vi "高压板校准程序1.2.vi"(8 "波特率":T3(ring)=enum."500Kbps", 9 "CAN路数":u16(ring) items=["0", "1"], 10 "设备索引":u16(ring) items=["0", "1", "2", "3", "4", "5", "6", "7", "8", "9", "10", "11", "12", "13", "14", "15", ""], 11 "CAN卡类型":u32(ring)=21 items=["PCI5121"=1, "PCI9810"=2, "USBCAN1"=3, "USBCAN2"=4, "PCI9820"=5, "PCI5110"=7, "CANLite(mini)"=8, "ISA9620"=9, "ISA5420"=10, "PC104CAN"=11, "DNP9810"=13, "PCI9840B"=14, "PC104C2"=15, "PCI9820I"=16, "pec9920"=18, "USBCAN_E_U"=20, "USBCAN_2E_U"=21]) -> (6 "E-U_baud":u32(ring)=393223 items=["0x060003--1000Kbps"=393219, "0x060004--800Kbps"=393220, "0x060007--500Kbps"=393223, "0x1C0008--250Kbps"=1835016, "0x1C0011--125Kbps"=1835025, "0x160023--100Kbps"=1441827, "0x1C002C--50Kbps"=1835052, "0x1600B3--20Kbps"=1441971, "0x1C00E0--10Kbps"=1835232, "0x1C01C1--5Kbps"=1835457])   [LabVIEW 2013]
uses:
  <vilib>/Instr/_visa.llb/VISA Configure Serial Port (Instr).vi
  <vilib>/Utility/config.llb/Write Key (String).vi
  <vilib>/Utility/file.llb/Read From Spreadsheet File (string).vi
  <vilib>/Utility/file.llb/Write To Spreadsheet File (string).vi
  <vilib>/Utility/config.llb/NI_LVConfig.lvlib
  data/kerneldlls/usbcan.dll
panel:
  out "输出3":dbl
  in  "输出簇":T1
  out "Life":dbl
  out "分流器":enum32{"选项卡 1"}(tab)
  out "外总压":enum32{"选项卡 1"}(tab)
  out "内总压":enum32{"选项卡 1"}(tab)
  out "电流校正 2":enum32{"选项卡 1"}(tab)
  out "电流校正":enum32{"选项卡 1"}(tab)
  in  "Judge(%)":dbl=1.0
  in  "Judge(%)":dbl=0.5
  in  "记录":bool
  out "结果":i32(listbox)=-1
  in  "一键校正":bool
  in  "刷新":bool
  in  "分流器大小":T2(ring)=enum."300A"
  out "监控状态":bool
  out "Curr":dbl format="%#.6f"
  out "SumV_out":dbl format="%#.6f"
  out "SumV_in":dbl format="%#.6f"
  in  "平均电压":dbl
  in  "电压增益":dbl
  in  "平均电流":dbl
  in  "电流增益":dbl
  in  "放电能量阀值":dbl=375.0
  in  "充电能量阀值":dbl=375.0
  in  "分流器型号":bool
  out "Current Gain结果 4":bool
  in  "充电能量阀值":bool
  out "Current Offset结果 4":bool
  in  "Set Current Gain 3":bool
  out "Current Gain结果 3":bool
  in  "Set Current Offset 3":bool
  out "Current Offset结果 3":bool
  out "Shunt Volt Gain":string
  out "Shunt Volt Offset":string
  in  "Set Current Gain 2":bool
  out "Current Gain结果 2":bool
  in  "Volt Offset":bool
  out "Current Offset结果 2":bool
  in  "导入配置结果":bool
  in  "读版本结果":bool
  in  "写版本结果":bool
  out "版本号-读":string
  in  "版本号":string
  in  "写配置文件版本":bool
  in  "读配置文件版本":bool
  in  "生成配置":bool
  in  "导入配置":bool
  out "config_data":string="000124FE00264205"
  out "充放电阈值":dbl=75006.0
  in  "连接状态 10":bool
  in  "设置参数":bool
  in  "安时分辨率/AH":u16(ring)=1 items=["0.001", "0.2"]
  in  "是否有外部高压":u16(ring)=1 items=["有", "无"]
  in  "分流器大小/A":u16(ring)=3 items=["50", "100", "200", "300", "400", "500", "600", "700", "800", "900", "1000"]
  in  "传感器类型":u16(ring)=1 items=["霍尔传感器", "分流器"]
  in  "电压分辨率/V":u16(ring)=1 items=["0.01", "0.1"]
  in  "电流分辨率/A":u16(ring)=1 items=["0.01", "0.1"]
  in  "Set":dbl
  in  "Volt2":dbl=300.0
  in  "Volt1":dbl=150.0
  in  "Clear":bool
  out "Clear结果":bool
  out "电流增益":string
  out "电流零点":string
  in  "Read1_in":bool
  out "Read1_in结果":bool
  in  "REAL1":dbl=150.0
  out "AD1":dbl
  in  "REAL2":dbl=300.0
  out "AD2":dbl
  in  "Offset":i32 format="%x"
  in  "Gain":dbl
  in  "REAL1":dbl=150.0
  in  "AD1":dbl
  in  "REAL2":dbl=300.0
  in  "AD2":dbl
  in  "Offset":i32 format="%x"
  in  "Gain":dbl
  in  "Read2_in":bool
  out "Read2_in结果":bool
  in  "Set_in":bool
  out "Set_in结果":bool
  in  "Read1_Out":bool
  out "Read1_Out结果":bool
  in  "Read2_Out":bool
  out "Read2_Out结果":bool
  in  "Set_out":bool
  out "Set_out结果":bool
  in  "Read1":bool
  out "Read1结果":bool
  in  "REAL1":dbl=40.0
  out "AD1":u16
  in  "REAL2":dbl=80.0
  out "AD2":u16
  in  "Gain":dbl
  in  "Read2":bool
  out "Read2结果":bool
  in  "Set":bool
  out "Set结果":bool
  in  "Set Current Gain":bool
  out "Current Gain结果":bool
  in  "Set Current Offset":bool
  out "Current Offset结果":bool
  in  "Clear_out":bool
  out "Clear_out结果":bool
  in  "Clear_in":bool
  out "Clear_in结果":bool
  in  "输出自定义值1":bool
  in  "输出自定义值2":bool
  out "Actual":dbl format="%#.6f"
  out "Set":dbl format="%#.6f"
  out "Actual":dbl
  in  "连接电压源":bool
  out "连接状态 10":bool
  in  "VISA resource name 4":refnum<visa-resource-name>="COM1" caption="设备端口号"
  in  "工作方式":u8(ring) items=["Normal", "Listen Only"]
  in  "滤波方式":u8(ring) items=["Dual Filter", "Single Filter"]
  out "CAN连接状态":bool
  in  "启动CAN连接":bool
  in  "VISA resource name 2":refnum<visa-resource-name>="GPIB0::5::INSTR" caption="设备端口号"
  out "连接状态 10":bool
  in  "连接GPIB":bool
  in  "Curr1":dbl=40.0
  in  "输出自定义值1 2":bool
  in  "输出自定义值2 2":bool
  in  "Curr2":dbl=80.0
  in  "退出":bool
  out "设置中？ 2":bool
  out "CAN状态 3":bool
  in  "设备索引 3":u16(ring) items=["0", "1", "2", "3", "4", "5", "6", "7", "8", "9", "10", "11", "12", "13", "14", "15", ""]
  in  "CAN路数 3":u16(ring) items=["0", "1"]
  in  "设备类型 3":u16(ring)=4 items=["PCI5121"=1, "PCI9810"=2, "USBCAN1"=3, "USBCAN2"=4, "PCI9820"=5, "CAN232"=6, "PCI5110"=7, "CANLite(mini)"=8, "ISA9620"=9, "ISA5420"=10, "PC104CAN"=11, "CANETE"=12, "DNP9810"=13]
  out "CAN 3":bool
  in  "停止 2":bool=TRUE
  out "监控 4":bool
  out "x-y":u32
  in  "退出程序 2":bool
  in  "error in (no error)":errorcluster caption="错误输入（无错误）"
  in  "控制读取  2":bool
  out "VISA资源名称输出":refnum<visa-resource-name>="0"
  in  "退出程序 3":bool
  in  "输出200A":bool
  out "实际值 2":dbl
  out "设定值 2":dbl
  in  "输出100A":bool
  in  "停止 7":bool=TRUE
  in  "分辨率偏移值 4":T4={"主板总电压分辨率"=0.01, "主板总电压偏移量"=0.0, "主板总电流分辨率"=0.01, "主板总电流偏移量"=-300.0, "主板安时分辨率"=0.2, "主板安时偏移量"=0.0, "主板SOC分辨率"=0.4, "主板SOC偏移量"=0.0, "从板总电压分辨率"=0.01, "从板总电压偏移量"=0.0, "从板总电流分辨率"=0.01, "从板总电流偏移量"=0.0, "从板安时分辨率"=0.2, "从板安时偏移量"=0.0, "从板SOC分辨率"=0.4, "从板SOC偏移量"=0.0, "功率分辨率"=0.01, "功率偏移量"=-300.0, "单体电压分辨率 "=0.0001, "单体电压偏移量"=0.0, "温度分辨率"=1.0, "温度偏移量"=-40.0, "高压板总电压分辨率"=0.01, "高压板总电压偏移量"=0.0, "高压板总电流分辨率"=0.01, "高压板总电流偏移量"=-300.0, "高压板安时分辨率"=0.2, "高压板安时偏移量"=0.0, "高压板SOC分辨率"=0.4, "高压板SOC偏移量"=0.0, "高压板功率分辨率"=0.01, "高压板功率偏移量"=-300.0}
  in  "分辨率偏移值 3":T4={"主板总电压分辨率"=0.01, "主板总电压偏移量"=0.0, "主板总电流分辨率"=0.01, "主板总电流偏移量"=-300.0, "主板安时分辨率"=0.2, "主板安时偏移量"=0.0, "主板SOC分辨率"=0.4, "主板SOC偏移量"=0.0, "从板总电压分辨率"=0.01, "从板总电压偏移量"=0.0, "从板总电流分辨率"=0.01, "从板总电流偏移量"=0.0, "从板安时分辨率"=0.2, "从板安时偏移量"=0.0, "从板SOC分辨率"=0.4, "从板SOC偏移量"=0.0, "功率分辨率"=0.01, "功率偏移量"=-300.0, "单体电压分辨率 "=0.0001, "单体电压偏移量"=0.0, "温度分辨率"=1.0, "温度偏移量"=-40.0, "高压板总电压分辨率"=0.01, "高压板总电压偏移量"=0.0, "高压板总电流分辨率"=0.01, "高压板总电流偏移量"=-300.0, "高压板安时分辨率"=0.2, "高压板安时偏移量"=0.0, "高压板SOC分辨率"=0.4, "高压板SOC偏移量"=0.0, "高压板功率分辨率"=0.01, "高压板功率偏移量"=-300.0}
  in  "监控":bool
  out "VCI_CAN_OBJ_R 2":T5={"ID"=0, "TimeStamp"=0, "TimeFlag"=0, "SendType"=1, "RemoteFlag"=0, "ExternFlag"=0, "DataLen"=8, 0, 0, 0, 0, 0, 0, 0, 0, 0, 0, 0}
  in  "分辨率偏移值":T6
  out "允许读取":bool
  out "设置中？":bool
  out "CAN状态 2":bool=TRUE
  in  "设备索引 2":u16(ring) items=["0", "1", "2", "3", "4", "5", "6", "7", "8", "9", "10", "11", "12", "13", "14", "15", ""]
  in  "CAN路数 2":u16(ring) items=["0", "1"]
  in  "设备类型 2":u16(ring)=4 items=["PCI5121"=1, "PCI9810"=2, "USBCAN1"=3, "USBCAN2"=4, "PCI9820"=5, "CAN232"=6, "PCI5110"=7, "CANLite(mini)"=8, "ISA9620"=9, "ISA5420"=10, "PC104CAN"=11, "CANETE"=12, "DNP9810"=13]
  out "CAN 2":bool
  in  "监控 2":bool
  in  "停止 6":bool=TRUE
  out "接收":T5={"ID"=67239966, "TimeStamp"=241409471, "TimeFlag"=1, "SendType"=250, "RemoteFlag"=0, "ExternFlag"=1, "DataLen"=8, 0, 0, 117, 48, 117, 48, 0, 0, 0, 0, 124} {"ID" format="%x"}
  in  "高压板信息":T7={"内部高压/V"=0.0, "Life"=10.0, "外部高压/V"=0.0, "power/KW"=0.0, "current/A"=0.0, "error code"=1, "SOC/%"=0.0, "总充电安时/AH"=0.0, "总放电安时/AH"=0.0, "平均电压"=0.0} {"平均电压" format="%.3f"; "总放电安时/AH" format="%#.3f"; "总充电安时/AH" format="%#.3f"; "SOC/%" format="%.3g"; "error code" format="%x"; "current/A" format="%.3g"; "power/KW" format="%#.3f"; "外部高压/V" format="%.3g"; "内部高压/V" format="%.3g"}
  in  "控制读取  5":bool
  out "VISA资源名称输出 10":refnum<visa-resource-name>
  in  "输出300V":bool
  out "电流/A 4":dbl
  in  "输出150V":bool
  in  "停止 3":bool=TRUE
  out "error out 3":errorcluster caption="error out"
  in  "错误输入（无错误）":errorcluster
  in  "控制读取  2":bool
  out "VISA资源名称输出 9":refnum<visa-resource-name>
  in  "退出程序":bool
  in  "输出80A":bool
  in  "输出40A":bool
  in  "控制读取  4":bool
  out "VISA资源名称输出 8":refnum<visa-resource-name>
  in  "连接状态 7":bool
  out "error out 2":errorcluster caption="error out"
  in  "控制读取  2":bool
  in  "连接状态 6":bool
  in  "控制读取  3":bool
  out "VISA资源名称输出 6":refnum<visa-resource-name>
  out "error out":errorcluster
  in  "控制读取  2":bool
  out "VISA资源名称输出 5":refnum<visa-resource-name>
  in  "电流值":dbl
  in  "自动控制仪器":bool=TRUE
  out "VISA资源名称输出 4":refnum<visa-resource-name>
  out "VISA资源名称输出 3":refnum<visa-resource-name>
  out "实际值 3":dbl format="%#.6f"
  out "设定值":dbl format="%#.6f"
  in  "控制读取  2":bool
  out "电流/A":dbl
  in  "控制读取":bool
  in  "Boar_Type":bool
  out "temp1":bool
  in  "总步骤":dbl=21.0
  in  "NG重测次数":dbl=3.0
  out "一键测试":bool
  out "测试结果":bool=TRUE
  in  "行号":dbl
  out "CAN状态":bool=TRUE
  out "CAN":bool
  in  "监控":bool=TRUE
  out "VCI_CAN_OBJ_R":T5={"ID"=0, "TimeStamp"=0, "TimeFlag"=0, "SendType"=1, "RemoteFlag"=0, "ExternFlag"=0, "DataLen"=8, 0, 0, 0, 0, 0, 0, 0, 0, 0, 0, 0}
  in  "停止":bool=TRUE
  # "重要参数设置"
  # "A"
  # "V"
  # "蓝微新源BMS_电压电流校准"
  # "内总压"
  # "电流增益"
  # "AD2=AD1*2"
  # "外总压"
  # "BMS_Monitor"
  # "分辩率"
  # "偏移量"
  # "分辩率"
  # "偏移量"
  # "分辩率"
  # "偏移量"
  # "分辩率"
  # "偏移量"
  # "分辩率"
  # "偏移量"
  # "分辩率"
  # "偏移量"
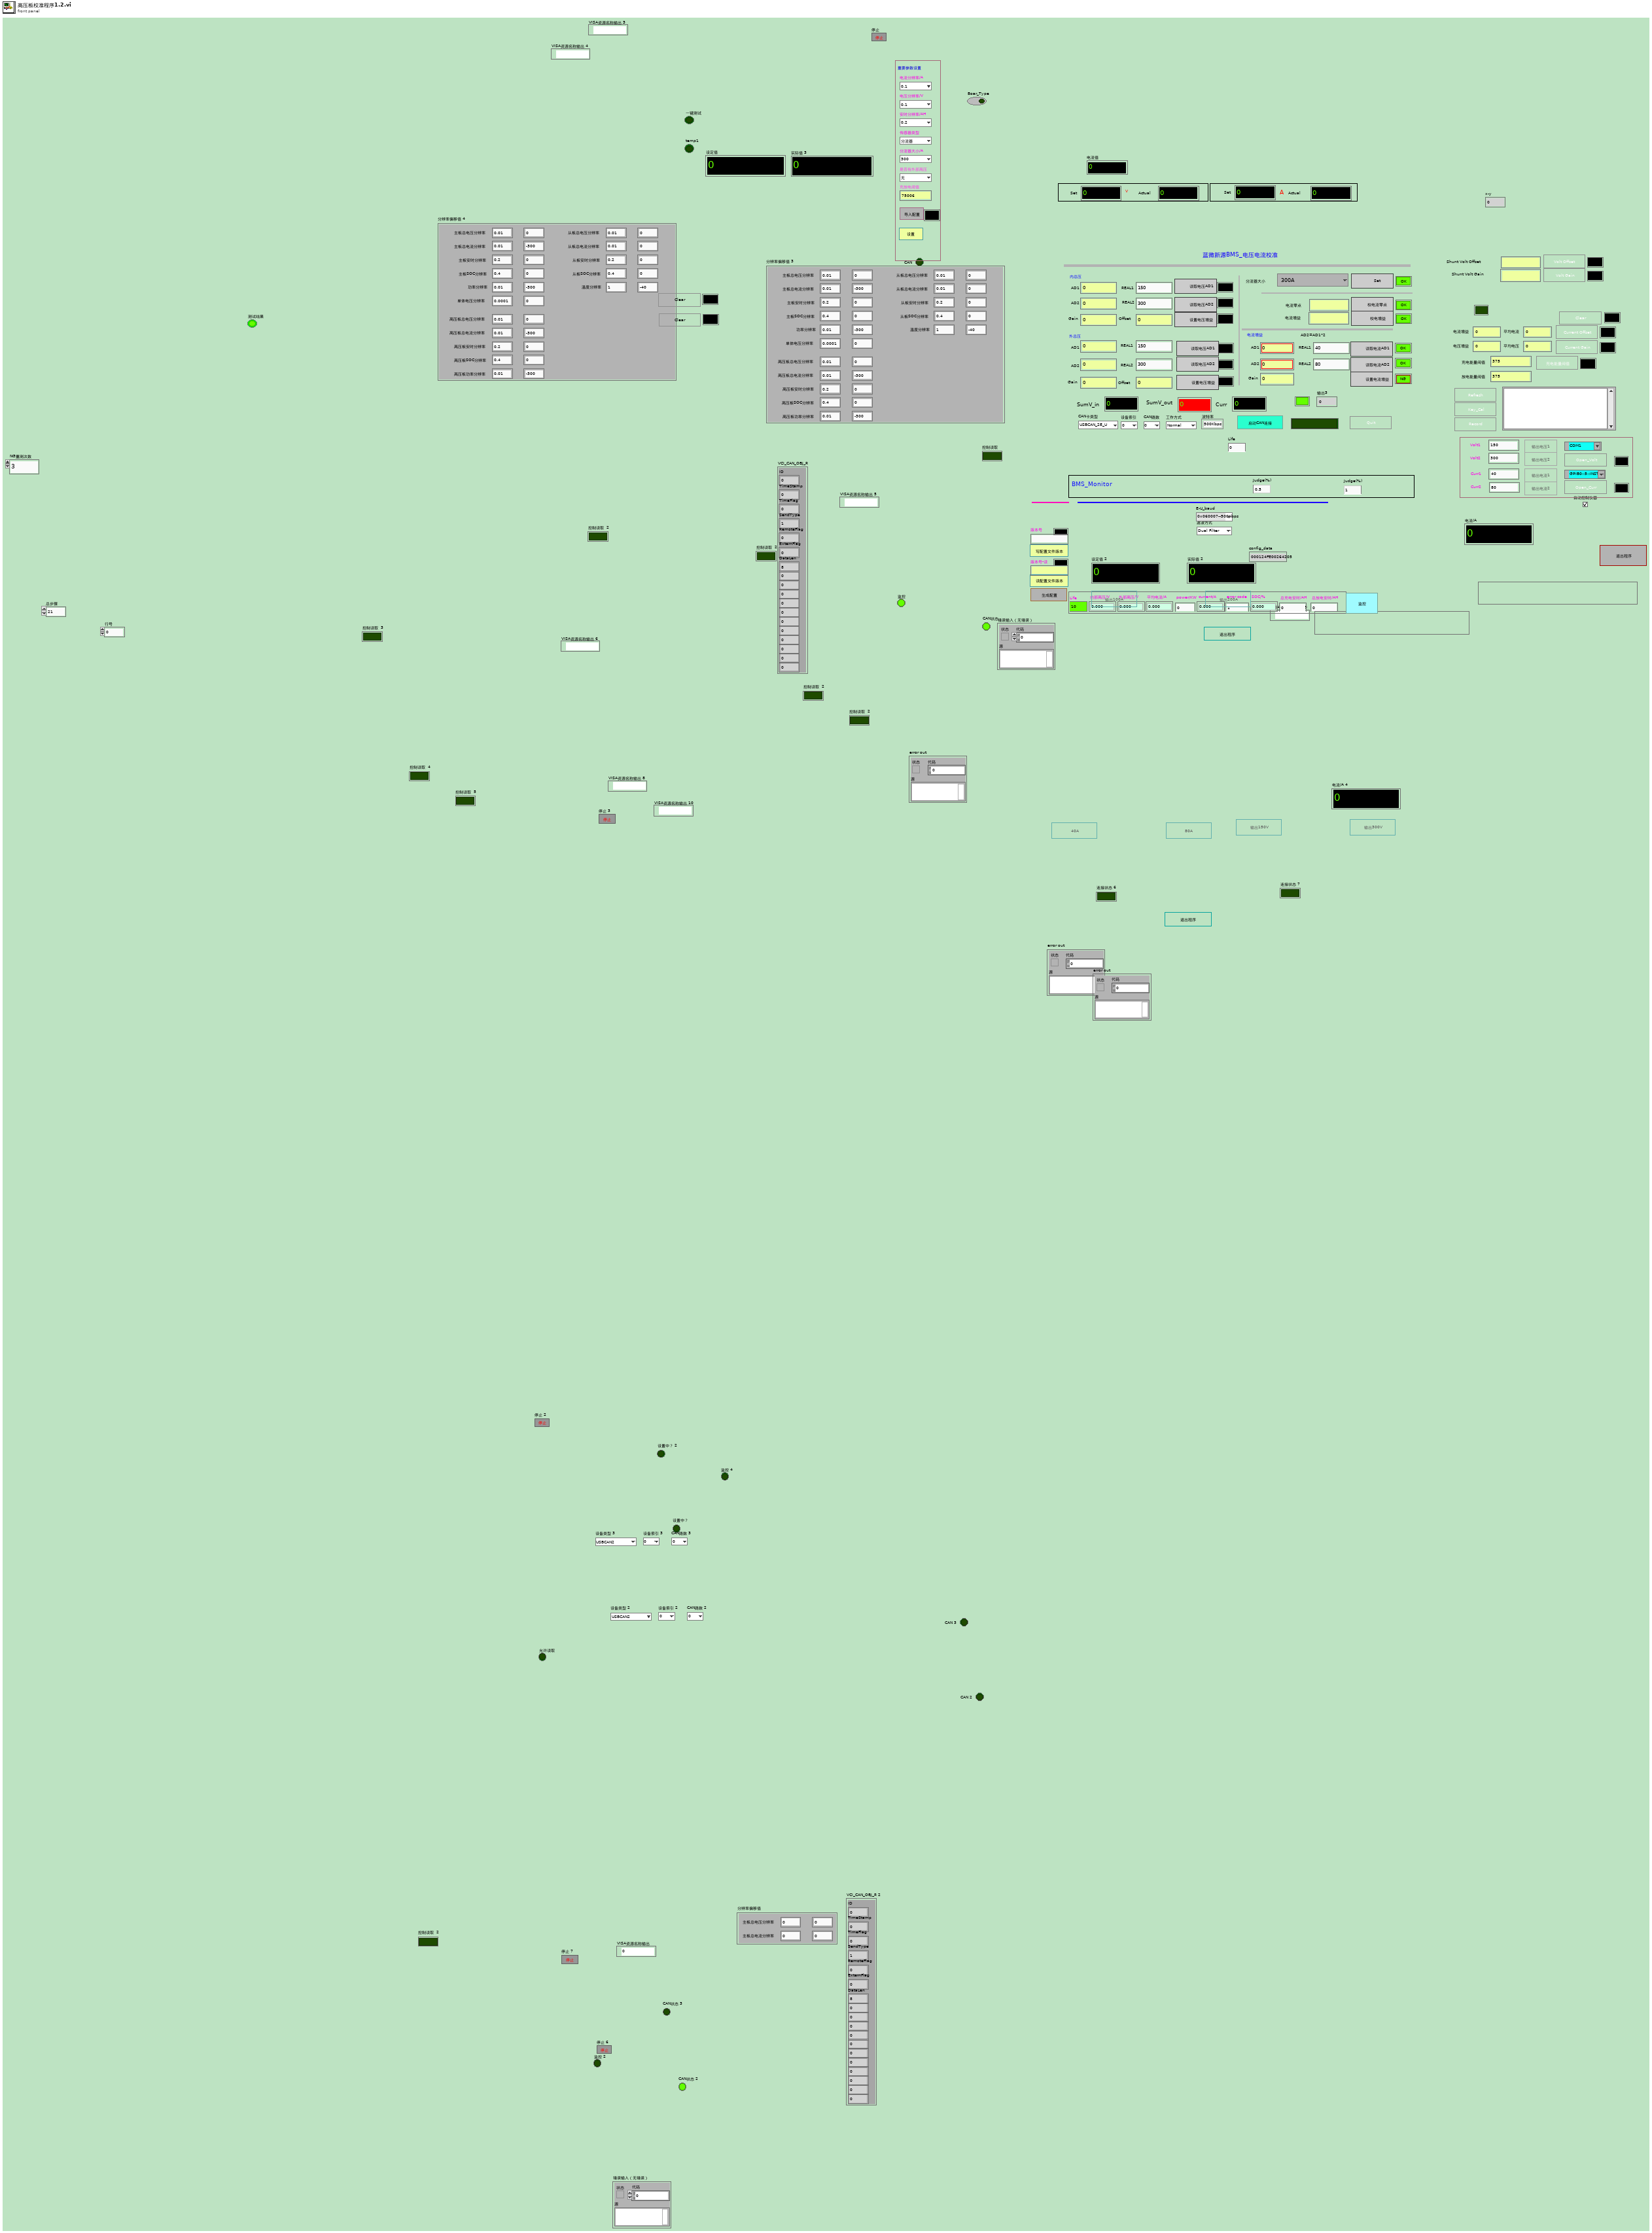
[diagram p1: front panel]
types:
  T1 = cluster{"return type":u32, "pReceive":cluster{"ID":u32, "TimeStamp":u32, "TimeFlag":u8, "SendType":u8, "RemoteFlag":u8, "ExternFlag":u8, "DataLen":u8, u8, u8, u8, u8, u8, u8, u8, u8, u8, u8, u8}[]}
  T2 = enum16{"选择分流器型号", "100A", "200A", "300A", "400A", "500A", "600A", "700A", "800A", "900A", "1000A"}
  T3 = enum16{"5Kbps", "10Kbps", "20Kbps", "40Kbps", "50Kbps", "80Kbps", "100Kbps", "125Kbps", "200Kbps", "250Kbps", "400Kbps", "500Kbps", "666Kbps", "800Kbps", "1000Kbps"}
  T4 = cluster{"主板总电压分辨率":dbl, "主板总电压偏移量":dbl, "主板总电流分辨率":dbl, "主板总电流偏移量":dbl, "主板安时分辨率":dbl, "主板安时偏移量":dbl, "主板SOC分辨率":dbl, "主板SOC偏移量":dbl, "从板总电压分辨率":dbl, "从板总电压偏移量":dbl, "从板总电流分辨率":dbl, "从板总电流偏移量":dbl, "从板安时分辨率":dbl, "从板安时偏移量":dbl, "从板SOC分辨率":dbl, "从板SOC偏移量":dbl, "功率分辨率":dbl, "功率偏移量":dbl, "单体电压分辨率 ":dbl, "单体电压偏移量":dbl, "温度分辨率":dbl, "温度偏移量":dbl, "高压板总电压分辨率":dbl, "高压板总电压偏移量":dbl, "高压板总电流分辨率":dbl, "高压板总电流偏移量":dbl, "高压板安时分辨率":dbl, "高压板安时偏移量":dbl, "高压板SOC分辨率":dbl, "高压板SOC偏移量":dbl, "高压板功率分辨率":dbl, "高压板功率偏移量":dbl}
  T5 = cluster{"ID":u32, "TimeStamp":u32, "TimeFlag":u8, "SendType":u8, "RemoteFlag":u8, "ExternFlag":u8, "DataLen":u8, u8, u8, u8, u8, u8, u8, u8, u8, u8, u8, u8}
  T6 = cluster{"主板总电压分辨率":dbl, "主板总电压偏移量":dbl, "主板总电流分辨率":dbl, "主板总电流偏移量":dbl, "主板安时分辨率":dbl, "主板安时偏移量":dbl, "主板SOC分辨率":dbl, "主板SOC偏移量":dbl, "从板总电压分辨率":dbl, "从板总电压偏移量":dbl, "从板总电流分辨率":dbl, "从板总电流偏移量":dbl, "从板安时分辨率":dbl, "从板安时偏移量":dbl, "从板SOC分辨率":dbl, "从板SOC偏移量":dbl, "功率分辨率":dbl, "功率偏移量":dbl, "单体电压分辨率 ":dbl, "单体电压偏移量":dbl, "温度分辨率":dbl, "温度偏移量":dbl}
  T7 = cluster{"内部高压/V":dbl, "Life":dbl, "外部高压/V":dbl, "power/KW":dbl, "current/A":dbl, "error code":u32, "SOC/%":dbl, "总充电安时/AH":dbl, "总放电安时/AH":dbl, "平均电压":dbl}
  T8 = enum16{"Set Current Offset", "Set Current Gain 4", "Set Current Gain", "Set Volt offset", "Set Volt Gain", "Set Current Offset 3", "Set Current Gain 3", "Set Current Offset 4", "Read", "Set", "Clear", "Read_in", "Set_in", "Clear_in", "Read_out", "Set_out", "Clear_out", "参数设置", "写配置文件版本", "读配置文件版本"}
  T9 = enum16{"Set Current Offset", "Set Current Gain", "Read", "Set", "Clear", "Read_in", "Set_in", "Clear_in", "Read_out", "Set_out", "Clear_out", "参数设置", "写配置文件版本", "读配置文件版本"}
  T10 = enum16{"Set Current Offset", "Set Current Gain", "Read", "Set", "Clear", "Read_in", "Set_in", "Clear_in", "Read_out", "Set_out", "Clear_out"}
  T11 = cluster{"ID":u32, "TimeStamp":u32, "TimeFlag":u8, "SendType":u8, "RemoteFlag":u8, "ExternFlag":u8, "DataLen":u8, u8, u8, u8, u8, u8, u8, u8, u8, u8, u8, u8}[]
  T12 = enum32{"Invalid", "Standard", "Closed", "Hidden", "Minimized", "Maximized"}
  T13 = typedef "NI_LVConfig.lvlib/Config Data RefNum.ctl" = refnum<k1>
  T14 = cluster{"return type":u32, "pReceive":cluster{"ID":u32, "TimeStamp":u32, "TimeFlag":u8, "SendType":u8, "RemoteFlag":u8, "ExternFlag":u8, "DataLen":u8, "1":u8, "2":u8, "3":u8, "4":u8, "5":u8, "6":u8, "7":u8, "8":u8, "9":u8, "10":u8, "11":u8}[]}
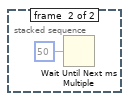
[diagram p2: hidden frame]
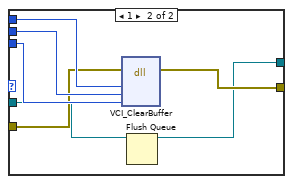
[diagram p4: hidden frame]
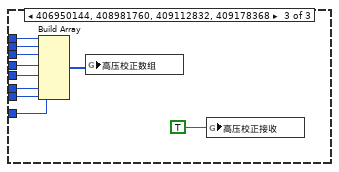
[diagram p7: hidden frame]
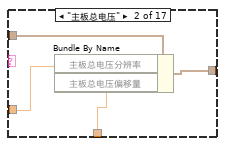
[diagram p10: hidden frame]
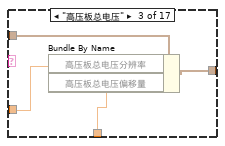
[diagram p11: hidden frame]
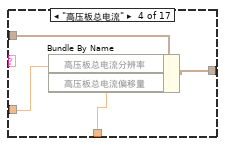
[diagram p12: hidden frame]
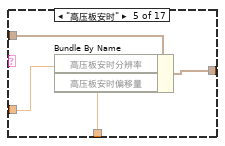
[diagram p13: hidden frame]
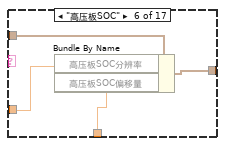
[diagram p14: hidden frame]
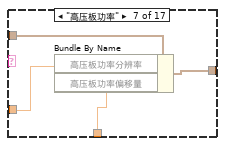
[diagram p15: hidden frame]
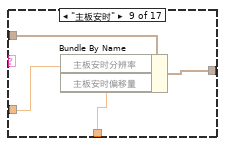
[diagram p16: hidden frame]
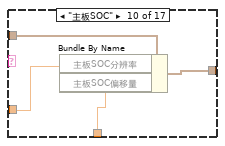
[diagram p17: hidden frame]
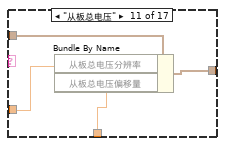
[diagram p18: hidden frame]
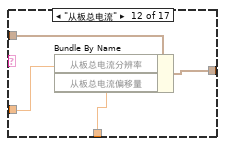
[diagram p19: hidden frame]
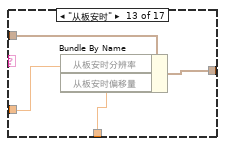
[diagram p20: hidden frame]
diagram:
  w19 = u32 0
  w36 = FALSE ("停止")
  w40 = u16 1 items=["霍尔传感器", "分流器"] ("传感器类型")
  w38 = cluster{u32, u32}[] [{0, 0}] ("颜色[4]")
  w37 = "" ("布尔文本.文本")
  w51 = u8 2 ("禁用")
  w47 = 0.0 ("电流/A")
  (unwired) "SET:GRO 1,10,1,1,0,0,0" ("写入缓冲区")
  w62 = u8 2 ("禁用")
  w46 = u8 2 ("禁用")
  (unwired) "SET:GRO 1,10,1,1,0,0,0" ("写入缓冲区")
  w69 = u8 0 ("禁用")
  w25 = cluster{u32, u32}[] [{0, 0}] ("颜色[4]")
  w24 = "" ("布尔文本.文本")
  (unwired) u8 2 ("禁用")
  (unwired) 20
  (unwired) u8 2 ("禁用")
  w70 = "Cmd" ("名称（未命名）")
  n1 = disable-structure shown="禁用" {
    frame Disabled {
      n2 = call "getpath.vi"() -> ("stripped path"=w78:path)  [unwired: 11 out]
      n3 = local read "分辨率偏移值 3"() -> (w75:T4)
      n4 = Build Path(base path=w78, name or relative path="Settings\\300以下分辨率偏移值.xls" ("名称或相对路径")) -> (appended path=w82:path)
      n5 = call-poly <vilib>:"Read From Spreadsheet File.vi"("file path (dialog if empty)"=w82) -> ("all rows"=w79:string[][])  [unwired: 3 in, 7 out]
      n6 = Delete From Array(array=w79, length=1 ("长度"), index (row)=0 ("索引")) -> (array with subset deleted=w76:string[][])  [unwired: 1 in, 1 out]
      n7 = for {
        tunnel: w76 -> [w91] mode=indexing
        shift-right: [w83] -> w74
        shift-left: w75 -> [w88]
        n8 = Index Array(array=w91, index #1=0 ("索引")) -> (element #1=w89:string, element #2=w87:string, element #3=w85:string)  [unwired: 2 in]
        n9 = Fract/Exp String To Number(string=w87) -> (number=w86:dbl)  [unwired: 4 out]
        n10 = Fract/Exp String To Number(string=w85) -> (number=w84:dbl)  [unwired: 4 out]
        n11 = case shown="\"主板总电流\"" w89 {
          tunnel: w88 -> [w92 w96 w100 w104 w108 w112 w116 w120 w124 w128 w132 w136 w140 w144 w148 w152 w156]
          tunnel: [w92 w95 w99 w103 w107 w111 w115 w119 w123 w127 w131 w135 w139 w143 w147 w151 w155] -> w83
          tunnel: w86 -> [_ w94 w98 w102 w106 w110 w114 w118 w122 w126 w130 w134 w138 w142 w146 w150 w154]
          tunnel: w84 -> [_ w93 w97 w101 w105 w109 w113 w117 w121 w125 w129 w133 w137 w141 w145 w149 w153]
          frame "假", Default {
          }
          frame "主板总电压" {
            n12 = Bundle By Name(cluster=w96, "主板总电压分辨率"=w94, "主板总电压偏移量"=w93) -> (w95:T4)
          }
          frame "高压板总电压" {
            n13 = Bundle By Name(cluster=w100, "高压板总电压分辨率"=w98, "高压板总电压偏移量"=w97) -> (w99:T4)
          }
          frame "高压板总电流" {
            n14 = Bundle By Name(cluster=w104, "高压板总电流分辨率"=w102, "高压板总电流偏移量"=w101) -> (w103:T4)
          }
          frame "高压板安时" {
            n15 = Bundle By Name(cluster=w108, "高压板安时分辨率"=w106, "高压板安时偏移量"=w105) -> (w107:T4)
          }
          frame "高压板SOC" {
            n16 = Bundle By Name(cluster=w112, "高压板SOC分辨率"=w110, "高压板SOC偏移量"=w109) -> (w111:T4)
          }
          frame "高压板功率" {
            n17 = Bundle By Name(cluster=w116, "高压板功率分辨率"=w114, "高压板功率偏移量"=w113) -> (w115:T4)
          }
          frame "主板总电流" {
            n18 = Bundle By Name(cluster=w120, "主板总电流分辨率"=w118, "主板总电流偏移量"=w117) -> (w119:T4)
          }
          frame "主板安时" {
            n19 = Bundle By Name(cluster=w124, "主板安时分辨率"=w122, "主板安时偏移量"=w121) -> (w123:T4)
          }
          frame "主板SOC" {
            n20 = Bundle By Name(cluster=w128, "主板SOC分辨率"=w126, "主板SOC偏移量"=w125) -> (w127:T4)
          }
          frame "从板总电压" {
            n21 = Bundle By Name(cluster=w132, "从板总电压分辨率"=w130, "从板总电压偏移量"=w129) -> (w131:T4)
          }
          frame "从板总电流" {
            n22 = Bundle By Name(cluster=w136, "从板总电流分辨率"=w134, "从板总电流偏移量"=w133) -> (w135:T4)
          }
          frame "从板安时" {
            n23 = Bundle By Name(cluster=w140, "从板安时分辨率"=w138, "从板安时偏移量"=w137) -> (w139:T4)
          }
          frame "从板SOC" {
            n24 = Bundle By Name(cluster=w144, "从板SOC分辨率"=w142, "从板SOC偏移量"=w141) -> (w143:T4)
          }
          frame "温度" {
            n25 = Bundle By Name(cluster=w148, "温度分辨率"=w146, "温度偏移量"=w145) -> (w147:T4)
          }
          frame "功率" {
            n26 = Bundle By Name(cluster=w152, "功率分辨率"=w150, "功率偏移量"=w149) -> (w151:T4)
          }
          frame "单体电压" {
            n27 = Bundle By Name(cluster=w156, "单体电压分辨率"=w154, "单体电压偏移量"=w153) -> (w155:T4)
          }
        }
      }
      n28 = local write "分辨率偏移值 3"(w74) -> ()
    }
    frame Enabled {
    }
  }
  n29 = disable-structure shown="禁用" {
    disable-tunnel: [w157 _] -> w20
    frame Disabled {
      n30 = stacked-sequence {
        tunnel: [w159 _] -> w157
        frame #0 {
          n31 = global read "EV05全局变量1.vi" "设备索引号"() -> (w161:u16)
          n32 = global read "EV05全局变量1.vi" "CAN卡类型"() -> (w162:u32)
          n33 = global read "EV05全局变量1.vi" "CAN端口"() -> (w160:u16)
          n34 = Build Array(1) -> (w163:i32[])
          n35 = call "transmit-8.6.vi"("can卡类型"=w162, "设备索引号"=w161, "CAN端口"=w160, "ID"=418398080, "SendType"=u8 0, "Data"=w163) -> ("错误输出"=w159:errorcluster)  [unwired: 3 in, 10 out]
        }
        frame #1 {
          n36 = Wait Until Next ms Multiple(millisecond multiple=u32 50 ("毫秒倍数")) -> ()  [unwired: 1 out]
        }
      }
    }
    frame Enabled {
    }
  }
  n37 = disable-structure shown="禁用" {
    frame Disabled {
      w173 = "MOSHI" ("section")
      n38 = call "getpath.vi"() -> ("stripped path"=w177:path)  [unwired: 11 out]
      n39 = Build Path(base path=w177, name or relative path="Settings\\EV03.ini" ("名称或相对路径")) -> (appended path=w175:path)
      n40 = call "Read&Write ini.vi"("功能"=enum16{"读取配置", "写入配置"}."读取配置", "configuration file path"=w175, "section"=w173, "key"=w173) -> ("key 4"=w172:string)  [unwired: 1 in, 10 out]
      n41 = Equal?(x=w172, y="1") -> (x = y?=w170:bool)
      n42 = Select(t=u8 0 ("禁用"), s=w170, f=u8 1 ("禁用")) -> (s? t:f=w167:u8)
      n43 = property on="电流分辨率/A" class="Ring (严格)"("Disabled"=w167) -> ()  [unwired: 2 in, 2 out]
      n44 = property on="电压分辨率/V" class="Ring (严格)"("Disabled"=w167) -> ()  [unwired: 2 in, 2 out]
      n45 = property on="是否有外部高压" class="Ring (严格)"("Disabled"=w167) -> ()  [unwired: 2 in, 2 out]
      n46 = property on="充放电阈值" class="DigNum (严格)"("Disabled"=w167) -> ()  [unwired: 2 in, 2 out]
      n47 = property on="传感器类型" class="Ring (严格)"("Disabled"=w167) -> ()  [unwired: 2 in, 2 out]
      n48 = property on="分流器大小/A" class="Ring (严格)"("Disabled"=w167) -> ()  [unwired: 2 in, 2 out]
      n49 = property on="安时分辨率/AH" class="Ring (严格)"("Disabled"=w167) -> ()  [unwired: 2 in, 2 out]
      n50 = property on="版本号" class="Str"("Disabled"=w167) -> ()  [unwired: 2 in, 2 out]
    }
    frame Enabled {
    }
  }
  n51 = local write "连接状态 10"(FALSE ("连接状态")) -> ()
  n52 = property on="输出150V" class="Bool"("Disabled"=w62) -> ()  [unwired: 2 in, 2 out]
  n53 = property on="输出300V" class="Bool"("Disabled"=w62) -> ()  [unwired: 2 in, 2 out]
  n54 = property on="输出自定义值2" class="Bool"("Disabled"=w62) -> ()  [unwired: 2 in, 2 out]
  n55 = property on="输出自定义值1" class="Bool"("Disabled"=w62) -> ()  [unwired: 2 in, 2 out]
  n56 = local write "VISA resource name 2"("GPIB0::5::INSTR" ("写入缓冲区")) -> ()
  n57 = local write "VISA资源名称输出 9"("" ("写入缓冲区")) -> ()
  n58 = local write "连接状态 10"(FALSE ("连接状态")) -> ()
  n59 = global read "EV05全局变量1.vi" "分流器型号"() -> (w2:T2)
  n60 = local write "连接状态 10"(FALSE ("设置_结果")) -> ()
  n61 = property on="Set_out" class="Bool (严格)"("Disabled"=w69) -> ()  [unwired: 2 in, 2 out]
  n62 = property on="Clear_in" class="Bool (严格)"("Disabled"=w69) -> ()  [unwired: 2 in, 2 out]
  n63 = property on="Set_in" class="Bool (严格)"("Disabled"=w69) -> ()  [unwired: 2 in, 2 out]
  n64 = local write "连接状态 10"(FALSE ("连接状态")) -> ()
  n65 = property on="Read2_Out" class="Bool (严格)"("Disabled"=w69) -> ()  [unwired: 2 in, 2 out]
  n66 = property on="Clear" class="Bool (严格)"("Disabled"=w69) -> ()  [unwired: 2 in, 2 out]
  n67 = local write "退出"(FALSE ("退出")) -> ()
  n68 = property on="输出40A" class="Bool"("Disabled"=w46) -> ()  [unwired: 2 in, 2 out]
  n69 = property on="输出80A" class="Bool"("Disabled"=w46) -> ()  [unwired: 2 in, 2 out]
  n70 = local write "NG重测次数"(3.0 ("NG重测次数")) -> ()
  n71 = property on="Read1_Out" class="Bool (严格)"("Disabled"=w69) -> ()  [unwired: 2 in, 2 out]
  n72 = property on="输出100A" class="Bool"("Disabled"=w51) -> ()  [unwired: 2 in, 2 out]
  n73 = property on="输出200A" class="Bool"("Disabled"=w51) -> ()  [unwired: 2 in, 2 out]
  n74 = property on="输出自定义值2 2" class="Bool"("Disabled"=w51) -> ()  [unwired: 2 in, 2 out]
  n75 = property on="输出自定义值1 2" class="Bool"("Disabled"=w51) -> ()  [unwired: 2 in, 2 out]
  n76 = property on="Set Current Gain" class="Bool (严格)"("Disabled"=w69) -> ()  [unwired: 2 in, 2 out]
  n77 = property on="Set Current Offset" class="Bool (严格)"("Disabled"=w69) -> ()  [unwired: 2 in, 2 out]
  n78 = property on="Read1_in" class="Bool (严格)"("Disabled"=w69) -> ()  [unwired: 2 in, 2 out]
  n79 = property on="Clear_out" class="Bool (严格)"("Disabled"=w69) -> ()  [unwired: 2 in, 2 out]
  n80 = local write "分流器大小"(w2) -> ()
  n81 = local write "Actual"(w47) -> ()
  n82 = global read "EV05全局变量1.vi" "设备索引号"() -> (w33:u16)
  n83 = global read "EV05全局变量1.vi" "CAN卡类型"() -> (w34:u32)
  n84 = local write "连接状态 10"(FALSE ("连接状态")) -> ()
  n85 = global read "EV05全局变量1.vi" "CAN端口"() -> (w35:u16)
  n86 = property on="Read2_in" class="Bool (严格)"("Disabled"=w69) -> ()  [unwired: 2 in, 2 out]
  n87 = global read "EV05全局变量1.vi" "波特率"() -> (w1:u16)
  n88 = property on="Set" class="Bool (严格)"("Disabled"=w69) -> ()  [unwired: 2 in, 2 out]
  n89 = property on="Read2" class="Bool (严格)"("Disabled"=w69) -> ()  [unwired: 2 in, 2 out]
  n90 = local write "Set"(w47) -> ()
  n91 = property on="Read1" class="Bool (严格)"("Disabled"=w69) -> ()  [unwired: 2 in, 2 out]
  n92 = local write "Curr1"(40.0 ("电流1（A）")) -> ()
  n93 = local write "Curr2"(80.0 ("电流2（A）")) -> ()
  n94 = local write "Volt1"(150.0 ("电压1 4")) -> ()
  n95 = local write "Volt2"(300.0 ("电压2 5")) -> ()
  n96 = local write "CAN卡类型"(w34) -> ()
  n97 = local write "CAN路数"(w35) -> ()
  n98 = local write "设备索引"(w33) -> ()
  n99 = local write "波特率"(w1) -> ()
  n100 = Obtain Queue(name (unnamed)="CAN" ("名称（未命名）"), element data type="输出簇", error in (no error)="error in (no error)") -> (queue out=w8:refnum<queue>, error out=w42:errorcluster)  [unwired: 2 in, 1 out]
  n101 = local write "VISA资源名称输出"("0" ("写入缓冲区")) -> ()
  n102 = property on="读版本结果" class="Bool (严格)"("Colors [4]"=w38, "BoolText.Text"=w37) -> ()  [unwired: 2 in, 2 out]
  n103 = property on="写版本结果" class="Bool (严格)"("Colors [4]"=w38, "BoolText.Text"=w37) -> ()  [unwired: 2 in, 2 out]
  n104 = property on="导入配置结果" class="Bool (严格)"("Colors [4]"=w38, "BoolText.Text"=w37) -> ()  [unwired: 2 in, 2 out]
  n105 = property on="连接状态 10" class="Bool (严格)"("Colors [4]"=w38, "BoolText.Text"=w37) -> ()  [unwired: 2 in, 2 out]
  n106 = local write "版本号"("" ("版本号")) -> ()
  n107 = invoke on="监控" class="Bool" method="Reinit To Default"() -> ()  [unwired: 3 in, 3 out]
  n108 = local write "监控 2"(FALSE ("监控 2")) -> ()
  n109 = local write "传感器类型"(w40) -> ()
  n110 = Obtain Queue(name (unnamed)=w70, element data type=w70) -> (queue out=w45:refnum<queue>, error out=w44:errorcluster)  [unwired: 3 in, 1 out]
  n111 = while {
    tunnel: [w213] -> _
    tunnel: w20 -> [_]
    stop <- "停止 3" stop-if-true
    n112 = local read "连接状态 10"() -> (w216:bool)
    n113 = local read "控制读取  5"() -> (w217:bool)
    n114 = local read "Judge(%)"() -> (w212:dbl)
    n115 = local read "SumV_out"() -> (w205:dbl)
    n116 = local read "SumV_in"() -> (w207:dbl)
    n117 = local read "Actual"() -> (w200:dbl)
    n118 = And(x=w216, y=w217) -> (x .and. y?=w215:bool)
    n119 = case shown="真" w215 {
      tunnel: [_ w220] -> w214
      frame False {
      }
      frame True {
        n120 = local read "VISA资源名称输出 10"() -> (w237:refnum<visa-resource-name>)
        n121 = Concatenate Strings("MEA:ALL?" ("写入缓冲区"), "\n") -> (w234:string)
        n122 = VISA Write(VISA resource name=w237, write buffer=w234) -> (VISA resource name out=w236:refnum<visa-resource-name>, error out=w232:errorcluster)  [unwired: 1 in, 1 out]
        n123 = flat-sequence {
          tunnel: w236 -> [w240]
          tunnel: [w240] -> w231
          tunnel: [w238] -> w230
          tunnel: w232 -> [w238]
          tunnel: [w245] -> w229
          tunnel: [w244] -> w228
          tunnel: w231 -> [w243]
          tunnel: w230 -> [w242]
          tunnel: [w241] -> w227
          frame #0 {
            n124 = Wait (ms)(milliseconds to wait=u32 50 ("等待时间（毫秒）")) -> ()  [unwired: 1 out]
          }
          frame #1 {
            n125 = property class="Instr"(reference=w243, error in=w242) -> (reference out=w245:refnum<visa-resource-name>, error out=w241:errorcluster, "Serial Settings:Number of Bytes at Serial Port"=w244:u32)
          }
        }
        n126 = VISA Read(VISA resource name=w229, byte count=w228, error in (no error)=w227) -> (read buffer=w226:string, error out=w220:errorcluster)  [unwired: 2 out]
        n127 = Match Pattern(string=w226, regular expression="," ("正则表达式")) -> (before substring=w223:string, after substring=w224:string)  [unwired: 3 out]
        n128 = Fract/Exp String To Number(string=w223) -> (number=w222:dbl)  [unwired: 4 out]
        n129 = Fract/Exp String To Number(string=w224) -> (number=w221:dbl)  [unwired: 4 out]
        n130 = local write "电流/A 4"(w221) -> ()
        n131 = local write "Actual"(w222) -> ()
      }
    }
    n132 = Divide(x=w212, y=100.0) -> (x/y=w208:dbl)
    n133 = Add(x=1.0, y=w208) -> (x+y=w204:dbl)
    n134 = Subtract(x=1.0, y=w208) -> (x-y=w206:dbl)
    n135 = Multiply(x=w204, y=w200) -> (x*y=w194:dbl)
    n136 = Multiply(x=w206, y=w200) -> (x*y=w193:dbl)
    n137 = In Range and Coerce(upper limit=w194, x=w207, lower limit=w193) -> (In Range?=w203:bool)  [unwired: 1 out]
    n138 = In Range and Coerce(upper limit=w194, x=w205, lower limit=w193) -> (In Range?=w196:bool)  [unwired: 1 out]
    n139 = Select(t=u32 0, s=w203, f=u32 16711680) -> (s? t:f=w199:u32)
    n140 = Select(t=u32 0, s=w196, f=u32 16711680) -> (s? t:f=w195:u32)
    n141 = property on="SumV_in" class="DigNum (严格)"("NumText.BGColor"=w199) -> ()  [unwired: 2 in, 2 out]
    n142 = property on="SumV_out" class="DigNum (严格)"("NumText.BGColor"=w195) -> ()  [unwired: 2 in, 2 out]
    n143 = local read "Judge(%)"() -> (w187:dbl)
    n144 = local read "Actual"() -> (w188:dbl)
    n145 = Divide(x=w187, y=100.0) -> (x/y=w178:dbl)
    n146 = local read "Curr"() -> (w182:dbl)
    n147 = Subtract(x=1.0, y=w178) -> (x-y=w190:dbl)
    n148 = Add(x=1.0, y=w178) -> (x+y=w192:dbl)
    n149 = Multiply(x=w190, y=w188) -> (x*y=w180:dbl)
    n150 = Multiply(x=w192, y=w188) -> (x*y=w181:dbl)
    n151 = In Range and Coerce(upper limit=w181, x=w182, lower limit=w180) -> (In Range?=w185:bool)  [unwired: 1 out]
    n152 = Wait (ms)(milliseconds to wait=u32 50 ("等待时间（毫秒）")) -> ()  [unwired: 1 out]
    n153 = Select(t=u32 0, s=w185, f=u32 16711680) -> (s? t:f=w179:u32)
    n154 = property on="Curr" class="DigNum (严格)"("NumText.BGColor"=w179) -> ()  [unwired: 2 in, 2 out]
    n155 = call <vilib>:"Clear Errors.vi"("error in (no error)"=w214) -> ("error out"=w213:errorcluster)  [unwired: 6 out]
  }
  n156 = while {
    tunnel: w45 -> [w248]
    tunnel: w44 -> [w247]
    tunnel: w20 -> [_]
    stop <- w246 stop-if-true
    n157 = Dequeue Element(queue=w248, error in (no error)=w247) -> (queue out=w249:refnum<queue>, element=w250:string, error out=w246:errorcluster)  [unwired: 2 out]
    n158 = case shown="无错误" w246 {
      tunnel: w250 -> [w253 _]
      tunnel: w249 -> [w252 _]
      tunnel: w246 -> [w251 _]
      frame No Error {
        n159 = while {
          tunnel: w253 -> [w280]
          tunnel: w251 -> [_]
          tunnel: w252 -> [_]
          i -> [w278]
          stop <- w276 stop-if-true
          n160 = case shown="\"Set Current Gain 4\"" w280 {
            selector: w280 -> [w921 w925 w929 w933 w937 w943 w947 w951 w955 w959 w963 w967 w973 w979 w982 w986 w992 w998 w1002 w1006 w1010 w1014 w1024 w1034]
            tunnel: ["" ("转换结果") "00" ("产品编号") "00" ("产品编号") "00" ("产品编号") "00" ("产品编号") w939 "00" ("产品编号") "00" ("产品编号") "00" ("产品编号") "00" ("产品编号") "00" ("产品编号") "00" ("产品编号") w969 w975 "2710" ("产品编号") w984 w989 w994 "000100000000" ("产品编号") "000100000000" ("产品编号") "00" ("产品编号") "00" ("产品编号") w1016 w1028] -> w274
            tunnel: [w921 w925 w929 w933 w937 w943 w947 w951 w955 w959 w963 w967 w973 w979 w982 w986 w992 w998 w1002 w1006 w1010 w1014 w1024 w1034] -> w281
            tunnel: [enum16{"ASCII字符", "16进制字符"}."ASCII字符" ("传入类型") enum16{"ASCII字符", "16进制字符"}."16进制字符" ("传入类型") enum16{"ASCII字符", "16进制字符"}."16进制字符" ("传入类型") enum16{"ASCII字符", "16进制字符"}."16进制字符" ("传入类型") enum16{"ASCII字符", "16进制字符"}."16进制字符" ("传入类型") enum16{"ASCII字符", "16进制字符"}."16进制字符" ("传入类型") enum16{"ASCII字符", "16进制字符"}."16进制字符" ("传入类型") enum16{"ASCII字符", "16进制字符"}."16进制字符" ("传入类型") enum16{"ASCII字符", "16进制字符"}."16进制字符" ("传入类型") enum16{"ASCII字符", "16进制字符"}."16进制字符" ("传入类型") enum16{"ASCII字符", "16进制字符"}."16进制字符" ("传入类型") enum16{"ASCII字符", "16进制字符"}."16进制字符" ("传入类型") enum16{"ASCII字符", "16进制字符"}."16进制字符" ("传入类型") enum16{"ASCII字符", "16进制字符"}."16进制字符" ("传入类型") enum16{"ASCII字符", "16进制字符"}."16进制字符" ("传入类型") enum16{"ASCII字符", "16进制字符"}."16进制字符" ("传入类型") enum16{"ASCII字符", "16进制字符"}."ASCII字符" ("传入类型") enum16{"ASCII字符", "16进制字符"}."ASCII字符" ("传入类型") enum16{"ASCII字符", "16进制字符"}."16进制字符" ("传入类型") enum16{"ASCII字符", "16进制字符"}."16进制字符" ("传入类型") enum16{"ASCII字符", "16进制字符"}."16进制字符" ("传入类型") enum16{"ASCII字符", "16进制字符"}."16进制字符" ("传入类型") enum16{"ASCII字符", "16进制字符"}."16进制字符" ("传入类型") enum16{"ASCII字符", "16进制字符"}."16进制字符" ("传入类型")] -> w265
            tunnel: [_ T8."Read" ("校准命令") T8."Read_out" ("校准命令") T8."Read_out" ("校准命令") T8."Read" ("校准命令") T8."Set" ("校准命令") T8."Set Current Offset" ("校准命令") T8."Set Current Gain" ("校准命令") T8."Set Volt offset" ("校准命令") T8."Set Volt Gain" ("校准命令") T8."Set Current Offset 3" ("校准命令") T8."Set Current Gain 3" ("校准命令") T8."Set Current Offset 4" ("校准命令") T8."Set Current Gain 4" ("校准命令") _ T8."参数设置" ("校准命令") T8."写配置文件版本" ("校准命令") T9."读配置文件版本" ("校准命令") T10."Clear_in" ("校准命令") T10."Clear_out" ("校准命令") T8."Read_in" ("校准命令") T8."Read_in" ("校准命令") T8."Set_in" ("校准命令") T8."Set_out" ("校准命令")] -> w263
            frame "NULL", Default {
            }
            frame "Read1" {
            }
            frame "Read1_out" {
            }
            frame "Read2_out" {
            }
            frame "Read2" {
            }
            frame "Set" {
              n161 = local read "Gain"() -> (w941:dbl)
              n162 = Number To Hexadecimal String(1:i16 4 ("宽度(-)"), 2:w941) -> (0:w939:string)
            }
            frame "Set Current Offset" {
            }
            frame "Set Current Gain" {
            }
            frame "Set Volt offset" {
            }
            frame "Set Volt Gain" {
            }
            frame "Set Current Offset 3" {
            }
            frame "Set Current Gain 3" {
            }
            frame "Set Current Offset 4" {
              n163 = local read "充电能量阀值"() -> (w968:dbl)
              n164 = Number To Hexadecimal String(1:i16 8 ("宽度(-)"), 2:w968) -> (0:w969:string)
            }
            frame "Set Current Gain 4" {
              n165 = local read "分流器大小"() -> (w974:T2)
              n166 = Number To Hexadecimal String(1:i16 2 ("宽度(-)"), 2:w974) -> (0:w975:string)
            }
            frame "Clear" {
              (unwired) T8."Clear" ("校准命令")
            }
            frame "设置参数" {
              n167 = local read "config_data"() -> (w984:string)
            }
            frame "写配置文件版本" {
              n168 = local read "版本号"() -> (w988:string)
              n169 = String Subset(string=w988, length (rest)=8 ("长度（剩余）")) -> (substring=w989:string)  [unwired: 1 out]
            }
            frame "读配置文件版本" {
              n170 = local read "版本号"() -> (w993:string)
              n171 = String Subset(string=w993, length (rest)=8 ("长度（剩余）")) -> (substring=w994:string)  [unwired: 1 out]
            }
            frame "Clear_in" {
            }
            frame "Clear_out" {
            }
            frame "Read1_in" {
            }
            frame "Read2_in" {
            }
            frame "Set_in" {
              n172 = local read "Offset"() -> (w1021:i32)
              n173 = local read "Gain"() -> (w1022:dbl)
              n174 = Number To Hexadecimal String(1:i16 4 ("宽度(-)"), 2:w1022) -> (0:w1018:string)
              n175 = Number To Hexadecimal String(1:i16 8 ("宽度(-)"), 2:w1021) -> (0:w1017:string)
              n176 = Concatenate Strings(w1018, w1017) -> (w1016:string)
            }
            frame "Set_out" {
              n177 = local read "Offset"() -> (w1027:i32)
              n178 = local read "Gain"() -> (w1026:dbl)
              n179 = Number To Hexadecimal String(1:i16 4 ("宽度(-)"), 2:w1026) -> (0:w1030:string)
              n180 = Number To Hexadecimal String(1:i16 8 ("宽度(-)"), 2:w1027) -> (0:w1029:string)
              n181 = Concatenate Strings(w1030, w1029) -> (w1028:string)
            }
          }
          n182 = local read "CAN卡类型"() -> (w270:u32)
          n183 = disable-structure shown="禁用" {
            disable-tunnel: [w282 0.0 ("NG重测次数")] -> w279
            frame Disabled {
              n184 = local read "NG重测次数"() -> (w282:dbl)
            }
            frame Enabled {
            }
          }
          n185 = local read "滤波方式"() -> (w269:u8)
          n186 = local read "设备索引"() -> (w271:u16)
          n187 = local read "CAN路数"() -> (w272:u16)
          n188 = local read "工作方式"() -> (w268:u8)
          n189 = local read "波特率"() -> (w273:T3)
          n190 = call "高压板校正命令.vi"("CAN卡类型"=w270, "设备索引"=w271, "波特率"=w273, "CAN路数"=w272, "Data Input"=w274, "滤波方式"=w269, "传入类型"=w265, "工作方式"=w268, "校准命令"=w263) -> ("结果"=w267:bool, "VCI_CAN_OBJ_R"=w254:T5, "添加的数组"=w262:u8[], "错误输出"=w256:errorcluster)  [unwired: 3 in, 4 out]
          n191 = Equal?(x=w279, y=w278) -> (x = y?=w277:bool)
          n192 = call <vilib>:"Clear Errors.vi"("error in (no error)"=w256) -> ()  [unwired: 7 out]
          n193 = Index Array(array=w262) -> (element #1=w257:u8, element #2=w261:u8, element #3=w260:u8, element #4=w259:u8, element #5=w258:u8)  [unwired: 5 in]
          n194 = case shown="\"Read1_in\"" w281 {
            tunnel: "" ("转换结果") -> [_ _ _ _ _ _ _ _ _ _ _ _ _ _ _ _ _ _ _ _ _ _ _ _]
            tunnel: ["跳过..." ("布尔文本.文本") w297 w330 w356 w383 w409 w436 w459 w481 w516 _ w578 w613 w648 w684 w717 w748 w771 w789 w807 w824 w845 w866 w880] -> _
            tunnel: [TRUE w286 w319 w345 w372 w398 w426 w449 w470 w506 w530 w566 w601 w636 w671 w704 w738 w761 w782 w800 w817 w835 w856 w876] -> w266
            tunnel: FALSE -> [_ w293 w326 w352 w379 w405 w432 w455 w477 w512 w539 w574 w609 w644 w680 w713 w744 w767 w785 w803 w820 w841 w862 w878]
            tunnel: w277 -> [_ w294 w327 w353 w380 w406 w433 w456 w478 w513 w540 w575 w610 w645 w681 w714 w745 w768 w786 w804 w821 w842 w863 w879]
            tunnel: w267 -> [_ w286 w319 w345 w372 w398 w426 w449 w470 w506 w530 w566 w601 w636 w671 w704 w738 w761 w782 w800 w817 w836 w857 w877]
            tunnel: w261 -> [_ w289 w322 w348 w375 w401 w429 w452 w473 w509 w535 w570 w605 w640 w675 w708 w741 w764 _ _ _ w834 w855 _]
            tunnel: w260 -> [_ w288 w321 w347 w374 w400 _ _ w472 _ w534 w569 w604 w639 w674 w707 _ _ _ _ _ _ _ _]
            tunnel: w259 -> [_ _ _ _ _ _ _ _ _ _ w533 w568 w603 w638 w673 w706 _ _ _ _ _ _ _ _]
            tunnel: w258 -> [_ _ _ _ _ _ _ _ _ _ w532 w567 w602 w637 w672 w705 _ _ _ _ _ _ _ _]
            tunnel: w257 -> [_ _ _ _ _ _ _ _ _ _ _ _ _ _ _ _ _ _ _ _ _ _ _ _]
            tunnel: w254 -> [_ _ _ _ w371 _ _ _ _ _ _ _ _ _ _ _ _ _ _ _ _ _ _ _]
            frame "NULL", Default {
              n195 = call <vilib>:"Unset Busy.vi"() -> ()  [unwired: 2 in, 10 out]
            }
            frame "Read1" {
              n196 = case shown="真" w286 {
                tunnel: [_ w303] -> w290
                tunnel: w289 -> [_ w302]
                tunnel: w288 -> [_ w301]
                frame False {
                }
                frame True {
                  n197 = Join Numbers(hi=w302, lo=w301) -> ((hi.lo)=w303:u16)
                }
              }
              n198 = disable-structure shown="禁用" {
                disable-tunnel: w290 -> [w304 _]
                frame Disabled {
                  w307 = 500.0 ("x")
                  n199 = local read "REAL1"() -> (w310:dbl)
                  n200 = Multiply(x=w310, y=100.0) -> (x*y=w308:dbl)
                  n201 = Add(x=w307, y=w308) -> (x+y=w306:dbl)
                  n202 = Subtract(x=w308, y=w307) -> (x-y=w305:dbl)
                  n203 = In Range and Coerce(upper limit=w306, x=w304, lower limit=w305) -> ()  [unwired: 2 out]
                }
                frame Enabled {
                }
              }
              n204 = global write "EV05全局变量1.vi" "CAN接收"(TRUE ("CAN接收")) -> ()
              n205 = case shown="假" w286 {
                tunnel: cluster{u32, u32}[] [{6618880, 6618880}] ("颜色[4]") -> [w315 _]
                tunnel: cluster{u32, u32}[] [{15663131, 6618880}] ("颜色[4]") -> [_ w318]
                tunnel: [w315 w318] -> w298
                tunnel: ["OK" ("布尔文本.文本") "NG" ("布尔文本.文本")] -> w297
                frame True {
                  n206 = call <vilib>:"Unset Busy.vi"() -> ()  [unwired: 2 in, 10 out]
                }
                frame False {
                  n207 = call <vilib>:"Unset Busy.vi"() -> ()  [unwired: 2 in, 10 out]
                }
              }
              n208 = Not(x=w293) -> (.not. x?=w296:bool)
              n209 = And(x=w286, y=w296) -> (x .and. y?=w295:bool)
              n210 = And(x=w296, y=w294) -> (x .and. y?=w292:bool)
              n211 = Or(x=w295, y=w292) -> (x .or. y?=w291:bool)
              n212 = case shown="真" w291 {
                tunnel: w298 -> [_ w314]
                tunnel: w297 -> [_ w313]
                tunnel: w290 -> [_ w312]
                frame False {
                }
                frame True {
                  n213 = local write "AD1"(w312) -> ()
                  n214 = property on="Read1结果" class="Bool (严格)"("Colors [4]"=w314, "BoolText.Text"=w313) -> (error out=w311:errorcluster)  [unwired: 2 in, 1 out]
                  n215 = call <vilib>:"Clear Errors.vi"("error in (no error)"=w311) -> ()  [unwired: 7 out]
                }
              }
            }
            frame "Read1_out" {
              n216 = case shown="真" w319 {
                tunnel: [_ w336] -> w323
                tunnel: w322 -> [_ w335]
                tunnel: w321 -> [_ w334]
                frame False {
                }
                frame True {
                  n217 = Join Numbers(hi=w335, lo=w334) -> ((hi.lo)=w336:u16)
                }
              }
              n218 = global write "EV05全局变量1.vi" "CAN接收"(TRUE ("CAN接收")) -> ()
              n219 = case shown="假" w319 {
                tunnel: cluster{u32, u32}[] [{6618880, 6618880}] ("颜色[4]") -> [w341 _]
                tunnel: cluster{u32, u32}[] [{15663131, 6618880}] ("颜色[4]") -> [_ w344]
                tunnel: [w341 w344] -> w331
                tunnel: ["OK" ("布尔文本.文本") "NG" ("布尔文本.文本")] -> w330
                frame True {
                  n220 = call <vilib>:"Unset Busy.vi"() -> ()  [unwired: 2 in, 10 out]
                }
                frame False {
                  n221 = call <vilib>:"Unset Busy.vi"() -> ()  [unwired: 2 in, 10 out]
                }
              }
              n222 = Not(x=w326) -> (.not. x?=w329:bool)
              n223 = And(x=w319, y=w329) -> (x .and. y?=w328:bool)
              n224 = And(x=w329, y=w327) -> (x .and. y?=w325:bool)
              n225 = Or(x=w328, y=w325) -> (x .or. y?=w324:bool)
              n226 = case shown="真" w324 {
                tunnel: w331 -> [_ w340]
                tunnel: w330 -> [_ w339]
                tunnel: w323 -> [_ w338]
                frame False {
                }
                frame True {
                  n227 = local write "AD1"(w338) -> ()
                  n228 = property on="Read1_Out结果" class="Bool (严格)"("Colors [4]"=w340, "BoolText.Text"=w339) -> (error out=w337:errorcluster)  [unwired: 2 in, 1 out]
                  n229 = call <vilib>:"Clear Errors.vi"("error in (no error)"=w337) -> ()  [unwired: 7 out]
                }
              }
            }
            frame "Read2_out" {
              n230 = case shown="真" w345 {
                tunnel: [_ w362] -> w349
                tunnel: w348 -> [_ w361]
                tunnel: w347 -> [_ w360]
                frame False {
                }
                frame True {
                  n231 = Join Numbers(hi=w361, lo=w360) -> ((hi.lo)=w362:u16)
                }
              }
              n232 = global write "EV05全局变量1.vi" "CAN接收"(TRUE ("CAN接收")) -> ()
              n233 = case shown="假" w345 {
                tunnel: cluster{u32, u32}[] [{6618880, 6618880}] ("颜色[4]") -> [w367 _]
                tunnel: cluster{u32, u32}[] [{15663131, 6618880}] ("颜色[4]") -> [_ w370]
                tunnel: [w367 w370] -> w357
                tunnel: ["OK" ("布尔文本.文本") "NG" ("布尔文本.文本")] -> w356
                frame True {
                  n234 = call <vilib>:"Unset Busy.vi"() -> ()  [unwired: 2 in, 10 out]
                }
                frame False {
                  n235 = call <vilib>:"Unset Busy.vi"() -> ()  [unwired: 2 in, 10 out]
                }
              }
              n236 = Not(x=w352) -> (.not. x?=w355:bool)
              n237 = And(x=w345, y=w355) -> (x .and. y?=w354:bool)
              n238 = And(x=w355, y=w353) -> (x .and. y?=w351:bool)
              n239 = Or(x=w354, y=w351) -> (x .or. y?=w350:bool)
              n240 = case shown="真" w350 {
                tunnel: w357 -> [_ w366]
                tunnel: w356 -> [_ w365]
                tunnel: w349 -> [_ w364]
                frame False {
                }
                frame True {
                  n241 = local write "AD2"(w364) -> ()
                  n242 = property on="Read2_Out结果" class="Bool (严格)"("Colors [4]"=w366, "BoolText.Text"=w365) -> (error out=w363:errorcluster)  [unwired: 2 in, 1 out]
                  n243 = call <vilib>:"Clear Errors.vi"("error in (no error)"=w363) -> ()  [unwired: 7 out]
                }
              }
            }
            frame "Read1_in" {
              n244 = case shown="真" w372 {
                tunnel: [_ w389] -> w376
                tunnel: w375 -> [_ w388]
                tunnel: w374 -> [_ w387]
                frame False {
                }
                frame True {
                  n245 = Join Numbers(hi=w388, lo=w387) -> ((hi.lo)=w389:u16)
                }
              }
              n246 = global write "EV05全局变量1.vi" "CAN接收"(TRUE ("CAN接收")) -> ()
              n247 = case shown="假" w372 {
                tunnel: cluster{u32, u32}[] [{6618880, 6618880}] ("颜色[4]") -> [w394 _]
                tunnel: cluster{u32, u32}[] [{15663131, 6618880}] ("颜色[4]") -> [_ w397]
                tunnel: [w394 w397] -> w384
                tunnel: ["OK" ("布尔文本.文本") "NG" ("布尔文本.文本")] -> w383
                frame True {
                  n248 = call <vilib>:"Unset Busy.vi"() -> ()  [unwired: 2 in, 10 out]
                }
                frame False {
                  n249 = call <vilib>:"Unset Busy.vi"() -> ()  [unwired: 2 in, 10 out]
                }
              }
              n250 = Not(x=w379) -> (.not. x?=w382:bool)
              n251 = And(x=w372, y=w382) -> (x .and. y?=w381:bool)
              n252 = And(x=w382, y=w380) -> (x .and. y?=w378:bool)
              n253 = Or(x=w381, y=w378) -> (x .or. y?=w377:bool)
              n254 = case shown="真" w377 {
                tunnel: w384 -> [_ w393]
                tunnel: w383 -> [_ w392]
                tunnel: w376 -> [_ w391]
                tunnel: w371 -> [_ _]
                frame False {
                }
                frame True {
                  n255 = property on="Read1_in结果" class="Bool (严格)"("Colors [4]"=w393, "BoolText.Text"=w392) -> (error out=w390:errorcluster)  [unwired: 2 in, 1 out]
                  n256 = local write "AD1"(w391) -> ()
                  n257 = call <vilib>:"Clear Errors.vi"("error in (no error)"=w390) -> ()  [unwired: 7 out]
                }
              }
            }
            frame "Read2_in" {
              n258 = case shown="真" w398 {
                tunnel: [_ w415] -> w402
                tunnel: w401 -> [_ w414]
                tunnel: w400 -> [_ w413]
                frame False {
                }
                frame True {
                  n259 = Join Numbers(hi=w414, lo=w413) -> ((hi.lo)=w415:u16)
                }
              }
              n260 = global write "EV05全局变量1.vi" "CAN接收"(TRUE ("CAN接收")) -> ()
              n261 = case shown="假" w398 {
                tunnel: cluster{u32, u32}[] [{6618880, 6618880}] ("颜色[4]") -> [w420 _]
                tunnel: cluster{u32, u32}[] [{15663131, 6618880}] ("颜色[4]") -> [_ w423]
                tunnel: [w420 w423] -> w410
                tunnel: ["OK" ("布尔文本.文本") "NG" ("布尔文本.文本")] -> w409
                frame True {
                  n262 = call <vilib>:"Unset Busy.vi"() -> ()  [unwired: 2 in, 10 out]
                }
                frame False {
                  n263 = call <vilib>:"Unset Busy.vi"() -> ()  [unwired: 2 in, 10 out]
                }
              }
              n264 = Not(x=w405) -> (.not. x?=w408:bool)
              n265 = And(x=w398, y=w408) -> (x .and. y?=w407:bool)
              n266 = And(x=w408, y=w406) -> (x .and. y?=w404:bool)
              n267 = Or(x=w407, y=w404) -> (x .or. y?=w403:bool)
              n268 = case shown="真" w403 {
                tunnel: w410 -> [_ w419]
                tunnel: w409 -> [_ w418]
                tunnel: w402 -> [_ w417]
                frame False {
                }
                frame True {
                  n269 = local write "AD2"(w417) -> ()
                  n270 = property on="Read2_in结果" class="Bool (严格)"("Colors [4]"=w419, "BoolText.Text"=w418) -> (error out=w416:errorcluster)  [unwired: 2 in, 1 out]
                  n271 = call <vilib>:"Clear Errors.vi"("error in (no error)"=w416) -> ()  [unwired: 7 out]
                }
              }
            }
            frame "Set_in" {
              n272 = Equal?(x=w429, y=u8 1 ("x")) -> (x = y?=w427:bool)
              n273 = global write "EV05全局变量1.vi" "CAN接收"(TRUE ("CAN接收")) -> ()
              n274 = And(x=w427, y=w426) -> (x .and. y?=w425:bool)
              n275 = case shown="假" w425 {
                tunnel: cluster{u32, u32}[] [{6618880, 6618880}] ("颜色[4]") -> [w443 _]
                tunnel: cluster{u32, u32}[] [{15663131, 6618880}] ("颜色[4]") -> [_ w446]
                tunnel: [w443 w446] -> w437
                tunnel: ["OK" ("布尔文本.文本") "NG" ("布尔文本.文本")] -> w436
                frame True {
                  n276 = call <vilib>:"Unset Busy.vi"() -> ()  [unwired: 2 in, 10 out]
                }
                frame False {
                  n277 = call <vilib>:"Unset Busy.vi"() -> ()  [unwired: 2 in, 10 out]
                }
              }
              n278 = Not(x=w432) -> (.not. x?=w435:bool)
              n279 = And(x=w426, y=w435) -> (x .and. y?=w434:bool)
              n280 = And(x=w435, y=w433) -> (x .and. y?=w431:bool)
              n281 = Or(x=w434, y=w431) -> (x .or. y?=w430:bool)
              n282 = case shown="真" w430 {
                tunnel: w437 -> [_ w442]
                tunnel: w436 -> [_ w441]
                frame False {
                }
                frame True {
                  n283 = property on="Set_in结果" class="Bool (严格)"("Colors [4]"=w442, "BoolText.Text"=w441) -> (error out=w440:errorcluster)  [unwired: 2 in, 1 out]
                  n284 = call <vilib>:"Clear Errors.vi"("error in (no error)"=w440) -> ()  [unwired: 7 out]
                }
              }
            }
            frame "Set_out" {
              n285 = Equal?(x=w452, y=u8 1) -> (x = y?=w450:bool)
              n286 = global write "EV05全局变量1.vi" "CAN接收"(TRUE ("CAN接收")) -> ()
              n287 = And(x=w450, y=w449) -> (x .and. y?=w448:bool)
              n288 = case shown="假" w448 {
                tunnel: cluster{u32, u32}[] [{6618880, 6618880}] ("颜色[4]") -> [w466 _]
                tunnel: cluster{u32, u32}[] [{15663131, 6618880}] ("颜色[4]") -> [_ w469]
                tunnel: [w466 w469] -> w460
                tunnel: ["OK" ("布尔文本.文本") "NG" ("布尔文本.文本")] -> w459
                frame True {
                  n289 = call <vilib>:"Unset Busy.vi"() -> ()  [unwired: 2 in, 10 out]
                }
                frame False {
                  n290 = call <vilib>:"Unset Busy.vi"() -> ()  [unwired: 2 in, 10 out]
                }
              }
              n291 = Not(x=w455) -> (.not. x?=w458:bool)
              n292 = And(x=w449, y=w458) -> (x .and. y?=w457:bool)
              n293 = And(x=w458, y=w456) -> (x .and. y?=w454:bool)
              n294 = Or(x=w457, y=w454) -> (x .or. y?=w453:bool)
              n295 = case shown="真" w453 {
                tunnel: w460 -> [_ w465]
                tunnel: w459 -> [_ w464]
                frame False {
                }
                frame True {
                  n296 = property on="Set_out结果" class="Bool (严格)"("Colors [4]"=w465, "BoolText.Text"=w464) -> (error out=w463:errorcluster)  [unwired: 2 in, 1 out]
                  n297 = call <vilib>:"Clear Errors.vi"("error in (no error)"=w463) -> ()  [unwired: 7 out]
                }
              }
            }
            frame "Read2" {
              n298 = case shown="真" w470 {
                tunnel: [_ w487] -> w474
                tunnel: w473 -> [_ w486]
                tunnel: w472 -> [_ w485]
                frame False {
                }
                frame True {
                  n299 = Join Numbers(hi=w486, lo=w485) -> ((hi.lo)=w487:u16)
                }
              }
              n300 = disable-structure shown="禁用" {
                disable-tunnel: w474 -> [w489 _]
                frame Disabled {
                  w492 = 500.0 ("x")
                  n301 = local read "REAL2"() -> (w488:dbl)
                  n302 = Multiply(x=w488, y=100.0) -> (x*y=w493:dbl)
                  n303 = Add(x=w492, y=w493) -> (x+y=w491:dbl)
                  n304 = Subtract(x=w493, y=w492) -> (x-y=w490:dbl)
                  n305 = In Range and Coerce(upper limit=w491, x=w489, lower limit=w490) -> ()  [unwired: 2 out]
                }
                frame Enabled {
                }
              }
              n306 = global write "EV05全局变量1.vi" "CAN接收"(TRUE ("CAN接收")) -> ()
              n307 = case shown="假" w470 {
                tunnel: cluster{u32, u32}[] [{6618880, 6618880}] ("颜色[4]") -> [w499 _]
                tunnel: cluster{u32, u32}[] [{15663131, 6618880}] ("颜色[4]") -> [_ w502]
                tunnel: [w499 w502] -> w482
                tunnel: ["OK" ("布尔文本.文本") "NG" ("布尔文本.文本")] -> w481
                frame True {
                  n308 = call <vilib>:"Unset Busy.vi"() -> ()  [unwired: 2 in, 10 out]
                }
                frame False {
                  n309 = call <vilib>:"Unset Busy.vi"() -> ()  [unwired: 2 in, 10 out]
                }
              }
              n310 = Not(x=w477) -> (.not. x?=w480:bool)
              n311 = And(x=w470, y=w480) -> (x .and. y?=w479:bool)
              n312 = And(x=w480, y=w478) -> (x .and. y?=w476:bool)
              n313 = Or(x=w479, y=w476) -> (x .or. y?=w475:bool)
              n314 = case shown="真" w475 {
                tunnel: w482 -> [_ w498]
                tunnel: w481 -> [_ w497]
                tunnel: w474 -> [_ w496]
                frame False {
                }
                frame True {
                  n315 = local write "AD2"(w496) -> ()
                  n316 = property on="Read2结果" class="Bool (严格)"("Colors [4]"=w498, "BoolText.Text"=w497) -> (error out=w495:errorcluster)  [unwired: 2 in, 1 out]
                  n317 = call <vilib>:"Clear Errors.vi"("error in (no error)"=w495) -> ()  [unwired: 7 out]
                }
              }
            }
            frame "Set" {
              n318 = Equal?(x=w509, y=u8 1) -> (x = y?=w507:bool)
              n319 = disable-structure shown="禁用" {
                frame Disabled {
                  n320 = local read "Gain"() -> (w521:dbl)
                  n321 = In Range and Coerce(upper limit=100.0 ("上限"), x=w521, lower limit=94.0 ("上限")) -> (In Range?=w519:bool)  [unwired: 1 out]
                  n322 = And(x=w519, y=w519) -> ()  [unwired: 1 out]
                }
                frame Enabled {
                }
              }
              n323 = global write "EV05全局变量1.vi" "CAN接收"(TRUE ("CAN接收")) -> ()
              n324 = And(x=w507, y=w506) -> (x .and. y?=w505:bool)
              n325 = case shown="假" w505 {
                tunnel: cluster{u32, u32}[] [{6618880, 6618880}] ("颜色[4]") -> [w526 _]
                tunnel: cluster{u32, u32}[] [{15663131, 6618880}] ("颜色[4]") -> [_ w529]
                tunnel: [w526 w529] -> w517
                tunnel: ["OK" ("布尔文本.文本") "NG" ("布尔文本.文本")] -> w516
                frame True {
                  n326 = call <vilib>:"Unset Busy.vi"() -> ()  [unwired: 2 in, 10 out]
                }
                frame False {
                  n327 = call <vilib>:"Unset Busy.vi"() -> ()  [unwired: 2 in, 10 out]
                }
              }
              n328 = Not(x=w512) -> (.not. x?=w515:bool)
              n329 = And(x=w506, y=w515) -> (x .and. y?=w514:bool)
              n330 = And(x=w515, y=w513) -> (x .and. y?=w511:bool)
              n331 = Or(x=w514, y=w511) -> (x .or. y?=w510:bool)
              n332 = case shown="真" w510 {
                tunnel: w517 -> [_ w525]
                tunnel: w516 -> [_ w524]
                frame False {
                }
                frame True {
                  n333 = property on="Set结果" class="Bool (严格)"("Colors [4]"=w525, "BoolText.Text"=w524) -> (error out=w523:errorcluster)  [unwired: 2 in, 1 out]
                  n334 = call <vilib>:"Clear Errors.vi"("error in (no error)"=w523) -> ()  [unwired: 7 out]
                }
              }
            }
            frame "Set Current Offset" {
              n335 = case shown="假" w530 {
                tunnel: [_ w553] -> w536
                tunnel: w535 -> [_ w550]
                tunnel: w534 -> [_ w549]
                tunnel: w533 -> [_ w548]
                tunnel: w532 -> [_ w547]
                frame False {
                }
                frame True {
                  w552 = i16 2 ("宽度(-)")
                  n336 = Number To Hexadecimal String(1:w552, 2:w549) -> (0:w555:string)
                  n337 = Number To Hexadecimal String(1:w552, 2:w548) -> (0:w554:string)
                  n338 = Number To Hexadecimal String(1:w552, 2:w550) -> (0:w556:string)
                  n339 = Number To Hexadecimal String(1:w552, 2:w547) -> (0:w551:string)
                  n340 = Concatenate Strings(w556, w555, w554, w551) -> (w553:string)
                }
              }
              n341 = global write "EV05全局变量1.vi" "CAN接收"(TRUE ("CAN接收")) -> ()
              n342 = case shown="真" w530 {
                tunnel: cluster{u32, u32}[] [{6618880, 6618880}] ("颜色[4]") -> [w561 _]
                tunnel: cluster{u32, u32}[] [{15663131, 6618880}] ("颜色[4]") -> [_ w564]
                tunnel: [w561 w564] -> w544
                tunnel: ["OK" ("布尔文本.文本") "NG" ("布尔文本.文本")] -> w543
                frame True {
                  n343 = call <vilib>:"Unset Busy.vi"() -> ()  [unwired: 2 in, 10 out]
                }
                frame False {
                  n344 = call <vilib>:"Unset Busy.vi"() -> ()  [unwired: 2 in, 10 out]
                }
              }
              n345 = Not(x=w539) -> (.not. x?=w542:bool)
              n346 = And(x=w530, y=w542) -> (x .and. y?=w541:bool)
              n347 = And(x=w542, y=w540) -> (x .and. y?=w538:bool)
              n348 = Or(x=w541, y=w538) -> (x .or. y?=w537:bool)
              n349 = case shown="真" w537 {
                tunnel: w544 -> [_ w560]
                tunnel: w543 -> [_ w559]
                tunnel: w536 -> [_ w558]
                frame False {
                }
                frame True {
                  n350 = property on="Current Offset结果" class="Bool (严格)"("Colors [4]"=w560, "BoolText.Text"=w559) -> (error out=w557:errorcluster)  [unwired: 2 in, 1 out]
                  n351 = local write "电流零点"(w558) -> ()
                  n352 = call <vilib>:"Clear Errors.vi"("error in (no error)"=w557) -> ()  [unwired: 7 out]
                }
              }
            }
            frame "Set Current Gain" {
              n353 = case shown="真" w566 {
                tunnel: [_ w588] -> w571
                tunnel: w570 -> [_ w585]
                tunnel: w569 -> [_ w584]
                tunnel: w568 -> [_ w583]
                tunnel: w567 -> [_ w582]
                frame False {
                }
                frame True {
                  w587 = i16 2 ("宽度(-)")
                  n354 = Number To Hexadecimal String(1:w587, 2:w584) -> (0:w590:string)
                  n355 = Number To Hexadecimal String(1:w587, 2:w585) -> (0:w591:string)
                  n356 = Number To Hexadecimal String(1:w587, 2:w582) -> (0:w586:string)
                  n357 = Number To Hexadecimal String(1:w587, 2:w583) -> (0:w589:string)
                  n358 = Concatenate Strings(w591, w590, w589, w586) -> (w588:string)
                }
              }
              n359 = global write "EV05全局变量1.vi" "CAN接收"(TRUE ("CAN接收")) -> ()
              n360 = case shown="真" w566 {
                tunnel: cluster{u32, u32}[] [{6618880, 6618880}] ("颜色[4]") -> [w596 _]
                tunnel: cluster{u32, u32}[] [{15663131, 6618880}] ("颜色[4]") -> [_ w599]
                tunnel: [w596 w599] -> w579
                tunnel: ["OK" ("布尔文本.文本") "NG" ("布尔文本.文本")] -> w578
                frame True {
                  n361 = call <vilib>:"Unset Busy.vi"() -> ()  [unwired: 2 in, 10 out]
                }
                frame False {
                  n362 = call <vilib>:"Unset Busy.vi"() -> ()  [unwired: 2 in, 10 out]
                }
              }
              n363 = Not(x=w574) -> (.not. x?=w577:bool)
              n364 = And(x=w566, y=w577) -> (x .and. y?=w576:bool)
              n365 = And(x=w577, y=w575) -> (x .and. y?=w573:bool)
              n366 = Or(x=w576, y=w573) -> (x .or. y?=w572:bool)
              n367 = case shown="真" w572 {
                tunnel: w579 -> [_ w595]
                tunnel: w578 -> [_ w594]
                tunnel: w571 -> [_ w593]
                frame False {
                }
                frame True {
                  n368 = local write "电流增益"(w593) -> ()
                  n369 = property on="Current Gain结果" class="Bool (严格)"("Colors [4]"=w595, "BoolText.Text"=w594) -> (error out=w592:errorcluster)  [unwired: 2 in, 1 out]
                  n370 = call <vilib>:"Clear Errors.vi"("error in (no error)"=w592) -> ()  [unwired: 7 out]
                }
              }
            }
            frame "Set Volt offset" {
              n371 = case shown="真" w601 {
                tunnel: [_ w623] -> w606
                tunnel: w605 -> [_ w620]
                tunnel: w604 -> [_ w619]
                tunnel: w603 -> [_ w618]
                tunnel: w602 -> [_ w617]
                frame False {
                }
                frame True {
                  w622 = i16 2 ("宽度(-)")
                  n372 = Number To Hexadecimal String(1:w622, 2:w619) -> (0:w625:string)
                  n373 = Number To Hexadecimal String(1:w622, 2:w620) -> (0:w626:string)
                  n374 = Number To Hexadecimal String(1:w622, 2:w618) -> (0:w624:string)
                  n375 = Number To Hexadecimal String(1:w622, 2:w617) -> (0:w621:string)
                  n376 = Concatenate Strings(w626, w625, w624, w621) -> (w623:string)
                }
              }
              n377 = global write "EV05全局变量1.vi" "CAN接收"(TRUE ("CAN接收")) -> ()
              n378 = case shown="假" w601 {
                tunnel: cluster{u32, u32}[] [{6618880, 6618880}] ("颜色[4]") -> [w631 _]
                tunnel: cluster{u32, u32}[] [{15663131, 6618880}] ("颜色[4]") -> [_ w634]
                tunnel: [w631 w634] -> w614
                tunnel: ["OK" ("布尔文本.文本") "NG" ("布尔文本.文本")] -> w613
                frame True {
                  n379 = call <vilib>:"Unset Busy.vi"() -> ()  [unwired: 2 in, 10 out]
                }
                frame False {
                  n380 = call <vilib>:"Unset Busy.vi"() -> ()  [unwired: 2 in, 10 out]
                }
              }
              n381 = Not(x=w609) -> (.not. x?=w612:bool)
              n382 = And(x=w601, y=w612) -> (x .and. y?=w611:bool)
              n383 = And(x=w612, y=w610) -> (x .and. y?=w608:bool)
              n384 = Or(x=w611, y=w608) -> (x .or. y?=w607:bool)
              n385 = case shown="真" w607 {
                tunnel: w614 -> [_ w630]
                tunnel: w613 -> [_ w629]
                tunnel: w606 -> [_ w628]
                frame False {
                }
                frame True {
                  n386 = local write "Shunt Volt Offset"(w628) -> ()
                  n387 = property on="Current Offset结果 2" class="Bool (严格)"("Colors [4]"=w630, "BoolText.Text"=w629) -> (error out=w627:errorcluster)  [unwired: 2 in, 1 out]
                  n388 = call <vilib>:"Clear Errors.vi"("error in (no error)"=w627) -> ()  [unwired: 7 out]
                }
              }
            }
            frame "Set Volt Gain" {
              n389 = case shown="真" w636 {
                tunnel: [_ w658] -> w641
                tunnel: w640 -> [_ w655]
                tunnel: w639 -> [_ w654]
                tunnel: w638 -> [_ w653]
                tunnel: w637 -> [_ w652]
                frame False {
                }
                frame True {
                  w657 = i16 2 ("宽度(-)")
                  n390 = Number To Hexadecimal String(1:w657, 2:w653) -> (0:w659:string)
                  n391 = Number To Hexadecimal String(1:w657, 2:w652) -> (0:w656:string)
                  n392 = Number To Hexadecimal String(1:w657, 2:w654) -> (0:w660:string)
                  n393 = Number To Hexadecimal String(1:w657, 2:w655) -> (0:w661:string)
                  n394 = Concatenate Strings(w661, w660, w659, w656) -> (w658:string)
                }
              }
              n395 = global write "EV05全局变量1.vi" "CAN接收"(TRUE ("CAN接收")) -> ()
              n396 = case shown="假" w636 {
                tunnel: cluster{u32, u32}[] [{6618880, 6618880}] ("颜色[4]") -> [w666 _]
                tunnel: cluster{u32, u32}[] [{15663131, 6618880}] ("颜色[4]") -> [_ w669]
                tunnel: [w666 w669] -> w649
                tunnel: ["OK" ("布尔文本.文本") "NG" ("布尔文本.文本")] -> w648
                frame True {
                  n397 = call <vilib>:"Unset Busy.vi"() -> ()  [unwired: 2 in, 10 out]
                }
                frame False {
                  n398 = call <vilib>:"Unset Busy.vi"() -> ()  [unwired: 2 in, 10 out]
                }
              }
              n399 = Not(x=w644) -> (.not. x?=w647:bool)
              n400 = And(x=w636, y=w647) -> (x .and. y?=w646:bool)
              n401 = And(x=w647, y=w645) -> (x .and. y?=w643:bool)
              n402 = Or(x=w646, y=w643) -> (x .or. y?=w642:bool)
              n403 = case shown="真" w642 {
                tunnel: w649 -> [_ w665]
                tunnel: w648 -> [_ w664]
                tunnel: w641 -> [_ w663]
                frame False {
                }
                frame True {
                  n404 = local write "Shunt Volt Gain"(w663) -> ()
                  n405 = property on="Current Gain结果 2" class="Bool (严格)"("Colors [4]"=w665, "BoolText.Text"=w664) -> (error out=w662:errorcluster)  [unwired: 2 in, 1 out]
                  n406 = call <vilib>:"Clear Errors.vi"("error in (no error)"=w662) -> ()  [unwired: 7 out]
                }
              }
            }
            frame "Set Current Offset 3" {
              n407 = case shown="真" w671 {
                tunnel: [_ w693] -> w677
                tunnel: [_ w692] -> w676
                tunnel: w675 -> [_ w691]
                tunnel: w674 -> [_ w690]
                tunnel: w673 -> [_ w689]
                tunnel: w672 -> [_ w688]
                frame False {
                }
                frame True {
                  n408 = Join Numbers(hi=w691, lo=w690) -> ((hi.lo)=w693:u16)
                  n409 = Join Numbers(hi=w689, lo=w688) -> ((hi.lo)=w692:u16)
                }
              }
              n410 = global write "EV05全局变量1.vi" "CAN接收"(TRUE ("CAN接收")) -> ()
              n411 = case shown="假" w671 {
                tunnel: cluster{u32, u32}[] [{6618880, 6618880}] ("颜色[4]") -> [w699 _]
                tunnel: cluster{u32, u32}[] [{15663131, 6618880}] ("颜色[4]") -> [_ w702]
                tunnel: [w699 w702] -> w685
                tunnel: ["OK" ("布尔文本.文本") "NG" ("布尔文本.文本")] -> w684
                frame True {
                  n412 = call <vilib>:"Unset Busy.vi"() -> ()  [unwired: 2 in, 10 out]
                }
                frame False {
                  n413 = call <vilib>:"Unset Busy.vi"() -> ()  [unwired: 2 in, 10 out]
                }
              }
              n414 = Not(x=w680) -> (.not. x?=w683:bool)
              n415 = And(x=w671, y=w683) -> (x .and. y?=w682:bool)
              n416 = And(x=w683, y=w681) -> (x .and. y?=w679:bool)
              n417 = Or(x=w682, y=w679) -> (x .or. y?=w678:bool)
              n418 = case shown="真" w678 {
                tunnel: w685 -> [_ w698]
                tunnel: w684 -> [_ w697]
                tunnel: w677 -> [_ w696]
                tunnel: w676 -> [_ w695]
                frame False {
                }
                frame True {
                  n419 = property on="Current Offset结果 3" class="Bool (严格)"("Colors [4]"=w698, "BoolText.Text"=w697) -> (error out=w694:errorcluster)  [unwired: 2 in, 1 out]
                  n420 = local write "平均电流"(w695) -> ()
                  n421 = local write "电流增益"(w696) -> ()
                  n422 = call <vilib>:"Clear Errors.vi"("error in (no error)"=w694) -> ()  [unwired: 7 out]
                }
              }
            }
            frame "Set Current Gain 3" {
              n423 = case shown="真" w704 {
                tunnel: [_ w726] -> w710
                tunnel: [_ w725] -> w709
                tunnel: w708 -> [_ w724]
                tunnel: w707 -> [_ w723]
                tunnel: w706 -> [_ w722]
                tunnel: w705 -> [_ w721]
                frame False {
                }
                frame True {
                  n424 = Join Numbers(hi=w724, lo=w723) -> ((hi.lo)=w726:u16)
                  n425 = Join Numbers(hi=w722, lo=w721) -> ((hi.lo)=w725:u16)
                }
              }
              n426 = global write "EV05全局变量1.vi" "CAN接收"(TRUE ("CAN接收")) -> ()
              n427 = case shown="假" w704 {
                tunnel: cluster{u32, u32}[] [{6618880, 6618880}] ("颜色[4]") -> [w732 _]
                tunnel: cluster{u32, u32}[] [{15663131, 6618880}] ("颜色[4]") -> [_ w735]
                tunnel: [w732 w735] -> w718
                tunnel: ["OK" ("布尔文本.文本") "NG" ("布尔文本.文本")] -> w717
                frame True {
                  n428 = call <vilib>:"Unset Busy.vi"() -> ()  [unwired: 2 in, 10 out]
                }
                frame False {
                  n429 = call <vilib>:"Unset Busy.vi"() -> ()  [unwired: 2 in, 10 out]
                }
              }
              n430 = Not(x=w713) -> (.not. x?=w716:bool)
              n431 = And(x=w704, y=w716) -> (x .and. y?=w715:bool)
              n432 = And(x=w716, y=w714) -> (x .and. y?=w712:bool)
              n433 = Or(x=w715, y=w712) -> (x .or. y?=w711:bool)
              n434 = case shown="真" w711 {
                tunnel: w718 -> [_ w731]
                tunnel: w717 -> [_ w730]
                tunnel: w710 -> [_ w729]
                tunnel: w709 -> [_ w728]
                frame False {
                }
                frame True {
                  n435 = property on="Current Gain结果 3" class="Bool (严格)"("Colors [4]"=w731, "BoolText.Text"=w730) -> (error out=w727:errorcluster)  [unwired: 2 in, 1 out]
                  n436 = local write "电压增益"(w729) -> ()
                  n437 = local write "平均电压"(w728) -> ()
                  n438 = call <vilib>:"Clear Errors.vi"("error in (no error)"=w727) -> ()  [unwired: 7 out]
                }
              }
            }
            frame "Set Current Offset 4" {
              n439 = Equal?(x=w741, y=u8 1) -> (x = y?=w739:bool)
              n440 = global write "EV05全局变量1.vi" "CAN接收"(TRUE ("CAN接收")) -> ()
              n441 = And(x=w739, y=w738) -> (x .and. y?=w737:bool)
              n442 = case shown="假" w737 {
                tunnel: cluster{u32, u32}[] [{6618880, 6618880}] ("颜色[4]") -> [w755 _]
                tunnel: cluster{u32, u32}[] [{15663131, 6618880}] ("颜色[4]") -> [_ w758]
                tunnel: [w755 w758] -> w749
                tunnel: ["OK" ("布尔文本.文本") "NG" ("布尔文本.文本")] -> w748
                frame True {
                  n443 = call <vilib>:"Unset Busy.vi"() -> ()  [unwired: 2 in, 10 out]
                }
                frame False {
                  n444 = call <vilib>:"Unset Busy.vi"() -> ()  [unwired: 2 in, 10 out]
                }
              }
              n445 = Not(x=w744) -> (.not. x?=w747:bool)
              n446 = And(x=w738, y=w747) -> (x .and. y?=w746:bool)
              n447 = And(x=w747, y=w745) -> (x .and. y?=w743:bool)
              n448 = Or(x=w746, y=w743) -> (x .or. y?=w742:bool)
              n449 = case shown="真" w742 {
                tunnel: w749 -> [_ w754]
                tunnel: w748 -> [_ w753]
                frame False {
                }
                frame True {
                  n450 = property on="Current Offset结果 4" class="Bool (严格)"("Colors [4]"=w754, "BoolText.Text"=w753) -> (error out=w752:errorcluster)  [unwired: 2 in, 1 out]
                  n451 = call <vilib>:"Clear Errors.vi"("error in (no error)"=w752) -> ()  [unwired: 7 out]
                }
              }
            }
            frame "Set Current Gain 4" {
              n452 = Equal?(x=w764, y=u8 1) -> (x = y?=w762:bool)
              n453 = And(x=w762, y=w761) -> (x .and. y?=w760:bool)
              n454 = global write "EV05全局变量1.vi" "CAN接收"(TRUE ("CAN接收")) -> ()
              n455 = case shown="假" w760 {
                tunnel: cluster{u32, u32}[] [{6618880, 6618880}] ("颜色[4]") -> [w778 _]
                tunnel: cluster{u32, u32}[] [{15663131, 6618880}] ("颜色[4]") -> [_ w781]
                tunnel: [w778 w781] -> w772
                tunnel: ["OK" ("布尔文本.文本") "NG" ("布尔文本.文本")] -> w771
                frame True {
                  n456 = call <vilib>:"Unset Busy.vi"() -> ()  [unwired: 2 in, 10 out]
                }
                frame False {
                  n457 = call <vilib>:"Unset Busy.vi"() -> ()  [unwired: 2 in, 10 out]
                }
              }
              n458 = Not(x=w767) -> (.not. x?=w770:bool)
              n459 = And(x=w761, y=w770) -> (x .and. y?=w769:bool)
              n460 = And(x=w770, y=w768) -> (x .and. y?=w766:bool)
              n461 = Or(x=w769, y=w766) -> (x .or. y?=w765:bool)
              n462 = case shown="真" w765 {
                tunnel: w772 -> [_ w777]
                tunnel: w771 -> [_ w776]
                frame False {
                }
                frame True {
                  n463 = property on="Current Gain结果 4" class="Bool (严格)"("Colors [4]"=w777, "BoolText.Text"=w776) -> (error out=w775:errorcluster)  [unwired: 2 in, 1 out]
                  n464 = call <vilib>:"Clear Errors.vi"("error in (no error)"=w775) -> ()  [unwired: 7 out]
                }
              }
            }
            frame "Clear_in" {
              n465 = case shown="真" w782 {
                tunnel: cluster{u32, u32}[] [{6618880, 6618880}] ("颜色[4]") -> [w796 _]
                tunnel: cluster{u32, u32}[] [{15663131, 6618880}] ("颜色[4]") -> [_ w799]
                tunnel: [w796 w799] -> w790
                tunnel: ["OK" ("布尔文本.文本") "NG" ("布尔文本.文本")] -> w789
                frame True {
                }
                frame False {
                }
              }
              n466 = Not(x=w785) -> (.not. x?=w788:bool)
              n467 = And(x=w782, y=w788) -> (x .and. y?=w787:bool)
              n468 = And(x=w788, y=w786) -> (x .and. y?=w784:bool)
              n469 = Or(x=w787, y=w784) -> (x .or. y?=w783:bool)
              n470 = case shown="真" w783 {
                tunnel: w790 -> [_ w795]
                tunnel: w789 -> [_ w794]
                frame False {
                }
                frame True {
                  n471 = property on="Clear_in结果" class="Bool (严格)"("Colors [4]"=w795, "BoolText.Text"=w794) -> (error out=w793:errorcluster)  [unwired: 2 in, 1 out]
                  n472 = call <vilib>:"Clear Errors.vi"("error in (no error)"=w793) -> ()  [unwired: 7 out]
                }
              }
            }
            frame "Clear_out" {
              n473 = case shown="真" w800 {
                tunnel: cluster{u32, u32}[] [{6618880, 6618880}] ("颜色[4]") -> [w813 _]
                tunnel: cluster{u32, u32}[] [{15663131, 6618880}] ("颜色[4]") -> [_ w816]
                tunnel: [w813 w816] -> w808
                tunnel: ["OK" ("布尔文本.文本") "NG" ("布尔文本.文本")] -> w807
                frame True {
                }
                frame False {
                }
              }
              n474 = Not(x=w803) -> (.not. x?=w806:bool)
              n475 = And(x=w800, y=w806) -> (x .and. y?=w805:bool)
              n476 = And(x=w806, y=w804) -> (x .and. y?=w802:bool)
              n477 = Or(x=w805, y=w802) -> (x .or. y?=w801:bool)
              n478 = case shown="真" w801 {
                tunnel: w808 -> [_ w812]
                tunnel: w807 -> [_ w811]
                frame False {
                }
                frame True {
                  n479 = property on="Clear_out结果" class="Bool (严格)"("Colors [4]"=w812, "BoolText.Text"=w811) -> ()  [unwired: 2 in, 2 out]
                }
              }
            }
            frame "Clear" {
              n480 = case shown="真" w817 {
                tunnel: cluster{u32, u32}[] [{6618880, 6618880}] ("颜色[4]") -> [w830 _]
                tunnel: cluster{u32, u32}[] [{15663131, 6618880}] ("颜色[4]") -> [_ w833]
                tunnel: [w830 w833] -> w825
                tunnel: ["OK" ("布尔文本.文本") "NG" ("布尔文本.文本")] -> w824
                frame True {
                }
                frame False {
                }
              }
              n481 = Not(x=w820) -> (.not. x?=w823:bool)
              n482 = And(x=w817, y=w823) -> (x .and. y?=w822:bool)
              n483 = And(x=w823, y=w821) -> (x .and. y?=w819:bool)
              n484 = Or(x=w822, y=w819) -> (x .or. y?=w818:bool)
              n485 = case shown="真" w818 {
                tunnel: w825 -> [_ w829]
                tunnel: w824 -> [_ w828]
                frame False {
                }
                frame True {
                  n486 = property on="Clear结果" class="Bool (严格)"("Colors [4]"=w829, "BoolText.Text"=w828) -> ()  [unwired: 2 in, 2 out]
                }
              }
            }
            frame "设置参数" {
              n487 = Equal?(x=w834, y=u8 1) -> (x = y?=w837:bool)
              n488 = And(x=w837, y=w836) -> (x .and. y?=w835:bool)
              n489 = case shown="真" w835 {
                tunnel: cluster{u32, u32}[] [{6618880, 6618880}] ("颜色[4]") -> [w851 _]
                tunnel: cluster{u32, u32}[] [{15663131, 6618880}] ("颜色[4]") -> [_ w854]
                tunnel: [w851 w854] -> w846
                tunnel: ["OK" ("布尔文本.文本") "NG" ("布尔文本.文本")] -> w845
                frame True {
                }
                frame False {
                }
              }
              n490 = Not(x=w841) -> (.not. x?=w844:bool)
              n491 = And(x=w835, y=w844) -> (x .and. y?=w843:bool)
              n492 = And(x=w844, y=w842) -> (x .and. y?=w840:bool)
              n493 = Or(x=w843, y=w840) -> (x .or. y?=w839:bool)
              n494 = case shown="真" w839 {
                tunnel: w846 -> [_ w850]
                tunnel: w845 -> [_ w849]
                frame False {
                }
                frame True {
                  n495 = property on="连接状态 10" class="Bool (严格)"("Colors [4]"=w850, "BoolText.Text"=w849) -> ()  [unwired: 2 in, 2 out]
                }
              }
            }
            frame "写配置文件版本" {
              n496 = Equal?(x=w855, y=u8 1) -> (x = y?=w858:bool)
              n497 = And(x=w858, y=w857) -> (x .and. y?=w856:bool)
              n498 = case shown="真" w856 {
                tunnel: cluster{u32, u32}[] [{6618880, 6618880}] ("颜色[4]") -> [w872 _]
                tunnel: cluster{u32, u32}[] [{15663131, 6618880}] ("颜色[4]") -> [_ w875]
                tunnel: [w872 w875] -> w867
                tunnel: ["OK" ("布尔文本.文本") "NG" ("布尔文本.文本")] -> w866
                frame True {
                }
                frame False {
                }
              }
              n499 = Not(x=w862) -> (.not. x?=w865:bool)
              n500 = And(x=w856, y=w865) -> (x .and. y?=w864:bool)
              n501 = And(x=w865, y=w863) -> (x .and. y?=w861:bool)
              n502 = Or(x=w864, y=w861) -> (x .or. y?=w860:bool)
              n503 = case shown="真" w860 {
                tunnel: w867 -> [_ w871]
                tunnel: w866 -> [_ w870]
                frame False {
                }
                frame True {
                  n504 = property on="写版本结果" class="Bool (严格)"("Colors [4]"=w871, "BoolText.Text"=w870) -> ()  [unwired: 2 in, 2 out]
                }
              }
            }
            frame "读配置文件版本" {
              n505 = disable-structure shown="禁用" {
                disable-tunnel: [w890 _] -> w880
                disable-tunnel: w879 -> [w887 _]
                disable-tunnel: w878 -> [w886 _]
                disable-tunnel: w877 -> [w883 _]
                disable-tunnel: [w882 _] -> w876
                frame Disabled {
                  n506 = And(x=TRUE, y=w883) -> (x .and. y?=w882:bool)
                  n507 = case shown="真" w882 {
                    tunnel: cluster{u32, u32}[] [{6618880, 6618880}] ("颜色[4]") -> [w894 _]
                    tunnel: cluster{u32, u32}[] [{15663131, 6618880}] ("颜色[4]") -> [_ w897]
                    tunnel: [w894 w897] -> w891
                    tunnel: ["OK" ("布尔文本.文本") "NG" ("布尔文本.文本")] -> w890
                    frame True {
                    }
                    frame False {
                    }
                  }
                  n508 = Not(x=w886) -> (.not. x?=w889:bool)
                  n509 = And(x=w882, y=w889) -> (x .and. y?=w888:bool)
                  n510 = And(x=w889, y=w887) -> (x .and. y?=w885:bool)
                  n511 = Or(x=w888, y=w885) -> (x .or. y?=w884:bool)
                  n512 = case shown="真" w884 {
                    tunnel: w891 -> [_ w917]
                    tunnel: w890 -> [_ w916]
                    tunnel: _ -> [_ w918]
                    frame False {
                    }
                    frame True {
                      w915 = "" ("转换结果")
                      n513 = property on="读版本结果" class="Bool (严格)"("Colors [4]"=w917, "BoolText.Text"=w916) -> ()  [unwired: 2 in, 2 out]
                      n514 = Unbundle(w918) -> (w900, w901, w902, w903, w904, w905, w906, w907)  [unwired: 10 out]
                      n515 = Type Cast(type=w915, x=w906) -> (*(type *) &x=w913:string)
                      n516 = Type Cast(type=w915, x=w903) -> (*(type *) &x=w899:string)
                      n517 = Type Cast(type=w915, x=w900) -> (*(type *) &x=w908:string)
                      n518 = Type Cast(type=w915, x=w904) -> (*(type *) &x=w911:string)
                      n519 = Type Cast(type=w915, x=w905) -> (*(type *) &x=w912:string)
                      n520 = Type Cast(type=w915, x=w901) -> (*(type *) &x=w909:string)
                      n521 = Type Cast(type=w915, x=w902) -> (*(type *) &x=w910:string)
                      n522 = Type Cast(type=w915, x=w907) -> (*(type *) &x=w914:string)
                      n523 = Concatenate Strings(w908, w909, w910, w899, w911, w912, w913, w914) -> (w898:string)
                      n524 = local write "版本号-读"(w898) -> ()
                    }
                  }
                }
                frame Enabled {
                }
              }
            }
          }
          n525 = Or(x=w266, y=TRUE) -> (x .or. y?=w276:bool)
        }
      }
      frame Error {
      }
    }
  }
  n526 = while {
    tunnel: w20 -> [_]
    tunnel: w8 -> [w1037]
    stop <- "停止 2" stop-if-true
    n527 = Dequeue Element(queue=w1037) -> (element=w1035:T1, error out=w1036:errorcluster)  [unwired: 1 in, 3 out]
    n528 = case shown="无错误" w1036 {
      tunnel: w1035 -> [w1041 _]
      frame No Error {
        n529 = Unbundle(w1041) -> ("return type"=w1040:u32, "pReceive"=w1039:T11)
        n530 = for {
          N: w1040 -> [_]
          tunnel: w1039 -> [w1053] mode=indexing
          n531 = Unbundle(w1053) -> ("ID"=w1052:u32, w1051:u8, w1050:u8, w1049:u8, w1048:u8, w1047:u8, w1046:u8, w1043:u8, w1042:u8)  [unwired: 9 out]
          n532 = case shown="4019100" w1052 {
            tunnel: w1051 -> [_ w1066 w1082]
            tunnel: w1050 -> [_ w1065 w1081]
            tunnel: w1049 -> [_ w1064 w1080]
            tunnel: w1048 -> [_ w1063 w1079]
            tunnel: w1047 -> [_ w1062 w1078]
            tunnel: w1046 -> [_ w1061 w1077]
            tunnel: w1043 -> [_ w1057 w1076]
            tunnel: w1042 -> [_ w1056 w1075]
            frame 0, Default {
            }
            frame 67211520 {
              n533 = Join Numbers(hi=w1057, lo=w1056) -> ((hi.lo)=w1055:u16)
              n534 = Join Numbers(hi=w1066, lo=w1065) -> ((hi.lo)=w1070:u16)
              n535 = Join Numbers(hi=w1064, lo=w1063) -> ((hi.lo)=w1069:u16)
              n536 = Join Numbers(hi=w1062, lo=w1061) -> ((hi.lo)=w1068:u16)
              n537 = call "输出分辨率计算.vi"("偏移量"=sgl -3000.0, "分辨率"=0.1, "数值 3"=w1055, "数值 2"=w1069) -> ("输出3"=→"输出3":dbl, "输出2"=→"Curr":dbl)  [unwired: 2 in, 4 out]
              n538 = call "输出分辨率计算.vi"("分辨率"=0.1, "数值 3"=w1068, "数值 2"=w1070) -> ("输出3"=→"SumV_out":dbl, "输出2"=→"SumV_in":dbl)  [unwired: 3 in, 4 out]
            }
            frame 406950144, 408981760, 409112832, 409178368 {
              n539 = Build Array(w1082, w1081, w1080, w1079, w1078, w1077, w1076, w1075) -> (w1074:u8[])
              n540 = global write "EV05全局变量1.vi" "高压校正数组"(w1074) -> ()
              n541 = global write "EV05全局变量1.vi" "高压校正接收"(TRUE ("高压校正接收")) -> ()
            }
          }
          n542 = property on="监控状态" class="Bool (严格)"("Colors [4]"=cluster{u32, u32}[] [{6618880, 6618880}] ("颜色[4]")) -> (error out=w1044:errorcluster)  [unwired: 2 in, 1 out]
          n543 = call <vilib>:"Clear Errors.vi"("error in (no error)"=w1044) -> ()  [unwired: 7 out]
          "接收" <- w1053
        }
      }
      frame Error {
      }
    }
  }
  n544 = while {
    tunnel: w45 -> [w1088]
    tunnel: w44 -> [w1091]
    tunnel: [w1090] -> w32
    tunnel: [w1089] -> w31
    tunnel: w20 -> [_]
    stop <- w1083 stop-if-true
    n545 = local read "版本号"() -> (w1087:string)
    n546 = String Subset(string=w1087, length (rest)=8 ("长度（剩余）")) -> (substring=w1085:string)  [unwired: 1 out]
    n547 = local write "版本号"(w1085) -> ()
    n548 = event shown="[0] \"启动CAN连接\": 值改变" {
      selector: _ -> [_ _ _ _ _ _ _ _ _ _ _ _ _ _ _ _ _ _ _ _ _ _ _ _ _ _ _ _ _ _ _ _ _ _ _ _ _ _ _ _ _ _]
      dyn-events: _ -> [_ _ _ _ _ _ _ _ _ _ _ _ _ _ _ _ _ _ _ _ _ _ _ _ _ _ _ _ _ _ _ _ _ _ _ _ _ _ _ _ _ _]
      timeout: 100 -> [_ _ _ _ _ _ _ _ _ _ _ _ _ _ _ _ _ _ _ _ _ _ _ _ _ _ _ _ _ _ _ _ _ _ _ _ _ _ _ _ _ _]
      tunnel: w1088 -> [w1093 w1123 w1193 _ w1268 _ _ _ _ _ _ w3191 w3230 w3267 w3303 w3325 w3347 w3370 _ _ _ _ w3630 w3647 w3671 w3695 w3728 w3752 w3777 w3802 w3827 w3849 w3871 w3908 w3945 w3984 w4018 _ _ _ _ w4322]
      tunnel: w1091 -> [w1092 w1126 w1198 _ w1270 _ w2778 w2855 _ _ _ w3190 w3229 w3266 w3302 w3324 w3346 w3369 w3461 w3521 _ _ w3629 w3646 w3670 w3694 w3727 w3751 w3776 w3801 w3826 w3848 w3870 w3907 w3944 w3983 w4017 w4046 w4095 w4183 w4271 w4321]
      tunnel: [_ w1122 w1192 _ w1269 _ w2777 w2854 _ _ _ w3189 w3228 w3265 w3301 w3323 w3345 w3368 _ _ _ _ w3628 w3645 w3669 w3693 w3726 w3750 w3775 w3800 w3825 w3847 w3869 w3906 w3943 w3982 w4016 w4045 w4094 w4182 w4272 w4320] -> w1090
      tunnel: [_ w1123 w1193 _ w1267 _ _ _ _ _ _ w3188 w3227 w3264 w3300 w3322 w3344 w3367 _ _ _ _ w3627 w3644 w3668 w3692 w3725 w3749 w3774 w3799 w3824 w3846 w3868 w3905 w3942 w3981 w4015 _ _ _ _ w4319] -> w1089
      tunnel: [_ w1121 w1195 _ _ _ _ _ _ _ _ _ _ _ _ _ _ _ _ _ _ _ _ _ _ _ _ _ _ _ _ _ _ _ _ _ _ _ _ _ _ _] -> w1083
      event "启动CAN连接": Value Change {
        n549 = event-data() -> ("NewVal"=w1094:bool)  [unwired: 6 out]
        n550 = local write "监控"(w1094) -> ()
        n551 = local read "设备索引"() -> (w1099:u16)
        n552 = local read "CAN路数"() -> (w1097:u16)
        n553 = local read "CAN卡类型"() -> (w1100:u32)
        n554 = local read "波特率"() -> (w1098:T3)
        n555 = local read "滤波方式"() -> (w1096:u8)
        n556 = local read "工作方式"() -> (w1095:u8)
        n557 = case shown="真" w1094 {
          tunnel: w1100 -> [w1111 w1120]
          tunnel: w1099 -> [w1110 w1119]
          tunnel: w1098 -> [w1109 w1118]
          tunnel: w1097 -> [w1108 w1117]
          tunnel: w1096 -> [w1106 w1115]
          tunnel: w1095 -> [w1105 w1114]
          tunnel: w1093 -> [w1102 _]
          tunnel: w1092 -> [w1101 _]
          frame True {
            w1103 = u8 0 ("禁用")
            n558 = Flush Queue(queue=w1102, error in (no error)=w1101) -> ()  [unwired: 3 out]
            n559 = call "CAN_Init - EU.vi"("设备类型"=w1111, "设备索引"=w1110, "波特率"=w1109, "CAN路数"=w1108, "操作类型"=enum16{"初始化CAN", "关闭CAN"}."初始化CAN", "滤波方式"=w1106, "工作方式"=w1105) -> ("CAN 操作结果"=w1104:bool)  [unwired: 11 in, 1 out]
            n560 = local write "CAN连接状态"(w1104) -> ()
            n561 = local write "CAN状态"(w1104) -> ()
            n562 = property on="Set_out" class="Bool (严格)"("Disabled"=w1103) -> ()  [unwired: 2 in, 2 out]
            n563 = property on="Clear_in" class="Bool (严格)"("Disabled"=w1103) -> ()  [unwired: 2 in, 2 out]
            n564 = property on="Set_in" class="Bool (严格)"("Disabled"=w1103) -> ()  [unwired: 2 in, 2 out]
            n565 = property on="Read2_Out" class="Bool (严格)"("Disabled"=w1103) -> ()  [unwired: 2 in, 2 out]
            n566 = property on="Clear" class="Bool (严格)"("Disabled"=w1103) -> ()  [unwired: 2 in, 2 out]
            n567 = property on="Read1_Out" class="Bool (严格)"("Disabled"=w1103) -> ()  [unwired: 2 in, 2 out]
            n568 = property on="Set Current Gain" class="Bool (严格)"("Disabled"=w1103) -> ()  [unwired: 2 in, 2 out]
            n569 = property on="Set Current Offset" class="Bool (严格)"("Disabled"=w1103) -> ()  [unwired: 2 in, 2 out]
            n570 = property on="Read1_in" class="Bool (严格)"("Disabled"=w1103) -> ()  [unwired: 2 in, 2 out]
            n571 = property on="Clear_out" class="Bool (严格)"("Disabled"=w1103) -> ()  [unwired: 2 in, 2 out]
            n572 = property on="Read2_in" class="Bool (严格)"("Disabled"=w1103) -> ()  [unwired: 2 in, 2 out]
            n573 = property on="Set" class="Bool (严格)"("Disabled"=w1103) -> ()  [unwired: 2 in, 2 out]
            n574 = property on="Read2" class="Bool (严格)"("Disabled"=w1103) -> ()  [unwired: 2 in, 2 out]
            n575 = property on="Read1" class="Bool (严格)"("Disabled"=w1103) -> ()  [unwired: 2 in, 2 out]
          }
          frame False {
            w1112 = u8 0 ("禁用")
            w1113 = FALSE ("CAN状态")
            n576 = call "CAN_Init.vi"("设备类型"=w1120, "设备索引"=w1119, "波特率"=w1118, "CAN路数"=w1117, "操作类型"=enum16{"初始化CAN", "关闭CAN"}."关闭CAN", "滤波方式"=w1115, "工作方式"=w1114) -> ()  [unwired: 3 in, 10 out]
            n577 = invoke on="监控" class="Bool" method="Reinit To Default"() -> ()  [unwired: 3 in, 3 out]
            n578 = local write "CAN连接状态"(w1113) -> ()
            n579 = local write "CAN状态"(w1113) -> ()
            n580 = property on="Set_out" class="Bool (严格)"("Disabled"=w1112) -> ()  [unwired: 2 in, 2 out]
            n581 = property on="Clear_in" class="Bool (严格)"("Disabled"=w1112) -> ()  [unwired: 2 in, 2 out]
            n582 = property on="Set_in" class="Bool (严格)"("Disabled"=w1112) -> ()  [unwired: 2 in, 2 out]
            n583 = property on="Read2_Out" class="Bool (严格)"("Disabled"=w1112) -> ()  [unwired: 2 in, 2 out]
            n584 = property on="Clear" class="Bool (严格)"("Disabled"=w1112) -> ()  [unwired: 2 in, 2 out]
            n585 = property on="Read1_Out" class="Bool (严格)"("Disabled"=w1112) -> ()  [unwired: 2 in, 2 out]
            n586 = property on="Set Current Gain" class="Bool (严格)"("Disabled"=w1112) -> ()  [unwired: 2 in, 2 out]
            n587 = property on="Set Current Offset" class="Bool (严格)"("Disabled"=w1112) -> ()  [unwired: 2 in, 2 out]
            n588 = property on="Read1_in" class="Bool (严格)"("Disabled"=w1112) -> ()  [unwired: 2 in, 2 out]
            n589 = property on="Clear_out" class="Bool (严格)"("Disabled"=w1112) -> ()  [unwired: 2 in, 2 out]
            n590 = property on="Read2_in" class="Bool (严格)"("Disabled"=w1112) -> ()  [unwired: 2 in, 2 out]
            n591 = property on="Set" class="Bool (严格)"("Disabled"=w1112) -> ()  [unwired: 2 in, 2 out]
            n592 = property on="Read2" class="Bool (严格)"("Disabled"=w1112) -> ()  [unwired: 2 in, 2 out]
            n593 = property on="Read1" class="Bool (严格)"("Disabled"=w1112) -> ()  [unwired: 2 in, 2 out]
          }
        }
      }
      event "退出": Value Change {
        n594 = event-data() -> ()  [unwired: 7 out]
        n595 = flat-sequence {
          tunnel: w1126 -> [w1129]
          tunnel: [w1132] -> w1125
          tunnel: [w1131] -> w1124
          tunnel: [w1130] -> w1121
          tunnel: w1125 -> [_]
          tunnel: w1124 -> [w1191]
          tunnel: [w1191] -> w1122
          frame #0 {
            w1130 = TRUE ("停止")
            n596 = disable-structure shown="禁用" {
              frame Disabled {
                n597 = local read "CAN卡类型"() -> (w1149:u32)
                n598 = local read "设备索引"() -> (w1148:u16)
                n599 = call "CAN_Init.vi"("设备类型"=w1149, "设备索引"=w1148, "操作类型"=enum16{"初始化CAN", "关闭CAN"}."关闭CAN") -> ()  [unwired: 7 in, 10 out]
              }
              frame Enabled {
              }
            }
            n600 = local write "停止"(w1130) -> ()
            n601 = local write "停止 3"(w1130) -> ()
            n602 = local write "停止 2"(w1130) -> ()
            n603 = local write "停止 6"(w1130) -> ()
            n604 = local write "停止 7"(w1130) -> ()
            n605 = local read "VISA资源名称输出 10"() -> (w1135:refnum<visa-resource-name>)
            n606 = local read "VISA资源名称输出"() -> (w1140:refnum<visa-resource-name>)
            n607 = flat-sequence {
              tunnel: w1135 -> [w1154]
              tunnel: [w1154] -> w1139
              tunnel: w1129 -> [w1152]
              tunnel: [w1151] -> w1127
              tunnel: w1139 -> [w1157]
              tunnel: [w1157] -> w1138
              tunnel: [w1155] -> w1128
              tunnel: w1127 -> [w1155]
              tunnel: w1138 -> [w1161]
              tunnel: [w1160] -> w1137
              tunnel: [w1159] -> w1136
              tunnel: w1128 -> [w1158]
              tunnel: [w1164] -> w1133
              tunnel: [w1165] -> w1134
              tunnel: w1137 -> [w1165]
              tunnel: w1136 -> [w1164]
              frame #0 {
                n608 = VISA Write(VISA resource name=w1154, write buffer="OUT:OFF" ("写入缓冲区"), error in (no error)=w1152) -> (error out=w1151:errorcluster)  [unwired: 2 out]
              }
              frame #1 {
                n609 = Wait (ms)(milliseconds to wait=u32 50 ("等待时间（毫秒）")) -> ()  [unwired: 1 out]
              }
              frame #2 {
                n610 = VISA Write(VISA resource name=w1161, write buffer="OUT:OFF" ("写入缓冲区"), error in (no error)=w1158) -> (VISA resource name out=w1160:refnum<visa-resource-name>, error out=w1159:errorcluster)  [unwired: 1 out]
              }
              frame #3 {
                n611 = Wait (ms)(milliseconds to wait=u32 50 ("等待时间（毫秒）")) -> ()  [unwired: 1 out]
              }
            }
            n612 = flat-sequence {
              tunnel: w1140 -> [w1166]
              tunnel: [w1166] -> w1147
              tunnel: w1147 -> [w1168]
              tunnel: [w1168] -> w1146
              tunnel: w1146 -> [w1173]
              tunnel: [w1172] -> w1145
              tunnel: [w1171] -> w1144
              tunnel: [w1170] -> w1143
              tunnel: w1129 -> [w1169]
              tunnel: [w1176] -> w1142
              tunnel: [w1175] -> w1141
              tunnel: w1145 -> [w1178]
              tunnel: w1144 -> [w1177]
              tunnel: w1143 -> [w1174]
              frame #0 {
              }
              frame #1 {
                n613 = Wait (ms)(milliseconds to wait=u32 50 ("等待时间（毫秒）")) -> ()  [unwired: 1 out]
              }
              frame #2 {
                w1170 = "outp off" ("写入缓冲区")
                n614 = VISA Write(VISA resource name=w1173, write buffer=w1170, error in (no error)=w1169) -> (VISA resource name out=w1172:refnum<visa-resource-name>, error out=w1171:errorcluster)  [unwired: 1 out]
              }
              frame #3 {
                n615 = VISA Write(VISA resource name=w1178, write buffer=w1174, error in (no error)=w1177) -> (VISA resource name out=w1175:refnum<visa-resource-name>, error out=w1176:errorcluster)  [unwired: 1 out]
                n616 = Wait (ms)(milliseconds to wait=u32 50 ("等待时间（毫秒）")) -> ()  [unwired: 1 out]
              }
            }
            n617 = VISA Close(VISA resource name=w1141, error in (no error)=w1142) -> (error out=w1132:errorcluster)
            n618 = VISA Close(VISA resource name=w1134, error in (no error)=w1133) -> (error out=w1131:errorcluster)
          }
          frame #1 {
            n619 = global read "EV05全局变量1.vi" "设备索引号"() -> (w1186:u16)
            n620 = global read "EV05全局变量1.vi" "CAN卡类型"() -> (w1187:u32)
            n621 = global read "EV05全局变量1.vi" "CAN端口"() -> (w1185:u16)
            n622 = property class="VI"("FP.State"=T12."Hidden" ("前面板窗口:状态")) -> (reference out=w1183:refnum<vi>, error out=w1184:errorcluster)  [unwired: 2 in]
            n623 = Build Array(7) -> (w1188:i32[])
            n624 = call "transmit-8.6.vi"("can卡类型"=w1187, "设备索引号"=w1186, "CAN端口"=w1185, "ID"=418398080, "SendType"=u8 0, "Data"=w1188) -> ()  [unwired: 3 in, 11 out]
            n625 = property class="VI"(reference=w1183, error in=w1184, "Front Panel.Open"=FALSE ("前面板窗口:打开")) -> ()  [unwired: 2 out]
          }
        }
      }
      event Panel Close? {
        n626 = event-data() -> ()  [unwired: 5 out]
        n627 = flat-sequence {
          tunnel: w1198 -> [w1201]
          tunnel: [w1200] -> w1197
          tunnel: [w1199] -> w1196
          tunnel: w1197 -> [_]
          tunnel: w1196 -> [w1254]
          tunnel: [w1254] -> w1192
          tunnel: [w1253] -> w1195
          frame #0 {
            n628 = local read "VISA资源名称输出 10"() -> (w1204:refnum<visa-resource-name>)
            n629 = local read "VISA资源名称输出"() -> (w1209:refnum<visa-resource-name>)
            n630 = flat-sequence {
              tunnel: w1204 -> [w1217]
              tunnel: [w1217] -> w1208
              tunnel: w1208 -> [w1219]
              tunnel: [w1219] -> w1207
              tunnel: w1207 -> [w1223]
              tunnel: [w1222] -> w1206
              tunnel: [w1221] -> w1205
              tunnel: w1201 -> [w1220]
              tunnel: [w1226] -> w1202
              tunnel: [w1227] -> w1203
              tunnel: w1206 -> [w1227]
              tunnel: w1205 -> [w1226]
              frame #0 {
              }
              frame #1 {
                n631 = Wait (ms)(milliseconds to wait=u32 120 ("等待时间（毫秒）")) -> ()  [unwired: 1 out]
              }
              frame #2 {
                n632 = VISA Write(VISA resource name=w1223, write buffer="OUT:OFF" ("写入缓冲区"), error in (no error)=w1220) -> (VISA resource name out=w1222:refnum<visa-resource-name>, error out=w1221:errorcluster)  [unwired: 1 out]
              }
              frame #3 {
                n633 = Wait (ms)(milliseconds to wait=u32 50 ("等待时间（毫秒）")) -> ()  [unwired: 1 out]
              }
            }
            n634 = flat-sequence {
              tunnel: w1209 -> [w1228]
              tunnel: [w1228] -> w1216
              tunnel: w1216 -> [w1230]
              tunnel: [w1230] -> w1215
              tunnel: w1215 -> [w1235]
              tunnel: [w1234] -> w1214
              tunnel: [w1233] -> w1213
              tunnel: [w1232] -> w1212
              tunnel: w1201 -> [w1231]
              tunnel: [w1238] -> w1211
              tunnel: [w1237] -> w1210
              tunnel: w1214 -> [w1240]
              tunnel: w1213 -> [w1239]
              tunnel: w1212 -> [w1236]
              frame #0 {
              }
              frame #1 {
                n635 = Wait (ms)(milliseconds to wait=u32 120 ("等待时间（毫秒）")) -> ()  [unwired: 1 out]
              }
              frame #2 {
                w1232 = "outp off" ("写入缓冲区")
                n636 = VISA Write(VISA resource name=w1235, write buffer=w1232, error in (no error)=w1231) -> (VISA resource name out=w1234:refnum<visa-resource-name>, error out=w1233:errorcluster)  [unwired: 1 out]
              }
              frame #3 {
                n637 = VISA Write(VISA resource name=w1240, write buffer=w1236, error in (no error)=w1239) -> (VISA resource name out=w1237:refnum<visa-resource-name>, error out=w1238:errorcluster)  [unwired: 1 out]
                n638 = Wait (ms)(milliseconds to wait=u32 50 ("等待时间（毫秒）")) -> ()  [unwired: 1 out]
              }
            }
            n639 = VISA Close(VISA resource name=w1210, error in (no error)=w1211) -> (error out=w1200:errorcluster)
            n640 = VISA Close(VISA resource name=w1203, error in (no error)=w1202) -> (error out=w1199:errorcluster)
          }
          frame #1 {
            w1253 = TRUE ("停止")
            n641 = global read "EV05全局变量1.vi" "设备索引号"() -> (w1248:u16)
            n642 = global read "EV05全局变量1.vi" "CAN卡类型"() -> (w1249:u32)
            n643 = global read "EV05全局变量1.vi" "CAN端口"() -> (w1247:u16)
            n644 = property class="VI"("FP.State"=T12."Hidden" ("前面板窗口:状态")) -> (reference out=w1245:refnum<vi>, error out=w1246:errorcluster)  [unwired: 2 in]
            n645 = Build Array(7) -> (w1250:i32[])
            n646 = local write "停止"(w1253) -> ()
            n647 = call "transmit-8.6.vi"("can卡类型"=w1249, "设备索引号"=w1248, "CAN端口"=w1247, "ID"=418398080, "SendType"=u8 0, "Data"=w1250) -> ()  [unwired: 3 in, 11 out]
            n648 = local write "停止 3"(w1253) -> ()
            n649 = local write "停止 2"(w1253) -> ()
            n650 = local write "停止 6"(w1253) -> ()
            n651 = local write "停止 7"(w1253) -> ()
            n652 = property class="VI"(reference=w1245, error in=w1246, "Front Panel.Open"=FALSE ("前面板窗口:打开")) -> ()  [unwired: 2 out]
          }
        }
        n653 = event-data("Discard?"=FALSE ("放弃？")) -> ()  [unwired: 1 in, 1 out]
      }
      event "刷新": Value Change {
        n654 = event-data() -> ("NewVal"=w1255:bool)  [unwired: 6 out]
        n655 = case shown="真" w1255 {
          frame False {
          }
          frame True {
            w1261 = cluster{u32, u32}[] [{0, 0}] ("颜色[4]")
            w1260 = "" ("布尔文本.文本")
            n656 = property on="Set结果" class="Bool (严格)"("Colors [4]"=w1261, "BoolText.Text"=w1260) -> ()  [unwired: 2 in, 2 out]
            n657 = property on="Read1结果" class="Bool (严格)"("Colors [4]"=w1261, "BoolText.Text"=w1260) -> ()  [unwired: 2 in, 2 out]
            n658 = property on="Clear_in结果" class="Bool (严格)"("Colors [4]"=w1261, "BoolText.Text"=w1260) -> ()  [unwired: 2 in, 2 out]
            n659 = property on="Current Offset结果 2" class="Bool (严格)"("Colors [4]"=w1261, "BoolText.Text"=w1260) -> ()  [unwired: 2 in, 2 out]
            n660 = property on="Current Offset结果 4" class="Bool (严格)"("Colors [4]"=w1261, "BoolText.Text"=w1260) -> ()  [unwired: 2 in, 2 out]
            n661 = property on="Current Gain结果 4" class="Bool (严格)"("Colors [4]"=w1261, "BoolText.Text"=w1260) -> ()  [unwired: 2 in, 2 out]
            n662 = property on="Set_out结果" class="Bool (严格)"("Colors [4]"=w1261, "BoolText.Text"=w1260) -> ()  [unwired: 2 in, 2 out]
            n663 = property on="Read2_Out结果" class="Bool (严格)"("Colors [4]"=w1261, "BoolText.Text"=w1260) -> ()  [unwired: 2 in, 2 out]
            n664 = property on="Read1_Out结果" class="Bool (严格)"("Colors [4]"=w1261, "BoolText.Text"=w1260) -> ()  [unwired: 2 in, 2 out]
            n665 = property on="Current Offset结果" class="Bool (严格)"("Colors [4]"=w1261, "BoolText.Text"=w1260) -> ()  [unwired: 2 in, 2 out]
            n666 = property on="Current Offset结果 3" class="Bool (严格)"("Colors [4]"=w1261, "BoolText.Text"=w1260) -> ()  [unwired: 2 in, 2 out]
            n667 = property on="Current Gain结果 3" class="Bool (严格)"("Colors [4]"=w1261, "BoolText.Text"=w1260) -> ()  [unwired: 2 in, 2 out]
            n668 = property on="Read2结果" class="Bool (严格)"("Colors [4]"=w1261, "BoolText.Text"=w1260) -> ()  [unwired: 2 in, 2 out]
            n669 = property on="Current Offset结果" class="Bool (严格)"("Colors [4]"=w1261, "BoolText.Text"=w1260) -> ()  [unwired: 2 in, 2 out]
            n670 = property on="Current Gain结果" class="Bool (严格)"("Colors [4]"=w1261, "BoolText.Text"=w1260) -> ()  [unwired: 2 in, 2 out]
            n671 = property on="Clear结果" class="Bool (严格)"("Colors [4]"=w1261, "BoolText.Text"=w1260) -> ()  [unwired: 2 in, 2 out]
            n672 = property on="Read1_in结果" class="Bool (严格)"("Colors [4]"=w1261, "BoolText.Text"=w1260) -> ()  [unwired: 2 in, 2 out]
            n673 = property on="Clear_out结果" class="Bool (严格)"("Colors [4]"=w1261, "BoolText.Text"=w1260) -> ()  [unwired: 2 in, 2 out]
            n674 = property on="Read2_in结果" class="Bool (严格)"("Colors [4]"=w1261, "BoolText.Text"=w1260) -> ()  [unwired: 2 in, 2 out]
            n675 = property on="Set_in结果" class="Bool (严格)"("Colors [4]"=w1261, "BoolText.Text"=w1260) -> ()  [unwired: 2 in, 2 out]
            n676 = property on="Current Gain结果 2" class="Bool (严格)"("Colors [4]"=w1261, "BoolText.Text"=w1260) -> ()  [unwired: 2 in, 2 out]
            n677 = control-ref of="结果"() -> (w1258:refnum<vi>)
            n678 = for {
              N: 40 -> [_]
              tunnel: w1258 -> [w1266]
              i -> [w1264]
              n679 = Bundle(w1264, 0) -> (w1262:cluster{i32, i32})  [unwired: 1 out]
              n680 = property class="MCListbox (严格)"(reference=w1266, "ActiveCell"=w1262, "CellBG"=u32 16448250) -> ()  [unwired: 1 in, 2 out]
            }
            n681 = property class="MCListbox (严格)"(reference=w1258, "ItemNames"=string[][] [] ("项名")) -> ()  [unwired: 1 in, 2 out]
            n682 = local write "分流器大小"(T2."选择分流器型号" ("Shunt Type")) -> ()
          }
        }
      }
      event "一键校正": Value Change {
        n683 = event-data() -> ("NewVal"=w1271:bool)  [unwired: 6 out]
        n684 = case shown="真" w1271 {
          tunnel: w1270 -> [w1273 w1277]
          tunnel: [w1273 w1276] -> w1269
          tunnel: w1268 -> [w1272 w1275]
          tunnel: [w1272 w1274] -> w1267
          frame False {
          }
          frame True {
            n685 = while {
              tunnel: w1277 -> [w1286]
              tunnel: [w1283] -> w1276
              tunnel: w1275 -> [w1285]
              tunnel: [w1284] -> w1274
              i -> [w1287]
              stop <- w1282 continue-if-true
              n686 = case shown="0, 默认" w1287 {
                tunnel: w1286 -> [w1300 w1327 w1363 w1435 w1471 w1544 w1584 w1624 w1666 w1737 w1779 w1842 w1932 w1971 w1995 w2080 w2126 w2169 w2254 w2300 w2344 w2389 w2447 w2594 w2626]
                tunnel: [w1292 w1320 w1361 w1428 w1469 w1537 w1577 w1619 w1663 w1732 w1772 w1840 TRUE ("status") w1968 w1991 w2075 w2121 w2166 w2249 w2295 w2339 w2384 w2444 w2590 w2623] -> w1282
                tunnel: w1285 -> [w1297 w1328 w1360 w1436 w1468 w1545 w1585 w1625 w1665 w1738 w1780 w1839 w1931 w1967 w1994 w2081 w2127 w2168 w2255 w2301 w2345 w2390 w2446 w2592 w2627]
                tunnel: [w1297 w1326 w1360 w1434 w1468 w1543 w1583 w1627 w1665 w1740 w1778 w1839 w1931 w1967 w1994 w2079 w2125 w2168 w2253 w2299 w2343 w2388 w2446 w2592 w2625] -> w1284
                tunnel: [w1299 w1325 w1362 w1433 w1470 w1542 w1582 w1626 w1664 w1739 w1777 w1841 w1930 w1970 w1993 w2078 w2124 w2167 w2252 w2298 w2342 w2387 w2445 w2593 w2624] -> w1283
                frame 0, Default {
                  # "打开电流源"
                  n687 = local read "VISA resource name 2"() -> (w1307:refnum<visa-resource-name>)
                  n688 = VISA Open(error in (no error)=w1300, VISA resource name=w1307) -> (VISA resource name=w1302:refnum<visa-resource-name>, error out=w1305:errorcluster)  [unwired: 3 out]
                  n689 = property class="Instr"(reference=w1302, "Timeout"=u32 100 ("General Settings:Timeout Value")) -> (reference out=w1301:refnum<visa-resource-name>)  [unwired: 1 in, 1 out]
                  n690 = VISA Write(VISA resource name=w1301, write buffer="*rst" ("写入缓冲区"), error in (no error)=w1305) -> (VISA resource name out=w1304:refnum<visa-resource-name>, error out=w1299:errorcluster)  [unwired: 1 out]
                  n691 = Unbundle(w1299) -> ("status"=w1298:bool)  [unwired: 2 out]
                  n692 = case shown="假" w1298 {
                    tunnel: w1304 -> [w1313 w1318]
                    tunnel: ["电流源连接成功" "电流源连接NG"] -> w1294
                    tunnel: [u32 6618880 u32 16711680] -> w1295
                    frame False {
                      w1311 = u8 0 ("禁用")
                      n693 = local write "VISA资源名称输出"(w1313) -> ()
                      n694 = local write "连接状态 10"(TRUE ("连接状态")) -> ()
                      n695 = property on="连接状态 10" class="Bool (严格)"("Colors [4]"=cluster{u32, u32}[] [{6618880, 6618880}] ("颜色[4]")) -> ()  [unwired: 2 in, 2 out]
                      n696 = property on="输出100A" class="Bool"("Disabled"=w1311) -> ()  [unwired: 2 in, 2 out]
                      n697 = property on="输出200A" class="Bool"("Disabled"=w1311) -> ()  [unwired: 2 in, 2 out]
                      n698 = property on="输出自定义值2 2" class="Bool"("Disabled"=w1311) -> ()  [unwired: 2 in, 2 out]
                      n699 = property on="输出自定义值1 2" class="Bool"("Disabled"=w1311) -> ()  [unwired: 2 in, 2 out]
                    }
                    frame True {
                      w1317 = u8 2 ("禁用")
                      n700 = local write "VISA资源名称输出"(w1318) -> ()
                      n701 = local write "连接状态 10"(FALSE ("连接状态")) -> ()
                      n702 = property on="连接状态 10" class="Bool (严格)"("Colors [4]"=cluster{u32, u32}[] [{15663131, 6618880}] ("颜色[4]")) -> ()  [unwired: 2 in, 2 out]
                      n703 = property on="输出100A" class="Bool"("Disabled"=w1317) -> ()  [unwired: 2 in, 2 out]
                      n704 = property on="输出200A" class="Bool"("Disabled"=w1317) -> ()  [unwired: 2 in, 2 out]
                      n705 = property on="输出自定义值2 2" class="Bool"("Disabled"=w1317) -> ()  [unwired: 2 in, 2 out]
                      n706 = property on="输出自定义值1 2" class="Bool"("Disabled"=w1317) -> ()  [unwired: 2 in, 2 out]
                    }
                  }
                  n707 = control-ref of="结果"() -> (w1296:refnum<vi>)
                  n708 = Build Array(w1294) -> (w1293:string[])
                  n709 = call "表格编辑.vi"("新元素/子数组"=w1293, "活动单元格:单元格背景色"=w1295, "MCListbox引用句柄"=w1296) -> ()  [unwired: 9 out]
                  n710 = Not(x=w1298) -> (.not. x?=w1292:bool)
                }
                frame 1 {
                  # "5460电流零点"
                  n711 = flat-sequence {
                    tunnel: w1327 -> [w1334]
                    tunnel: w1328 -> [w1335]
                    tunnel: [w1335] -> w1324
                    tunnel: [w1334] -> w1323
                    tunnel: w1324 -> [w1339]
                    tunnel: w1323 -> [w1338]
                    tunnel: [w1337] -> w1322
                    tunnel: [w1336] -> w1321
                    tunnel: [w1346] -> w1325
                    tunnel: [w1347] -> w1326
                    tunnel: w1322 -> [w1347]
                    tunnel: w1321 -> [w1346]
                    tunnel: [w1341] -> w1320
                    frame #0 {
                      n712 = local write "电流零点"("" ("5460Current Offset")) -> ()
                      n713 = global write "EV05全局变量1.vi" "高压校正接收"(FALSE ("高压校正接收")) -> ()
                      n714 = global write "EV05全局变量1.vi" "CAN接收"(FALSE ("CAN接收")) -> ()
                      n715 = call <vilib>:"Set Busy.vi"() -> ()  [unwired: 4 in, 8 out]
                      n716 = property on="Current Offset结果" class="Bool (严格)"("Colors [4]"=cluster{u32, u32}[] [{0, 0}] ("颜色[4]"), "BoolText.Text"="" ("布尔文本.文本")) -> ()  [unwired: 2 in, 2 out]
                    }
                    frame #1 {
                      n717 = Enqueue Element(queue=w1339, element="Set Current Offset" ("元素"), error in (no error)=w1338) -> (queue out=w1337:refnum<queue>, error out=w1336:errorcluster)  [unwired: 2 out]
                    }
                    frame #2 {
                      n718 = while {
                        tunnel: [w1353] -> w1341
                        i -> [w1358]
                        stop <- w1354 stop-if-true
                        n719 = property on="Current Offset结果" class="Bool (严格)"() -> ("BoolText.Text"=w1352:string)  [unwired: 2 in, 2 out]
                        n720 = Greater Or Equal?(x=w1358, y=30) -> (x >= y?=w1355:bool)
                        n721 = Not Equal?(x=w1352, y="NG" ("布尔文本.文本")) -> (x != y?=w1353:bool)
                        n722 = Wait Until Next ms Multiple(millisecond multiple=u32 110 ("毫秒倍数")) -> ()  [unwired: 1 out]
                        n723 = Or(x=w1353, y=w1355) -> (x .or. y?=w1354:bool)
                      }
                      n724 = case shown="真" w1341 {
                        tunnel: ["5460电流零点校正NG" "5460电流零点校正成功"] -> w1342
                        tunnel: [u32 16711680 u32 6618880] -> w1343
                        frame False {
                        }
                        frame True {
                        }
                      }
                      n725 = control-ref of="结果"() -> (w1344:refnum<vi>)
                      n726 = Build Array(w1342) -> (w1345:string[])
                      n727 = call "表格编辑.vi"("新元素/子数组"=w1345, "活动单元格:单元格背景色"=w1343, "MCListbox引用句柄"=w1344) -> ()  [unwired: 9 out]
                    }
                  }
                }
                frame 2 {
                  # "300A"
                  n728 = flat-sequence {
                    tunnel: FALSE ("控制读取") -> [w1376]
                    tunnel: [w1386] -> w1375
                    tunnel: [w1385] -> w1374
                    tunnel: [w1380] -> w1373
                    tunnel: w1363 -> [w1379]
                    tunnel: w1375 -> [w1390]
                    tunnel: [w1390] -> w1372
                    tunnel: w1374 -> [w1389]
                    tunnel: [w1389] -> w1371
                    tunnel: [w1387] -> w1370
                    tunnel: w1373 -> [w1387]
                    tunnel: w1372 -> [w1395]
                    tunnel: w1371 -> [w1394]
                    tunnel: [w1393] -> w1369
                    tunnel: [w1392] -> w1368
                    tunnel: w1370 -> [w1391]
                    tunnel: w1369 -> [w1398]
                    tunnel: [w1398] -> w1367
                    tunnel: w1368 -> [w1397]
                    tunnel: [w1397] -> w1366
                    tunnel: w1367 -> [w1402]
                    tunnel: w1366 -> [w1401]
                    tunnel: [w1399] -> w1365
                    tunnel: w1365 -> [w1410]
                    tunnel: [w1410] -> w1362
                    tunnel: [w1409] -> w1361
                    frame #0 {
                      n729 = local write "控制读取  2"(w1376) -> ()
                    }
                    frame #1 {
                      n730 = Wait (ms)(milliseconds to wait=u32 50 ("等待时间（毫秒）")) -> ()  [unwired: 1 out]
                    }
                    frame #2 {
                      n731 = local read "VISA资源名称输出"() -> (w1384:refnum<visa-resource-name>)
                      n732 = Number To Fractional String(number=300.0 ("数字"), precision (6)=i16 3 ("精度(6)")) -> (F-format string=w1381:string)  [unwired: 2 out]
                      n733 = Concatenate Strings("volt 1;curr " ("写入缓冲区"), w1381) -> (w1380:string)
                      n734 = VISA Write(VISA resource name=w1384, write buffer=w1380, error in (no error)=w1379) -> (VISA resource name out=w1386:refnum<visa-resource-name>, error out=w1385:errorcluster)  [unwired: 1 out]
                    }
                    frame #3 {
                      n735 = Wait (ms)(milliseconds to wait=u32 50 ("等待时间（毫秒）")) -> ()  [unwired: 1 out]
                    }
                    frame #4 {
                      n736 = VISA Write(VISA resource name=w1395, write buffer=w1391, error in (no error)=w1394) -> (VISA resource name out=w1393:refnum<visa-resource-name>, error out=w1392:errorcluster)  [unwired: 1 out]
                    }
                    frame #5 {
                      n737 = Wait (ms)(milliseconds to wait=u32 200 ("等待时间（毫秒）")) -> ()  [unwired: 1 out]
                    }
                    frame #6 {
                      n738 = Wait (ms)(milliseconds to wait=u32 50 ("等待时间（毫秒）")) -> ()  [unwired: 1 out]
                      n739 = VISA Write(VISA resource name=w1402, write buffer="outp on" ("写入缓冲区"), error in (no error)=w1401) -> (VISA resource name out=w1404:refnum<visa-resource-name>, error out=w1399:errorcluster)  [unwired: 1 out]
                      n740 = local write "VISA资源名称输出"(w1404) -> ()
                    }
                    frame #7 {
                      n741 = while {
                        tunnel: [w1413] -> w1409
                        i -> [w1416]
                        stop <- w1412 stop-if-true
                        w1418 = 300.0 ("x")
                        n742 = local read "Actual"() -> (w1422:dbl)
                        n743 = Greater Or Equal?(x=w1416, y=20) -> (x >= y?=w1414:bool)
                        n744 = Multiply(x=w1418, y=0.02) -> (x*y=w1419:dbl)
                        n745 = Add(x=w1418, y=w1419) -> (x+y=w1421:dbl)
                        n746 = Subtract(x=w1418, y=w1419) -> (x-y=w1420:dbl)
                        n747 = Wait Until Next ms Multiple(millisecond multiple=u32 200 ("毫秒倍数")) -> ()  [unwired: 1 out]
                        n748 = In Range and Coerce(upper limit=w1421, x=w1422, lower limit=w1420) -> (In Range?=w1413:bool)  [unwired: 1 out]
                        n749 = Or(x=w1413, y=w1414) -> (x .or. y?=w1412:bool)
                      }
                      n750 = local write "控制读取  2"(TRUE ("控制读取")) -> ()
                      n751 = case shown="假" w1409 {
                        tunnel: ["300A电流开启NG" "300A电流开启成功"] -> w1405
                        tunnel: [u32 16711680 u32 6618880] -> w1406
                        frame False {
                        }
                        frame True {
                        }
                      }
                      n752 = control-ref of="结果"() -> (w1407:refnum<vi>)
                      n753 = Build Array(w1405) -> (w1408:string[])
                      n754 = call "表格编辑.vi"("新元素/子数组"=w1408, "活动单元格:单元格背景色"=w1406, "MCListbox引用句柄"=w1407) -> ()  [unwired: 9 out]
                    }
                  }
                }
                frame 3 {
                  # "5460电流增益"
                  n755 = flat-sequence {
                    tunnel: w1435 -> [w1442]
                    tunnel: w1436 -> [w1443]
                    tunnel: [w1443] -> w1432
                    tunnel: [w1442] -> w1431
                    tunnel: w1432 -> [w1447]
                    tunnel: w1431 -> [w1446]
                    tunnel: [w1445] -> w1430
                    tunnel: [w1444] -> w1429
                    tunnel: [w1454] -> w1433
                    tunnel: [w1455] -> w1434
                    tunnel: w1430 -> [w1455]
                    tunnel: w1429 -> [w1454]
                    tunnel: [w1449] -> w1428
                    frame #0 {
                      n756 = global write "EV05全局变量1.vi" "高压校正接收"(FALSE ("高压校正接收")) -> ()
                      n757 = local write "电流增益"("" ("5460Current Offset")) -> ()
                      n758 = global write "EV05全局变量1.vi" "CAN接收"(FALSE ("CAN接收")) -> ()
                      n759 = call <vilib>:"Set Busy.vi"() -> ()  [unwired: 4 in, 8 out]
                      n760 = property on="Current Gain结果" class="Bool (严格)"("Colors [4]"=cluster{u32, u32}[] [{0, 0}] ("颜色[4]"), "BoolText.Text"="" ("布尔文本.文本")) -> ()  [unwired: 2 in, 2 out]
                    }
                    frame #1 {
                      n761 = Enqueue Element(queue=w1447, element="Set Current Gain" ("元素"), error in (no error)=w1446) -> (queue out=w1445:refnum<queue>, error out=w1444:errorcluster)  [unwired: 2 out]
                    }
                    frame #2 {
                      n762 = while {
                        tunnel: [w1461] -> w1449
                        i -> [w1466]
                        stop <- w1462 stop-if-true
                        n763 = property on="Current Gain结果" class="Bool (严格)"() -> ("BoolText.Text"=w1460:string)  [unwired: 2 in, 2 out]
                        n764 = Greater Or Equal?(x=w1466, y=30) -> (x >= y?=w1463:bool)
                        n765 = Not Equal?(x=w1460, y="NG" ("布尔文本.文本")) -> (x != y?=w1461:bool)
                        n766 = Wait Until Next ms Multiple(millisecond multiple=u32 110 ("毫秒倍数")) -> ()  [unwired: 1 out]
                        n767 = Or(x=w1461, y=w1463) -> (x .or. y?=w1462:bool)
                      }
                      n768 = case shown="假" w1449 {
                        tunnel: ["5460电流增益校正NG" "5460电流增益校正成功"] -> w1450
                        tunnel: [u32 16711680 u32 6618880] -> w1451
                        frame False {
                        }
                        frame True {
                        }
                      }
                      n769 = control-ref of="结果"() -> (w1452:refnum<vi>)
                      n770 = Build Array(w1450) -> (w1453:string[])
                      n771 = call "表格编辑.vi"("新元素/子数组"=w1453, "活动单元格:单元格背景色"=w1451, "MCListbox引用句柄"=w1452) -> ()  [unwired: 9 out]
                    }
                  }
                }
                frame 4 {
                  # "40A"
                  n772 = flat-sequence {
                    tunnel: FALSE ("控制读取") -> [w1485]
                    tunnel: [w1495] -> w1484
                    tunnel: [w1494] -> w1483
                    tunnel: [w1488] -> w1482
                    tunnel: w1471 -> [w1487]
                    tunnel: w1484 -> [w1499]
                    tunnel: [w1499] -> w1481
                    tunnel: w1483 -> [w1498]
                    tunnel: [w1498] -> w1480
                    tunnel: [w1496] -> w1479
                    tunnel: w1482 -> [w1496]
                    tunnel: w1481 -> [w1504]
                    tunnel: w1480 -> [w1503]
                    tunnel: [w1502] -> w1478
                    tunnel: [w1501] -> w1477
                    tunnel: w1479 -> [w1500]
                    tunnel: w1478 -> [w1507]
                    tunnel: [w1507] -> w1476
                    tunnel: w1477 -> [w1506]
                    tunnel: [w1506] -> w1475
                    tunnel: w1476 -> [w1511]
                    tunnel: w1475 -> [w1510]
                    tunnel: [w1508] -> w1474
                    tunnel: w1474 -> [w1519]
                    tunnel: [w1519] -> w1470
                    tunnel: [w1518] -> w1469
                    frame #0 {
                      n773 = local write "控制读取  2"(w1485) -> ()
                    }
                    frame #1 {
                      n774 = Wait (ms)(milliseconds to wait=u32 50 ("等待时间（毫秒）")) -> ()  [unwired: 1 out]
                    }
                    frame #2 {
                      n775 = local read "VISA资源名称输出"() -> (w1493:refnum<visa-resource-name>)
                      n776 = local read "Curr1"() -> (w1491:dbl)
                      n777 = Number To Fractional String(number=w1491, precision (6)=i16 3 ("精度(6)")) -> (F-format string=w1489:string)  [unwired: 2 out]
                      n778 = Concatenate Strings("volt 1;curr " ("写入缓冲区"), w1489) -> (w1488:string)
                      n779 = VISA Write(VISA resource name=w1493, write buffer=w1488, error in (no error)=w1487) -> (VISA resource name out=w1495:refnum<visa-resource-name>, error out=w1494:errorcluster)  [unwired: 1 out]
                    }
                    frame #3 {
                      n780 = Wait (ms)(milliseconds to wait=u32 50 ("等待时间（毫秒）")) -> ()  [unwired: 1 out]
                    }
                    frame #4 {
                      n781 = VISA Write(VISA resource name=w1504, write buffer=w1500, error in (no error)=w1503) -> (VISA resource name out=w1502:refnum<visa-resource-name>, error out=w1501:errorcluster)  [unwired: 1 out]
                    }
                    frame #5 {
                      n782 = Wait (ms)(milliseconds to wait=u32 200 ("等待时间（毫秒）")) -> ()  [unwired: 1 out]
                    }
                    frame #6 {
                      n783 = Wait (ms)(milliseconds to wait=u32 50 ("等待时间（毫秒）")) -> ()  [unwired: 1 out]
                      n784 = VISA Write(VISA resource name=w1511, write buffer="outp on" ("写入缓冲区"), error in (no error)=w1510) -> (VISA resource name out=w1513:refnum<visa-resource-name>, error out=w1508:errorcluster)  [unwired: 1 out]
                      n785 = local write "VISA资源名称输出"(w1513) -> ()
                    }
                    frame #7 {
                      n786 = while {
                        tunnel: [w1523] -> w1518
                        i -> [w1524]
                        stop <- w1522 stop-if-true
                        n787 = local read "Actual"() -> (w1531:dbl)
                        n788 = local read "Curr1"() -> (w1528:dbl)
                        n789 = Greater Or Equal?(x=w1524, y=20) -> (x >= y?=w1525:bool)
                        n790 = Multiply(x=w1528, y=0.02) -> (x*y=w1527:dbl)
                        n791 = Add(x=w1528, y=w1527) -> (x+y=w1530:dbl)
                        n792 = Subtract(x=w1528, y=w1527) -> (x-y=w1529:dbl)
                        n793 = Wait Until Next ms Multiple(millisecond multiple=u32 200 ("毫秒倍数")) -> ()  [unwired: 1 out]
                        n794 = In Range and Coerce(upper limit=w1530, x=w1531, lower limit=w1529) -> (In Range?=w1523:bool)  [unwired: 1 out]
                        n795 = Or(x=w1523, y=w1525) -> (x .or. y?=w1522:bool)
                      }
                      n796 = local write "控制读取  2"(TRUE ("控制读取")) -> ()
                      n797 = case shown="真" w1518 {
                        tunnel: ["40A电流开启NG" "40A电流开启成功"] -> w1514
                        tunnel: [u32 16711680 u32 6618880] -> w1515
                        frame False {
                        }
                        frame True {
                        }
                      }
                      n798 = control-ref of="结果"() -> (w1516:refnum<vi>)
                      n799 = Build Array(w1514) -> (w1517:string[])
                      n800 = call "表格编辑.vi"("新元素/子数组"=w1517, "活动单元格:单元格背景色"=w1515, "MCListbox引用句柄"=w1516) -> ()  [unwired: 9 out]
                    }
                  }
                  n801 = local read "Curr1"() -> (w1472:dbl)
                  n802 = local write "REAL1"(w1472) -> ()
                  n803 = local write "Set"(w1472) -> ()
                }
                frame 5 {
                  # "5460电压零点"
                  n804 = flat-sequence {
                    tunnel: w1544 -> [w1551]
                    tunnel: w1545 -> [w1552]
                    tunnel: [w1552] -> w1541
                    tunnel: [w1551] -> w1540
                    tunnel: w1541 -> [w1556]
                    tunnel: w1540 -> [w1555]
                    tunnel: [w1554] -> w1539
                    tunnel: [w1553] -> w1538
                    tunnel: [w1563] -> w1542
                    tunnel: [w1564] -> w1543
                    tunnel: w1539 -> [w1564]
                    tunnel: w1538 -> [w1563]
                    tunnel: [w1558] -> w1537
                    frame #0 {
                      n805 = local write "Shunt Volt Offset"("" ("5460Current Offset")) -> ()
                      n806 = global write "EV05全局变量1.vi" "高压校正接收"(FALSE ("高压校正接收")) -> ()
                      n807 = global write "EV05全局变量1.vi" "CAN接收"(FALSE ("CAN接收")) -> ()
                      n808 = call <vilib>:"Set Busy.vi"() -> ()  [unwired: 4 in, 8 out]
                      n809 = property on="Current Offset结果 2" class="Bool (严格)"("Colors [4]"=cluster{u32, u32}[] [{0, 0}] ("颜色[4]"), "BoolText.Text"="" ("布尔文本.文本")) -> ()  [unwired: 2 in, 2 out]
                    }
                    frame #1 {
                      n810 = Enqueue Element(queue=w1556, element="Set Volt offset" ("元素"), error in (no error)=w1555) -> (queue out=w1554:refnum<queue>, error out=w1553:errorcluster)  [unwired: 2 out]
                    }
                    frame #2 {
                      n811 = while {
                        tunnel: [w1570] -> w1558
                        i -> [w1575]
                        stop <- w1571 stop-if-true
                        n812 = property on="Current Offset结果 2" class="Bool (严格)"() -> ("BoolText.Text"=w1569:string)  [unwired: 2 in, 2 out]
                        n813 = Greater Or Equal?(x=w1575, y=30) -> (x >= y?=w1572:bool)
                        n814 = Not Equal?(x=w1569, y="NG" ("布尔文本.文本")) -> (x != y?=w1570:bool)
                        n815 = Wait Until Next ms Multiple(millisecond multiple=u32 110 ("毫秒倍数")) -> ()  [unwired: 1 out]
                        n816 = Or(x=w1570, y=w1572) -> (x .or. y?=w1571:bool)
                      }
                      n817 = case shown="真" w1558 {
                        tunnel: ["5460电压零点校正NG" "5460电压零点校正成功"] -> w1559
                        tunnel: [u32 16711680 u32 6618880] -> w1560
                        frame False {
                        }
                        frame True {
                        }
                      }
                      n818 = control-ref of="结果"() -> (w1561:refnum<vi>)
                      n819 = Build Array(w1559) -> (w1562:string[])
                      n820 = call "表格编辑.vi"("新元素/子数组"=w1562, "活动单元格:单元格背景色"=w1560, "MCListbox引用句柄"=w1561) -> ()  [unwired: 9 out]
                    }
                  }
                }
                frame 6 {
                  # "5460电压增益"
                  n821 = flat-sequence {
                    tunnel: w1584 -> [w1591]
                    tunnel: w1585 -> [w1592]
                    tunnel: [w1592] -> w1581
                    tunnel: [w1591] -> w1580
                    tunnel: w1581 -> [w1596]
                    tunnel: w1580 -> [w1595]
                    tunnel: [w1594] -> w1579
                    tunnel: [w1593] -> w1578
                    tunnel: [w1603] -> w1582
                    tunnel: [w1604] -> w1583
                    tunnel: w1579 -> [w1604]
                    tunnel: w1578 -> [w1603]
                    tunnel: [w1598] -> w1577
                    frame #0 {
                      n822 = local write "Shunt Volt Gain"("" ("5460Current Offset")) -> ()
                      n823 = global write "EV05全局变量1.vi" "高压校正接收"(FALSE ("高压校正接收")) -> ()
                      n824 = global write "EV05全局变量1.vi" "CAN接收"(FALSE ("CAN接收")) -> ()
                      n825 = call <vilib>:"Set Busy.vi"() -> ()  [unwired: 4 in, 8 out]
                      n826 = property on="Current Gain结果 2" class="Bool (严格)"("Colors [4]"=cluster{u32, u32}[] [{0, 0}] ("颜色[4]"), "BoolText.Text"="" ("布尔文本.文本")) -> ()  [unwired: 2 in, 2 out]
                    }
                    frame #1 {
                      n827 = Enqueue Element(queue=w1596, element="Set Volt Gain" ("元素"), error in (no error)=w1595) -> (queue out=w1594:refnum<queue>, error out=w1593:errorcluster)  [unwired: 2 out]
                    }
                    frame #2 {
                      n828 = while {
                        tunnel: [w1610] -> w1598
                        i -> [w1615]
                        stop <- w1611 stop-if-true
                        n829 = property on="Current Gain结果 2" class="Bool (严格)"() -> ("BoolText.Text"=w1609:string)  [unwired: 2 in, 2 out]
                        n830 = Greater Or Equal?(x=w1615, y=30) -> (x >= y?=w1612:bool)
                        n831 = Not Equal?(x=w1609, y="NG" ("布尔文本.文本")) -> (x != y?=w1610:bool)
                        n832 = Wait Until Next ms Multiple(millisecond multiple=u32 110 ("毫秒倍数")) -> ()  [unwired: 1 out]
                        n833 = Or(x=w1610, y=w1612) -> (x .or. y?=w1611:bool)
                      }
                      n834 = case shown="假" w1598 {
                        tunnel: ["5460电压增益校正NG" "5460电压增益校正成功"] -> w1599
                        tunnel: [u32 16711680 u32 6618880] -> w1600
                        frame False {
                        }
                        frame True {
                        }
                      }
                      n835 = control-ref of="结果"() -> (w1601:refnum<vi>)
                      n836 = Build Array(w1599) -> (w1602:string[])
                      n837 = call "表格编辑.vi"("新元素/子数组"=w1602, "活动单元格:单元格背景色"=w1600, "MCListbox引用句柄"=w1601) -> ()  [unwired: 9 out]
                    }
                  }
                }
                frame 7 {
                  # "AD1"
                  n838 = flat-sequence {
                    tunnel: w1624 -> [w1630]
                    tunnel: w1625 -> [w1631]
                    tunnel: [w1631] -> w1618
                    tunnel: [w1630] -> w1617
                    tunnel: [w1638] -> w1623
                    tunnel: [w1637] -> w1622
                    tunnel: w1618 -> [w1638]
                    tunnel: w1617 -> [w1637]
                    tunnel: w1623 -> [w1641]
                    tunnel: w1622 -> [w1640]
                    tunnel: [w1643] -> w1621
                    tunnel: [w1642] -> w1620
                    tunnel: [w1649] -> w1626
                    tunnel: [w1650] -> w1627
                    tunnel: w1621 -> [w1650]
                    tunnel: w1620 -> [w1649]
                    tunnel: [w1648] -> w1619
                    frame #0 {
                      n839 = One Button Dialog(message="请重启主板电源" ("消息"), button name ("OK")="确定" ("T按钮名称（“确定”）")) -> ()  [unwired: 1 out]
                    }
                    frame #1 {
                      n840 = global write "EV05全局变量1.vi" "CAN接收"(FALSE ("CAN接收")) -> ()
                      n841 = global write "EV05全局变量1.vi" "高压校正接收"(FALSE ("高压校正接收")) -> ()
                      n842 = local write "AD1"(u16 0 ("AD1")) -> ()
                      n843 = property on="Read1结果" class="Bool (严格)"("Colors [4]"=cluster{u32, u32}[] [{0, 0}] ("颜色[4]"), "BoolText.Text"="" ("布尔文本.文本")) -> ()  [unwired: 2 in, 2 out]
                    }
                    frame #2 {
                      n844 = Enqueue Element(queue=w1641, element="Read1" ("元素"), error in (no error)=w1640) -> (queue out=w1643:refnum<queue>, error out=w1642:errorcluster)  [unwired: 2 out]
                    }
                    frame #3 {
                      n845 = while {
                        tunnel: [w1655] -> w1648
                        i -> [w1660]
                        stop <- w1656 stop-if-true
                        n846 = property on="Read1结果" class="Bool (严格)"() -> ("BoolText.Text"=w1662:string)  [unwired: 2 in, 2 out]
                        n847 = Greater Or Equal?(x=w1660, y=30) -> (x >= y?=w1657:bool)
                        n848 = Not Equal?(x=w1662, y="NG" ("布尔文本.文本")) -> (x != y?=w1655:bool)
                        n849 = Wait Until Next ms Multiple(millisecond multiple=u32 110 ("毫秒倍数")) -> ()  [unwired: 1 out]
                        n850 = Or(x=w1655, y=w1657) -> (x .or. y?=w1656:bool)
                      }
                      n851 = case shown="真" w1648 {
                        tunnel: ["40A AD1值读取NG" "40A AD1值读取成功"] -> w1644
                        tunnel: [u32 16711680 u32 6618880] -> w1645
                        frame False {
                        }
                        frame True {
                        }
                      }
                      n852 = control-ref of="结果"() -> (w1646:refnum<vi>)
                      n853 = Build Array(w1644) -> (w1647:string[])
                      n854 = call "表格编辑.vi"("新元素/子数组"=w1647, "活动单元格:单元格背景色"=w1645, "MCListbox引用句柄"=w1646) -> ()  [unwired: 9 out]
                    }
                  }
                }
                frame 8 {
                  # "80A"
                  n855 = local read "Curr2"() -> (w1667:dbl)
                  n856 = flat-sequence {
                    tunnel: FALSE ("控制读取") -> [w1680]
                    tunnel: [w1690] -> w1679
                    tunnel: [w1689] -> w1678
                    tunnel: [w1684] -> w1677
                    tunnel: w1666 -> [w1682]
                    tunnel: w1679 -> [w1694]
                    tunnel: [w1694] -> w1676
                    tunnel: w1678 -> [w1693]
                    tunnel: [w1693] -> w1675
                    tunnel: [w1691] -> w1674
                    tunnel: w1677 -> [w1691]
                    tunnel: w1676 -> [w1699]
                    tunnel: w1675 -> [w1698]
                    tunnel: [w1697] -> w1673
                    tunnel: [w1696] -> w1672
                    tunnel: w1674 -> [w1695]
                    tunnel: w1673 -> [w1702]
                    tunnel: [w1702] -> w1671
                    tunnel: w1672 -> [w1701]
                    tunnel: [w1701] -> w1670
                    tunnel: w1671 -> [w1706]
                    tunnel: w1670 -> [w1705]
                    tunnel: [w1703] -> w1669
                    tunnel: w1669 -> [w1714]
                    tunnel: [w1714] -> w1664
                    tunnel: [w1713] -> w1663
                    frame #0 {
                      n857 = local write "控制读取  2"(w1680) -> ()
                    }
                    frame #1 {
                      n858 = Wait (ms)(milliseconds to wait=u32 50 ("等待时间（毫秒）")) -> ()  [unwired: 1 out]
                    }
                    frame #2 {
                      n859 = local read "VISA资源名称输出"() -> (w1688:refnum<visa-resource-name>)
                      n860 = local read "Curr2"() -> (w1683:dbl)
                      n861 = Number To Fractional String(number=w1683, precision (6)=i16 3 ("精度(6)")) -> (F-format string=w1685:string)  [unwired: 2 out]
                      n862 = Concatenate Strings("volt 1;curr " ("写入缓冲区"), w1685) -> (w1684:string)
                      n863 = VISA Write(VISA resource name=w1688, write buffer=w1684, error in (no error)=w1682) -> (VISA resource name out=w1690:refnum<visa-resource-name>, error out=w1689:errorcluster)  [unwired: 1 out]
                    }
                    frame #3 {
                      n864 = Wait (ms)(milliseconds to wait=u32 50 ("等待时间（毫秒）")) -> ()  [unwired: 1 out]
                    }
                    frame #4 {
                      n865 = VISA Write(VISA resource name=w1699, write buffer=w1695, error in (no error)=w1698) -> (VISA resource name out=w1697:refnum<visa-resource-name>, error out=w1696:errorcluster)  [unwired: 1 out]
                    }
                    frame #5 {
                      n866 = Wait (ms)(milliseconds to wait=u32 200 ("等待时间（毫秒）")) -> ()  [unwired: 1 out]
                    }
                    frame #6 {
                      n867 = Wait (ms)(milliseconds to wait=u32 50 ("等待时间（毫秒）")) -> ()  [unwired: 1 out]
                      n868 = VISA Write(VISA resource name=w1706, write buffer="outp on" ("写入缓冲区"), error in (no error)=w1705) -> (VISA resource name out=w1708:refnum<visa-resource-name>, error out=w1703:errorcluster)  [unwired: 1 out]
                      n869 = local write "VISA资源名称输出"(w1708) -> ()
                    }
                    frame #7 {
                      n870 = while {
                        tunnel: [w1718] -> w1713
                        i -> [w1716]
                        stop <- w1717 stop-if-true
                        n871 = local read "Curr2"() -> (w1722:dbl)
                        n872 = local read "Actual"() -> (w1726:dbl)
                        n873 = Greater Or Equal?(x=w1716, y=20) -> (x >= y?=w1720:bool)
                        n874 = Multiply(x=w1722, y=0.02) -> (x*y=w1723:dbl)
                        n875 = Add(x=w1722, y=w1723) -> (x+y=w1725:dbl)
                        n876 = Subtract(x=w1722, y=w1723) -> (x-y=w1724:dbl)
                        n877 = Wait Until Next ms Multiple(millisecond multiple=u32 200 ("毫秒倍数")) -> ()  [unwired: 1 out]
                        n878 = In Range and Coerce(upper limit=w1725, x=w1726, lower limit=w1724) -> (In Range?=w1718:bool)  [unwired: 1 out]
                        n879 = Or(x=w1718, y=w1720) -> (x .or. y?=w1717:bool)
                      }
                      n880 = local write "控制读取  2"(TRUE ("控制读取")) -> ()
                      n881 = case shown="真" w1713 {
                        tunnel: ["80A电流开启NG" "80A电流开启成功"] -> w1709
                        tunnel: [u32 16711680 u32 6618880] -> w1710
                        frame False {
                        }
                        frame True {
                        }
                      }
                      n882 = control-ref of="结果"() -> (w1711:refnum<vi>)
                      n883 = Build Array(w1709) -> (w1712:string[])
                      n884 = call "表格编辑.vi"("新元素/子数组"=w1712, "活动单元格:单元格背景色"=w1710, "MCListbox引用句柄"=w1711) -> ()  [unwired: 9 out]
                    }
                  }
                  n885 = local write "REAL2"(w1667) -> ()
                  n886 = local write "Set"(w1667) -> ()
                }
                frame 9 {
                  # "AD2"
                  n887 = flat-sequence {
                    tunnel: w1737 -> [w1746]
                    tunnel: w1738 -> [w1747]
                    tunnel: [w1747] -> w1736
                    tunnel: [w1746] -> w1735
                    tunnel: w1736 -> [w1750]
                    tunnel: w1735 -> [w1749]
                    tunnel: [w1752] -> w1734
                    tunnel: [w1751] -> w1733
                    tunnel: [w1758] -> w1739
                    tunnel: [w1759] -> w1740
                    tunnel: w1734 -> [w1759]
                    tunnel: w1733 -> [w1758]
                    tunnel: [w1757] -> w1732
                    frame #0 {
                      n888 = local write "AD2"(u16 0 ("AD2")) -> ()
                      n889 = global write "EV05全局变量1.vi" "CAN接收"(FALSE ("CAN接收")) -> ()
                      n890 = global write "EV05全局变量1.vi" "高压校正接收"(FALSE ("高压校正接收")) -> ()
                      n891 = property on="Read2结果" class="Bool (严格)"("Colors [4]"=cluster{u32, u32}[] [{0, 0}] ("颜色[4]"), "BoolText.Text"="" ("布尔文本.文本")) -> ()  [unwired: 2 in, 2 out]
                    }
                    frame #1 {
                      n892 = Enqueue Element(queue=w1750, element="Read2" ("元素"), error in (no error)=w1749) -> (queue out=w1752:refnum<queue>, error out=w1751:errorcluster)  [unwired: 2 out]
                    }
                    frame #2 {
                      n893 = while {
                        tunnel: [w1765] -> w1757
                        i -> [w1770]
                        stop <- w1766 stop-if-true
                        n894 = property on="Read2结果" class="Bool (严格)"() -> ("BoolText.Text"=w1764:string)  [unwired: 2 in, 2 out]
                        n895 = Greater Or Equal?(x=w1770, y=30) -> (x >= y?=w1767:bool)
                        n896 = Not Equal?(x=w1764, y="NG" ("布尔文本.文本")) -> (x != y?=w1765:bool)
                        n897 = Wait Until Next ms Multiple(millisecond multiple=u32 110 ("毫秒倍数")) -> ()  [unwired: 1 out]
                        n898 = Or(x=w1765, y=w1767) -> (x .or. y?=w1766:bool)
                      }
                      n899 = case shown="假" w1757 {
                        tunnel: ["80A AD2值读取NG" "80A AD2值读取成功"] -> w1753
                        tunnel: [u32 16711680 u32 6618880] -> w1754
                        frame False {
                        }
                        frame True {
                        }
                      }
                      n900 = control-ref of="结果"() -> (w1755:refnum<vi>)
                      n901 = Build Array(w1753) -> (w1756:string[])
                      n902 = call "表格编辑.vi"("新元素/子数组"=w1756, "活动单元格:单元格背景色"=w1754, "MCListbox引用句柄"=w1755) -> ()  [unwired: 9 out]
                    }
                  }
                }
                frame 10 {
                  # "写入电流增益"
                  n903 = flat-sequence {
                    tunnel: w1779 -> [w1795]
                    tunnel: w1780 -> [w1796]
                    tunnel: [w1796] -> w1776
                    tunnel: [w1795] -> w1775
                    tunnel: w1776 -> [w1801]
                    tunnel: w1775 -> [w1800]
                    tunnel: [w1799] -> w1774
                    tunnel: [w1798] -> w1773
                    tunnel: [w1807] -> w1778
                    tunnel: [w1808] -> w1777
                    tunnel: w1774 -> [w1808]
                    tunnel: w1773 -> [w1807]
                    tunnel: [w1806] -> w1772
                    frame #0 {
                      n904 = local read "REAL2"() -> (w1793:dbl)
                      n905 = local read "REAL1"() -> (w1792:dbl)
                      n906 = local read "AD1"() -> (w1788:u16)
                      n907 = local read "AD2"() -> (w1789:u16)
                      n908 = Subtract(x=w1793, y=w1792) -> (x-y=w1791:dbl)
                      n909 = Subtract(x=w1789, y=w1788) -> (x-y=w1787:u16)
                      n910 = Multiply(x=w1791, y=1000000.0) -> (x*y=w1790:dbl)
                      n911 = global write "EV05全局变量1.vi" "CAN接收"(FALSE ("CAN接收")) -> ()
                      n912 = Divide(x=w1790, y=w1787) -> (x/y=w1786:dbl)
                      n913 = Round Toward -Infinity(1:w1786) -> (0:w1785:dbl)
                      n914 = local write "Gain"(w1785) -> ()
                      n915 = global write "EV05全局变量1.vi" "高压校正接收"(FALSE ("高压校正接收")) -> ()
                      n916 = property on="Set结果" class="Bool (严格)"("Colors [4]"=cluster{u32, u32}[] [{0, 0}] ("颜色[4]"), "BoolText.Text"="" ("布尔文本.文本")) -> ()  [unwired: 2 in, 2 out]
                    }
                    frame #1 {
                      n917 = Enqueue Element(queue=w1801, element="Set" ("元素"), error in (no error)=w1800) -> (queue out=w1798:refnum<queue>, error out=w1799:errorcluster)  [unwired: 2 out]
                    }
                    frame #2 {
                      n918 = while {
                        tunnel: [w1814] -> w1806
                        i -> [w1819]
                        stop <- w1815 stop-if-true
                        n919 = property on="Set结果" class="Bool (严格)"() -> ("BoolText.Text"=w1813:string)  [unwired: 2 in, 2 out]
                        n920 = Greater Or Equal?(x=w1819, y=30) -> (x >= y?=w1816:bool)
                        n921 = Not Equal?(x=w1813, y="NG" ("布尔文本.文本")) -> (x != y?=w1814:bool)
                        n922 = Wait Until Next ms Multiple(millisecond multiple=u32 110 ("毫秒倍数")) -> ()  [unwired: 1 out]
                        n923 = Or(x=w1814, y=w1816) -> (x .or. y?=w1815:bool)
                      }
                      n924 = case shown="假" w1806 {
                        tunnel: ["设电流增益NG" "设电流增益成功"] -> w1802
                        tunnel: [u32 16711680 u32 6618880] -> w1803
                        frame False {
                        }
                        frame True {
                        }
                      }
                      n925 = control-ref of="结果"() -> (w1804:refnum<vi>)
                      n926 = Build Array(w1802) -> (w1805:string[])
                      n927 = call "表格编辑.vi"("新元素/子数组"=w1805, "活动单元格:单元格背景色"=w1803, "MCListbox引用句柄"=w1804) -> ()  [unwired: 9 out]
                    }
                  }
                }
                frame 11 {
                  # "检验电流校正状态"
                  n928 = flat-sequence {
                    tunnel: [w1843] -> w1838
                    tunnel: [w1848] -> w1837
                    tunnel: w1838 -> [w1848]
                    tunnel: [w1859] -> w1836
                    tunnel: [w1858] -> w1835
                    tunnel: [w1853] -> w1834
                    tunnel: w1842 -> [w1852]
                    tunnel: [w1850] -> w1833
                    tunnel: w1837 -> [w1850]
                    tunnel: w1836 -> [w1864]
                    tunnel: [w1864] -> w1832
                    tunnel: w1835 -> [w1863]
                    tunnel: [w1863] -> w1831
                    tunnel: [w1861] -> w1830
                    tunnel: w1834 -> [w1861]
                    tunnel: [w1860] -> w1829
                    tunnel: w1833 -> [w1860]
                    tunnel: w1832 -> [w1870]
                    tunnel: w1831 -> [w1869]
                    tunnel: [w1868] -> w1828
                    tunnel: [w1867] -> w1827
                    tunnel: w1830 -> [w1866]
                    tunnel: [w1865] -> w1826
                    tunnel: w1829 -> [w1865]
                    tunnel: w1828 -> [w1874]
                    tunnel: [w1874] -> w1825
                    tunnel: w1827 -> [w1873]
                    tunnel: [w1873] -> w1824
                    tunnel: [w1871] -> w1823
                    tunnel: w1826 -> [w1871]
                    tunnel: w1825 -> [w1879]
                    tunnel: w1824 -> [w1878]
                    tunnel: [w1876] -> w1822
                    tunnel: [w1875] -> w1821
                    tunnel: w1823 -> [w1875]
                    tunnel: w1822 -> [w1884]
                    tunnel: [w1884] -> w1841
                    tunnel: [w1882] -> w1840
                    tunnel: w1821 -> [w1883]
                    frame #0 {
                      n929 = local read "Actual"() -> (w1845:dbl)
                      n930 = local read "Curr"() -> (w1847:dbl)
                      n931 = Subtract(x=w1845, y=w1847) -> (x-y=w1846:dbl)
                      n932 = Absolute Value(x=w1846) -> (abs(x)=w1844:dbl)
                      n933 = Divide(x=w1844, y=w1845) -> (x/y=w1843:dbl)
                    }
                    frame #1 {
                      n934 = Wait (ms)(milliseconds to wait=u32 50 ("等待时间（毫秒）")) -> ()  [unwired: 1 out]
                    }
                    frame #2 {
                      n935 = local read "VISA资源名称输出"() -> (w1857:refnum<visa-resource-name>)
                      n936 = Number To Fractional String(number=200.0 ("数字"), precision (6)=i16 3 ("精度(6)")) -> (F-format string=w1854:string)  [unwired: 2 out]
                      n937 = Concatenate Strings("volt 1;curr " ("写入缓冲区"), w1854) -> (w1853:string)
                      n938 = VISA Write(VISA resource name=w1857, write buffer=w1853, error in (no error)=w1852) -> (VISA resource name out=w1859:refnum<visa-resource-name>, error out=w1858:errorcluster)  [unwired: 1 out]
                    }
                    frame #3 {
                      n939 = Wait (ms)(milliseconds to wait=u32 50 ("等待时间（毫秒）")) -> ()  [unwired: 1 out]
                    }
                    frame #4 {
                      n940 = VISA Write(VISA resource name=w1870, write buffer=w1866, error in (no error)=w1869) -> (VISA resource name out=w1868:refnum<visa-resource-name>, error out=w1867:errorcluster)  [unwired: 1 out]
                    }
                    frame #5 {
                      n941 = Wait (ms)(milliseconds to wait=u32 200 ("等待时间（毫秒）")) -> ()  [unwired: 1 out]
                    }
                    frame #6 {
                      n942 = Wait (ms)(milliseconds to wait=u32 50 ("等待时间（毫秒）")) -> ()  [unwired: 1 out]
                      n943 = VISA Write(VISA resource name=w1879, write buffer="outp on" ("写入缓冲区"), error in (no error)=w1878) -> (VISA resource name out=w1881:refnum<visa-resource-name>, error out=w1876:errorcluster)  [unwired: 1 out]
                      n944 = local write "VISA资源名称输出"(w1881) -> ()
                    }
                    frame #7 {
                      n945 = stacked-sequence {
                        seq-local: [w1885 _ _] -> [_ w1898 _]
                        tunnel: w1883 -> [_ _ w1919]
                        tunnel: [_ w1898 _] -> w1882
                        frame #0 {
                          n946 = while {
                            tunnel: [w1889] -> w1885
                            i -> [w1887]
                            stop <- w1888 stop-if-true
                            w1886 = 200.0 ("y")
                            n947 = local read "Actual"() -> (w1896:dbl)
                            n948 = Greater Or Equal?(x=w1887, y=20) -> (x >= y?=w1891:bool)
                            n949 = Multiply(x=w1886, y=0.02) -> (x*y=w1893:dbl)
                            n950 = Add(x=w1886, y=w1893) -> (x+y=w1895:dbl)
                            n951 = Subtract(x=w1886, y=w1893) -> (x-y=w1894:dbl)
                            n952 = Wait Until Next ms Multiple(millisecond multiple=u32 200 ("毫秒倍数")) -> ()  [unwired: 1 out]
                            n953 = In Range and Coerce(upper limit=w1895, x=w1896, lower limit=w1894) -> (In Range?=w1889:bool)  [unwired: 1 out]
                            n954 = Or(x=w1889, y=w1891) -> (x .or. y?=w1888:bool)
                          }
                        }
                        frame #1 {
                          n955 = case shown="假" w1898 {
                            tunnel: ["200A电流开启NG" "200A电流开启成功"] -> w1899
                            tunnel: [u32 16711680 u32 6618880] -> w1900
                            frame False {
                            }
                            frame True {
                            }
                          }
                          n956 = control-ref of="结果"() -> (w1901:refnum<vi>)
                          n957 = Build Array(w1899) -> (w1902:string[])
                          n958 = call "表格编辑.vi"("新元素/子数组"=w1902, "活动单元格:单元格背景色"=w1900, "MCListbox引用句柄"=w1901) -> ()  [unwired: 9 out]
                        }
                        frame #2 {
                          n959 = local read "Actual"() -> (w1924:dbl)
                          n960 = local read "Curr"() -> (w1923:dbl)
                          n961 = Multiply(x=w1919, y=100.0) -> (x*y=w1920:dbl)
                          n962 = Subtract(x=w1924, y=w1923) -> (x-y=w1925:dbl)
                          n963 = Format Into String(format string="%.3f%" ("格式字符串"), w1920) -> (resulting string=w1917:string)  [unwired: 2 in, 1 out]
                          n964 = Absolute Value(x=w1925) -> (abs(x)=w1926:dbl)
                          n965 = Divide(x=w1926, y=w1924) -> (x/y=w1914:dbl)
                          n966 = Multiply(x=w1914, y=100.0) -> (x*y=w1915:dbl)
                          n967 = Format Into String(format string="%.3f%" ("格式字符串"), w1915) -> (resulting string=w1912:string)  [unwired: 2 in, 1 out]
                          n968 = Concatenate Strings("80A误差", w1917, "  200A误差", w1912) -> (w1907:string)
                          n969 = control-ref of="结果"() -> (w1909:refnum<vi>)
                          n970 = Build Array(w1907) -> (w1910:string[])
                          n971 = call "表格编辑.vi"("新元素/子数组"=w1910, "活动单元格:单元格背景色"=u32 6618880, "MCListbox引用句柄"=w1909) -> ()  [unwired: 9 out]
                        }
                      }
                    }
                  }
                }
                frame 12 {
                  # "关闭电流源"
                  n972 = local read "VISA资源名称输出"() -> (w1933:refnum<visa-resource-name>)
                  n973 = local write "控制读取  2"(FALSE ("控制读取")) -> ()
                  n974 = flat-sequence {
                    tunnel: [w1942] -> w1940
                    tunnel: w1933 -> [w1942]
                    tunnel: w1940 -> [w1946]
                    tunnel: [w1945] -> w1939
                    tunnel: w1932 -> [w1944]
                    tunnel: [w1943] -> w1938
                    tunnel: w1939 -> [w1950]
                    tunnel: [w1950] -> w1937
                    tunnel: [w1948] -> w1936
                    tunnel: w1938 -> [w1948]
                    tunnel: w1937 -> [w1955]
                    tunnel: w1936 -> [w1952]
                    tunnel: [w1954] -> w1928
                    tunnel: [w1951] -> w1927
                    tunnel: [w1961] -> w1930
                    tunnel: [w1962] -> w1934
                    tunnel: w1928 -> [w1962]
                    tunnel: w1927 -> [w1961]
                    frame #0 {
                      n975 = Wait (ms)(milliseconds to wait=u32 200 ("等待时间（毫秒）")) -> ()  [unwired: 1 out]
                    }
                    frame #1 {
                      n976 = VISA Write(VISA resource name=w1946, write buffer="outp off" ("写入缓冲区"), error in (no error)=w1944) -> (VISA resource name out=w1945:refnum<visa-resource-name>, error out=w1943:errorcluster)  [unwired: 1 out]
                    }
                    frame #2 {
                      n977 = Wait (ms)(milliseconds to wait=u32 50 ("等待时间（毫秒）")) -> ()  [unwired: 1 out]
                    }
                    frame #3 {
                      n978 = local write "控制读取  2"(TRUE ("控制读取")) -> ()
                      n979 = VISA Write(VISA resource name=w1955, write buffer="outp off" ("写入缓冲区"), error in (no error)=w1952) -> (VISA resource name out=w1954:refnum<visa-resource-name>, error out=w1951:errorcluster)  [unwired: 1 out]
                    }
                    frame #4 {
                      n980 = control-ref of="结果"() -> (w1959:refnum<vi>)
                      n981 = Build Array("电流源关闭") -> (w1960:string[])
                      n982 = call "表格编辑.vi"("新元素/子数组"=w1960, "活动单元格:单元格背景色"=u32 6618880, "MCListbox引用句柄"=w1959) -> ()  [unwired: 9 out]
                    }
                  }
                  n983 = local write "VISA资源名称输出"(w1934) -> ()
                }
                frame 13 {
                  # "打开电压源"
                  n984 = local read "VISA resource name 4"() -> (w1972:refnum<visa-resource-name>)
                  n985 = VISA Open(error in (no error)=w1971, VISA resource name=w1972) -> (VISA resource name=w1976:refnum<visa-resource-name>, error out=w1975:errorcluster)  [unwired: 1 in, 2 out]
                  n986 = property class="Instr"(reference=w1976, error in=w1975, "Timeout"=u32 100 ("General Settings:Timeout Value")) -> (reference out=w1973:refnum<visa-resource-name>, error out=w1974:errorcluster)
                  n987 = call-poly "VISA Configure Serial Port"("VISA resource name"=w1973, "error in (no error)"=w1974) -> ("VISA resource name out"=w1978:refnum<visa-resource-name>, "error out"=w1970:errorcluster)  [unwired: 4 in, 8 out]
                  n988 = Unbundle(w1970) -> ("status"=w1969:bool)  [unwired: 2 out]
                  n989 = case shown="真" w1969 {
                    tunnel: w1978 -> [w1984 w1989]
                    tunnel: ["电压源打开成功" "电压源打开成功"] -> w1964
                    tunnel: [u32 6618880 u32 16711680] -> w1963
                    frame False {
                      w1982 = u8 0 ("禁用")
                      n990 = local write "VISA资源名称输出 10"(w1984) -> ()
                      n991 = local write "连接状态 10"(TRUE ("连接状态")) -> ()
                      n992 = property on="输出150V" class="Bool"("Disabled"=w1982) -> ()  [unwired: 2 in, 2 out]
                      n993 = property on="输出300V" class="Bool"("Disabled"=w1982) -> ()  [unwired: 2 in, 2 out]
                      n994 = property on="输出自定义值2" class="Bool"("Disabled"=w1982) -> ()  [unwired: 2 in, 2 out]
                      n995 = property on="输出自定义值1" class="Bool"("Disabled"=w1982) -> ()  [unwired: 2 in, 2 out]
                      n996 = property on="连接状态 10" class="Bool (严格)"("Colors [4]"=cluster{u32, u32}[] [{6618880, 6618880}] ("颜色[4]")) -> ()  [unwired: 2 in, 2 out]
                    }
                    frame True {
                      w1988 = u8 2 ("禁用")
                      n997 = local write "VISA资源名称输出 10"(w1989) -> ()
                      n998 = local write "连接状态 10"(FALSE ("连接状态")) -> ()
                      n999 = property on="输出自定义值2" class="Bool"("Disabled"=w1988) -> ()  [unwired: 2 in, 2 out]
                      n1000 = property on="输出150V" class="Bool"("Disabled"=w1988) -> ()  [unwired: 2 in, 2 out]
                      n1001 = property on="输出自定义值1" class="Bool"("Disabled"=w1988) -> ()  [unwired: 2 in, 2 out]
                      n1002 = property on="输出300V" class="Bool"("Disabled"=w1988) -> ()  [unwired: 2 in, 2 out]
                      n1003 = property on="连接状态 10" class="Bool (严格)"("Colors [4]"=cluster{u32, u32}[] [{15663131, 6618880}] ("颜色[4]")) -> ()  [unwired: 2 in, 2 out]
                    }
                  }
                  n1004 = control-ref of="结果"() -> (w1966:refnum<vi>)
                  n1005 = Build Array(w1964) -> (w1965:string[])
                  n1006 = call "表格编辑.vi"("新元素/子数组"=w1965, "活动单元格:单元格背景色"=w1963, "MCListbox引用句柄"=w1966) -> ()  [unwired: 9 out]
                  n1007 = Not(x=w1969) -> (.not. x?=w1968:bool)
                }
                frame 14 {
                  w2004 = "," ("字符串")
                  # "150V"
                  n1008 = local read "Volt1"() -> (w1992:dbl)
                  n1009 = local write "REAL1"(w1992) -> ()
                  n1010 = local write "REAL1"(w1992) -> ()
                  n1011 = local write "Set"(w1992) -> ()
                  n1012 = local write "控制读取  5"(FALSE ("控制读取")) -> ()
                  n1013 = Number To Fractional String(number=w1992, precision (6)=i16 2 ("精度(6)")) -> (F-format string=w2008:string)  [unwired: 2 out]
                  n1014 = Number To Fractional String(number=0.2 ("数字"), precision (6)=i16 2 ("精度(6)")) -> (F-format string=w2007:string)  [unwired: 2 out]
                  n1015 = Number To Fractional String(number=1.0 ("数字"), precision (6)=i16 2 ("精度(6)")) -> (F-format string=w2005:string)  [unwired: 2 out]
                  n1016 = Number To Fractional String(number=320.0 ("数字"), precision (6)=i16 2 ("精度(6)")) -> (F-format string=w2006:string)  [unwired: 2 out]
                  n1017 = Concatenate Strings(w2008, w2004, w2007, w2004, w2006, w2004, w2005, w2004, w2004, w2004) -> (w2003:string)
                  n1018 = flat-sequence {
                    tunnel: [w2027] -> w2019
                    tunnel: [w2026] -> w2018
                    tunnel: [w2025] -> w2017
                    tunnel: w2003 -> [w2022]
                    tunnel: w1995 -> [w2021]
                    tunnel: w2019 -> [w2032]
                    tunnel: [w2032] -> w2016
                    tunnel: w2018 -> [w2031]
                    tunnel: [w2031] -> w2015
                    tunnel: w2017 -> [w2030]
                    tunnel: [w2030] -> w2014
                    tunnel: w2016 -> [w2036]
                    tunnel: w2015 -> [w2035]
                    tunnel: w2014 -> [_]
                    tunnel: [w2034] -> w2013
                    tunnel: [w2033] -> w2012
                    tunnel: w2013 -> [w2042]
                    tunnel: [w2042] -> w2011
                    tunnel: w2012 -> [w2041]
                    tunnel: [w2041] -> w2010
                    tunnel: w2011 -> [w2045]
                    tunnel: w2010 -> [w2044]
                    tunnel: [w2043] -> w1993
                    tunnel: [w2053] -> w1991
                    frame #0 {
                      n1019 = Wait (ms)(milliseconds to wait=u32 50 ("等待时间（毫秒）")) -> ()  [unwired: 1 out]
                    }
                    frame #1 {
                      n1020 = local read "VISA资源名称输出 10"() -> (w2024:refnum<visa-resource-name>)
                      n1021 = Concatenate Strings("SET:GRO 12," ("写入缓冲区"), w2022, "\n") -> (w2025:string)
                      n1022 = VISA Write(VISA resource name=w2024, write buffer=w2025, error in (no error)=w2021) -> (VISA resource name out=w2027:refnum<visa-resource-name>, error out=w2026:errorcluster)  [unwired: 1 out]
                    }
                    frame #2 {
                      n1023 = Wait (ms)(milliseconds to wait=u32 50 ("等待时间（毫秒）")) -> ()  [unwired: 1 out]
                    }
                    frame #3 {
                      n1024 = Concatenate Strings("SET:STE 12" ("写入缓冲区"), "\n") -> (w2037:string)
                      n1025 = VISA Write(VISA resource name=w2036, write buffer=w2037, error in (no error)=w2035) -> (VISA resource name out=w2034:refnum<visa-resource-name>, error out=w2033:errorcluster)  [unwired: 1 out]
                    }
                    frame #4 {
                      n1026 = Wait (ms)(milliseconds to wait=u32 200 ("等待时间（毫秒）")) -> ()  [unwired: 1 out]
                    }
                    frame #5 {
                      n1027 = Concatenate Strings("OUT:ON" ("写入缓冲区"), "\n") -> (w2050:string)
                      n1028 = Wait (ms)(milliseconds to wait=u32 50 ("等待时间（毫秒）")) -> ()  [unwired: 1 out]
                      n1029 = VISA Write(VISA resource name=w2045, write buffer=w2050, error in (no error)=w2044) -> (VISA resource name out=w2047:refnum<visa-resource-name>, error out=w2043:errorcluster)  [unwired: 1 out]
                      n1030 = local write "VISA资源名称输出 10"(w2047) -> ()
                    }
                    frame #6 {
                      n1031 = while {
                        tunnel: [w2058] -> w2053
                        i -> [w2059]
                        stop <- w2057 stop-if-true
                        n1032 = local read "Actual"() -> (w2064:dbl)
                        n1033 = local read "Volt1"() -> (w2063:dbl)
                        n1034 = Greater Or Equal?(x=w2059, y=20) -> (x >= y?=w2061:bool)
                        n1035 = Multiply(x=w2063, y=0.02) -> (x*y=w2065:dbl)
                        n1036 = Add(x=w2063, y=w2065) -> (x+y=w2067:dbl)
                        n1037 = Subtract(x=w2063, y=w2065) -> (x-y=w2066:dbl)
                        n1038 = Wait Until Next ms Multiple(millisecond multiple=u32 200 ("毫秒倍数")) -> ()  [unwired: 1 out]
                        n1039 = In Range and Coerce(upper limit=w2067, x=w2064, lower limit=w2066) -> (In Range?=w2058:bool)  [unwired: 1 out]
                        n1040 = Or(x=w2058, y=w2061) -> (x .or. y?=w2057:bool)
                      }
                      n1041 = case shown="假" w2053 {
                        tunnel: ["150V电压开启NG" "150V电压开启成功"] -> w2052
                        tunnel: [u32 16711680 u32 6618880] -> w2051
                        frame False {
                        }
                        frame True {
                        }
                      }
                      n1042 = control-ref of="结果"() -> (w2055:refnum<vi>)
                      n1043 = Build Array(w2052) -> (w2054:string[])
                      n1044 = local write "控制读取  5"(TRUE ("控制读取")) -> ()
                      n1045 = call "表格编辑.vi"("新元素/子数组"=w2054, "活动单元格:单元格背景色"=w2051, "MCListbox引用句柄"=w2055) -> ()  [unwired: 9 out]
                    }
                  }
                }
                frame 15 {
                  # "150V内总压AD1"
                  n1046 = flat-sequence {
                    tunnel: w2080 -> [w2086]
                    tunnel: w2081 -> [w2087]
                    tunnel: [w2087] -> w2074
                    tunnel: [w2086] -> w2073
                    tunnel: [w2094] -> w2083
                    tunnel: [w2093] -> w2082
                    tunnel: w2074 -> [w2094]
                    tunnel: w2073 -> [w2093]
                    tunnel: w2083 -> [w2099]
                    tunnel: w2082 -> [w2098]
                    tunnel: [w2097] -> w2077
                    tunnel: [w2096] -> w2076
                    tunnel: [w2105] -> w2079
                    tunnel: [w2106] -> w2078
                    tunnel: w2077 -> [w2106]
                    tunnel: w2076 -> [w2105]
                    tunnel: [w2104] -> w2075
                    frame #0 {
                      n1047 = One Button Dialog(message="请把继电器调到\n内总压状态" ("消息"), button name ("OK")="确定" ("按钮名称（“确定”）")) -> ()  [unwired: 1 out]
                    }
                    frame #1 {
                      n1048 = global write "EV05全局变量1.vi" "CAN接收"(FALSE ("CAN接收")) -> ()
                      n1049 = global write "EV05全局变量1.vi" "高压校正接收"(FALSE ("高压校正接收")) -> ()
                      n1050 = local write "AD1"(0.0 ("AD1 2")) -> ()
                      n1051 = property on="Read1_in结果" class="Bool (严格)"("Colors [4]"=cluster{u32, u32}[] [{0, 0}] ("颜色[4]"), "BoolText.Text"="" ("布尔文本.文本")) -> ()  [unwired: 2 in, 2 out]
                    }
                    frame #2 {
                      n1052 = Enqueue Element(queue=w2099, element="Read1_in" ("元素"), error in (no error)=w2098) -> (queue out=w2096:refnum<queue>, error out=w2097:errorcluster)  [unwired: 2 out]
                    }
                    frame #3 {
                      n1053 = while {
                        tunnel: [w2112] -> w2104
                        i -> [w2117]
                        stop <- w2113 stop-if-true
                        n1054 = property on="Read1_in结果" class="Bool (严格)"() -> ("BoolText.Text"=w2111:string)  [unwired: 2 in, 2 out]
                        n1055 = Greater Or Equal?(x=w2117, y=30) -> (x >= y?=w2114:bool)
                        n1056 = Not Equal?(x=w2111, y="NG" ("布尔文本.文本")) -> (x != y?=w2112:bool)
                        n1057 = Wait Until Next ms Multiple(millisecond multiple=u32 110 ("毫秒倍数")) -> ()  [unwired: 1 out]
                        n1058 = Or(x=w2112, y=w2114) -> (x .or. y?=w2113:bool)
                      }
                      n1059 = case shown="假" w2104 {
                        tunnel: ["内总压AD1值读取NG" "内总压AD1值读取成功"] -> w2101
                        tunnel: [u32 16711680 u32 6618880] -> w2100
                        frame False {
                        }
                        frame True {
                        }
                      }
                      n1060 = control-ref of="结果"() -> (w2102:refnum<vi>)
                      n1061 = Build Array(w2101) -> (w2103:string[])
                      n1062 = call "表格编辑.vi"("新元素/子数组"=w2103, "活动单元格:单元格背景色"=w2100, "MCListbox引用句柄"=w2102) -> ()  [unwired: 9 out]
                    }
                  }
                }
                frame 16 {
                  # "150V外总压AD1"
                  n1063 = flat-sequence {
                    tunnel: w2126 -> [w2132]
                    tunnel: w2127 -> [w2133]
                    tunnel: [w2133] -> w2120
                    tunnel: [w2132] -> w2119
                    tunnel: [w2140] -> w2129
                    tunnel: [w2139] -> w2128
                    tunnel: w2120 -> [w2140]
                    tunnel: w2119 -> [w2139]
                    tunnel: w2129 -> [w2145]
                    tunnel: w2128 -> [w2144]
                    tunnel: [w2143] -> w2123
                    tunnel: [w2142] -> w2122
                    tunnel: [w2151] -> w2125
                    tunnel: [w2152] -> w2124
                    tunnel: w2123 -> [w2152]
                    tunnel: w2122 -> [w2151]
                    tunnel: [w2150] -> w2121
                    frame #0 {
                      n1064 = One Button Dialog(message="请把继电器调到\n外总压状态" ("消息"), button name ("OK")="确定" ("按钮名称（“确定”）")) -> ()  [unwired: 1 out]
                    }
                    frame #1 {
                      n1065 = global write "EV05全局变量1.vi" "CAN接收"(FALSE ("CAN接收")) -> ()
                      n1066 = local write "AD1"(0.0 ("AD1 3")) -> ()
                      n1067 = global write "EV05全局变量1.vi" "高压校正接收"(FALSE ("高压校正接收")) -> ()
                      n1068 = property on="Read1_Out结果" class="Bool (严格)"("Colors [4]"=cluster{u32, u32}[] [{0, 0}] ("颜色[4]"), "BoolText.Text"="" ("布尔文本.文本")) -> ()  [unwired: 2 in, 2 out]
                    }
                    frame #2 {
                      n1069 = Enqueue Element(queue=w2145, element="Read1_out" ("元素"), error in (no error)=w2144) -> (queue out=w2142:refnum<queue>, error out=w2143:errorcluster)  [unwired: 2 out]
                    }
                    frame #3 {
                      n1070 = while {
                        tunnel: [w2158] -> w2150
                        i -> [w2163]
                        stop <- w2159 stop-if-true
                        n1071 = property on="Read1_Out结果" class="Bool (严格)"() -> ("BoolText.Text"=w2157:string)  [unwired: 2 in, 2 out]
                        n1072 = Greater Or Equal?(x=w2163, y=30) -> (x >= y?=w2160:bool)
                        n1073 = Not Equal?(x=w2157, y="NG" ("布尔文本.文本")) -> (x != y?=w2158:bool)
                        n1074 = Or(x=w2158, y=w2160) -> (x .or. y?=w2159:bool)
                        n1075 = Wait Until Next ms Multiple(millisecond multiple=u32 110 ("毫秒倍数")) -> ()  [unwired: 1 out]
                      }
                      n1076 = case shown="真" w2150 {
                        tunnel: ["外总压AD1值读取NG" "外总压AD1值读取成功"] -> w2147
                        tunnel: [u32 16711680 u32 6618880] -> w2146
                        frame False {
                        }
                        frame True {
                        }
                      }
                      n1077 = control-ref of="结果"() -> (w2148:refnum<vi>)
                      n1078 = Build Array(w2147) -> (w2149:string[])
                      n1079 = call "表格编辑.vi"("新元素/子数组"=w2149, "活动单元格:单元格背景色"=w2146, "MCListbox引用句柄"=w2148) -> ()  [unwired: 9 out]
                    }
                  }
                }
                frame 17 {
                  w2178 = "," ("字符串")
                  # "300V"
                  n1080 = local read "Volt2"() -> (w2165:dbl)
                  n1081 = local write "REAL2"(w2165) -> ()
                  n1082 = local write "REAL2"(w2165) -> ()
                  n1083 = local write "Set"(w2165) -> ()
                  n1084 = local write "控制读取  5"(FALSE ("控制读取")) -> ()
                  n1085 = Number To Fractional String(number=w2165, precision (6)=i16 2 ("精度(6)")) -> (F-format string=w2182:string)  [unwired: 2 out]
                  n1086 = Number To Fractional String(number=0.2 ("数字"), precision (6)=i16 2 ("精度(6)")) -> (F-format string=w2181:string)  [unwired: 2 out]
                  n1087 = Number To Fractional String(number=1.0 ("数字"), precision (6)=i16 2 ("精度(6)")) -> (F-format string=w2179:string)  [unwired: 2 out]
                  n1088 = Number To Fractional String(number=320.0 ("数字"), precision (6)=i16 2 ("精度(6)")) -> (F-format string=w2180:string)  [unwired: 2 out]
                  n1089 = Concatenate Strings(w2182, w2178, w2181, w2178, w2180, w2178, w2179, w2178, w2178, w2178) -> (w2177:string)
                  n1090 = flat-sequence {
                    tunnel: [w2201] -> w2193
                    tunnel: [w2200] -> w2192
                    tunnel: [w2199] -> w2191
                    tunnel: w2177 -> [w2196]
                    tunnel: w2169 -> [w2195]
                    tunnel: w2193 -> [w2206]
                    tunnel: [w2206] -> w2190
                    tunnel: w2192 -> [w2205]
                    tunnel: [w2205] -> w2189
                    tunnel: w2191 -> [w2204]
                    tunnel: [w2204] -> w2188
                    tunnel: w2190 -> [w2210]
                    tunnel: w2189 -> [w2209]
                    tunnel: w2188 -> [_]
                    tunnel: [w2208] -> w2187
                    tunnel: [w2207] -> w2186
                    tunnel: w2187 -> [w2216]
                    tunnel: [w2216] -> w2185
                    tunnel: w2186 -> [w2215]
                    tunnel: [w2215] -> w2184
                    tunnel: w2185 -> [w2219]
                    tunnel: w2184 -> [w2218]
                    tunnel: [w2217] -> w2167
                    tunnel: [w2227] -> w2166
                    frame #0 {
                      n1091 = Wait (ms)(milliseconds to wait=u32 50 ("等待时间（毫秒）")) -> ()  [unwired: 1 out]
                    }
                    frame #1 {
                      n1092 = local read "VISA资源名称输出 10"() -> (w2198:refnum<visa-resource-name>)
                      n1093 = Concatenate Strings("SET:GRO 12," ("写入缓冲区"), w2196, "\n") -> (w2199:string)
                      n1094 = VISA Write(VISA resource name=w2198, write buffer=w2199, error in (no error)=w2195) -> (VISA resource name out=w2201:refnum<visa-resource-name>, error out=w2200:errorcluster)  [unwired: 1 out]
                    }
                    frame #2 {
                      n1095 = Wait (ms)(milliseconds to wait=u32 50 ("等待时间（毫秒）")) -> ()  [unwired: 1 out]
                    }
                    frame #3 {
                      n1096 = Concatenate Strings("SET:STE 12" ("写入缓冲区"), "\n") -> (w2211:string)
                      n1097 = VISA Write(VISA resource name=w2210, write buffer=w2211, error in (no error)=w2209) -> (VISA resource name out=w2208:refnum<visa-resource-name>, error out=w2207:errorcluster)  [unwired: 1 out]
                    }
                    frame #4 {
                      n1098 = Wait (ms)(milliseconds to wait=u32 200 ("等待时间（毫秒）")) -> ()  [unwired: 1 out]
                    }
                    frame #5 {
                      n1099 = Concatenate Strings("OUT:ON" ("写入缓冲区"), "\n") -> (w2224:string)
                      n1100 = Wait (ms)(milliseconds to wait=u32 50 ("等待时间（毫秒）")) -> ()  [unwired: 1 out]
                      n1101 = VISA Write(VISA resource name=w2219, write buffer=w2224, error in (no error)=w2218) -> (VISA resource name out=w2221:refnum<visa-resource-name>, error out=w2217:errorcluster)  [unwired: 1 out]
                      n1102 = local write "VISA资源名称输出 10"(w2221) -> ()
                    }
                    frame #6 {
                      n1103 = while {
                        tunnel: [w2232] -> w2227
                        i -> [w2233]
                        stop <- w2231 stop-if-true
                        n1104 = local read "Volt2"() -> (w2237:dbl)
                        n1105 = local read "Actual"() -> (w2238:dbl)
                        n1106 = Greater Or Equal?(x=w2233, y=20) -> (x >= y?=w2235:bool)
                        n1107 = Multiply(x=w2237, y=0.02) -> (x*y=w2239:dbl)
                        n1108 = Add(x=w2237, y=w2239) -> (x+y=w2241:dbl)
                        n1109 = Subtract(x=w2237, y=w2239) -> (x-y=w2240:dbl)
                        n1110 = Wait Until Next ms Multiple(millisecond multiple=u32 200 ("毫秒倍数")) -> ()  [unwired: 1 out]
                        n1111 = In Range and Coerce(upper limit=w2241, x=w2238, lower limit=w2240) -> (In Range?=w2232:bool)  [unwired: 1 out]
                        n1112 = Or(x=w2232, y=w2235) -> (x .or. y?=w2231:bool)
                      }
                      n1113 = case shown="真" w2227 {
                        tunnel: ["300V电压开启NG" "300V电压开启成功"] -> w2226
                        tunnel: [u32 16711680 u32 6618880] -> w2225
                        frame False {
                        }
                        frame True {
                        }
                      }
                      n1114 = control-ref of="结果"() -> (w2229:refnum<vi>)
                      n1115 = Build Array(w2226) -> (w2228:string[])
                      n1116 = local write "控制读取  5"(TRUE ("控制读取")) -> ()
                      n1117 = call "表格编辑.vi"("新元素/子数组"=w2228, "活动单元格:单元格背景色"=w2225, "MCListbox引用句柄"=w2229) -> ()  [unwired: 9 out]
                    }
                  }
                }
                frame 18 {
                  # "300V内总压AD2"
                  n1118 = flat-sequence {
                    tunnel: w2254 -> [w2260]
                    tunnel: w2255 -> [w2261]
                    tunnel: [w2261] -> w2248
                    tunnel: [w2260] -> w2247
                    tunnel: [w2268] -> w2257
                    tunnel: [w2267] -> w2256
                    tunnel: w2248 -> [w2268]
                    tunnel: w2247 -> [w2267]
                    tunnel: w2257 -> [w2273]
                    tunnel: w2256 -> [w2272]
                    tunnel: [w2271] -> w2251
                    tunnel: [w2270] -> w2250
                    tunnel: [w2279] -> w2253
                    tunnel: [w2280] -> w2252
                    tunnel: w2251 -> [w2280]
                    tunnel: w2250 -> [w2279]
                    tunnel: [w2278] -> w2249
                    frame #0 {
                      n1119 = One Button Dialog(message="请把继电器调到\n内总压状态" ("消息"), button name ("OK")="确定" ("按钮名称（“确定”）")) -> ()  [unwired: 1 out]
                    }
                    frame #1 {
                      n1120 = global write "EV05全局变量1.vi" "CAN接收"(FALSE ("CAN接收")) -> ()
                      n1121 = global write "EV05全局变量1.vi" "高压校正接收"(FALSE ("高压校正接收")) -> ()
                      n1122 = local write "AD2"(0.0 ("AD2 2")) -> ()
                      n1123 = property on="Read2_in结果" class="Bool (严格)"("Colors [4]"=cluster{u32, u32}[] [{0, 0}] ("颜色[4]"), "BoolText.Text"="" ("布尔文本.文本")) -> ()  [unwired: 2 in, 2 out]
                    }
                    frame #2 {
                      n1124 = Enqueue Element(queue=w2273, element="Read2_in" ("元素"), error in (no error)=w2272) -> (queue out=w2270:refnum<queue>, error out=w2271:errorcluster)  [unwired: 2 out]
                    }
                    frame #3 {
                      n1125 = while {
                        tunnel: [w2286] -> w2278
                        i -> [w2291]
                        stop <- w2287 stop-if-true
                        n1126 = property on="Read2_in结果" class="Bool (严格)"() -> ("BoolText.Text"=w2285:string)  [unwired: 2 in, 2 out]
                        n1127 = Greater Or Equal?(x=w2291, y=30) -> (x >= y?=w2288:bool)
                        n1128 = Not Equal?(x=w2285, y="NG" ("布尔文本.文本")) -> (x != y?=w2286:bool)
                        n1129 = Or(x=w2286, y=w2288) -> (x .or. y?=w2287:bool)
                        n1130 = Wait Until Next ms Multiple(millisecond multiple=u32 110 ("毫秒倍数")) -> ()  [unwired: 1 out]
                      }
                      n1131 = case shown="真" w2278 {
                        tunnel: ["内总压AD2值读取NG" "内总压AD2值读取成功"] -> w2275
                        tunnel: [u32 16711680 u32 6618880] -> w2274
                        frame False {
                        }
                        frame True {
                        }
                      }
                      n1132 = control-ref of="结果"() -> (w2276:refnum<vi>)
                      n1133 = Build Array(w2275) -> (w2277:string[])
                      n1134 = call "表格编辑.vi"("新元素/子数组"=w2277, "活动单元格:单元格背景色"=w2274, "MCListbox引用句柄"=w2276) -> ()  [unwired: 9 out]
                    }
                  }
                }
                frame 19 {
                  # "300V外总压AD2"
                  n1135 = flat-sequence {
                    tunnel: w2300 -> [w2306]
                    tunnel: w2301 -> [w2307]
                    tunnel: [w2307] -> w2294
                    tunnel: [w2306] -> w2293
                    tunnel: [w2314] -> w2303
                    tunnel: [w2313] -> w2302
                    tunnel: w2294 -> [w2314]
                    tunnel: w2293 -> [w2313]
                    tunnel: w2303 -> [w2319]
                    tunnel: w2302 -> [w2318]
                    tunnel: [w2317] -> w2297
                    tunnel: [w2316] -> w2296
                    tunnel: [w2325] -> w2299
                    tunnel: [w2326] -> w2298
                    tunnel: w2297 -> [w2326]
                    tunnel: w2296 -> [w2325]
                    tunnel: [w2324] -> w2295
                    frame #0 {
                      n1136 = One Button Dialog(message="请把继电器调到\n外总压状态" ("消息"), button name ("OK")="确定" ("按钮名称（“确定”）")) -> ()  [unwired: 1 out]
                    }
                    frame #1 {
                      n1137 = global write "EV05全局变量1.vi" "CAN接收"(FALSE ("CAN接收")) -> ()
                      n1138 = global write "EV05全局变量1.vi" "高压校正接收"(FALSE ("高压校正接收")) -> ()
                      n1139 = local write "AD2"(0.0 ("AD2 3")) -> ()
                      n1140 = property on="Read2_Out结果" class="Bool (严格)"("Colors [4]"=cluster{u32, u32}[] [{0, 0}] ("颜色[4]"), "BoolText.Text"="" ("布尔文本.文本")) -> ()  [unwired: 2 in, 2 out]
                    }
                    frame #2 {
                      n1141 = Enqueue Element(queue=w2319, element="Read1_in" ("元素"), error in (no error)=w2318) -> (queue out=w2316:refnum<queue>, error out=w2317:errorcluster)  [unwired: 2 out]
                    }
                    frame #3 {
                      n1142 = while {
                        tunnel: [w2332] -> w2324
                        i -> [w2337]
                        stop <- w2333 stop-if-true
                        n1143 = property on="Read2_Out结果" class="Bool (严格)"() -> ("BoolText.Text"=w2331:string)  [unwired: 2 in, 2 out]
                        n1144 = Greater Or Equal?(x=w2337, y=30) -> (x >= y?=w2334:bool)
                        n1145 = Not Equal?(x=w2331, y="NG" ("布尔文本.文本")) -> (x != y?=w2332:bool)
                        n1146 = Or(x=w2332, y=w2334) -> (x .or. y?=w2333:bool)
                        n1147 = Wait Until Next ms Multiple(millisecond multiple=u32 110 ("毫秒倍数")) -> ()  [unwired: 1 out]
                      }
                      n1148 = case shown="真" w2324 {
                        tunnel: ["外总压AD2值读取NG" "外总压AD2值读取成功"] -> w2321
                        tunnel: [u32 16711680 u32 6618880] -> w2320
                        frame False {
                        }
                        frame True {
                        }
                      }
                      n1149 = control-ref of="结果"() -> (w2322:refnum<vi>)
                      n1150 = Build Array(w2321) -> (w2323:string[])
                      n1151 = call "表格编辑.vi"("新元素/子数组"=w2323, "活动单元格:单元格背景色"=w2320, "MCListbox引用句柄"=w2322) -> ()  [unwired: 9 out]
                    }
                  }
                }
                frame 20 {
                  # "SET内总压"
                  n1152 = flat-sequence {
                    tunnel: w2344 -> [w2358]
                    tunnel: w2345 -> [w2359]
                    tunnel: [w2359] -> w2347
                    tunnel: [w2358] -> w2346
                    tunnel: w2347 -> [w2364]
                    tunnel: w2346 -> [w2363]
                    tunnel: [w2362] -> w2341
                    tunnel: [w2361] -> w2340
                    tunnel: [w2370] -> w2343
                    tunnel: [w2371] -> w2342
                    tunnel: w2341 -> [w2371]
                    tunnel: w2340 -> [w2370]
                    tunnel: [w2369] -> w2339
                    frame #0 {
                      n1153 = local read "REAL2"() -> (w2356:dbl)
                      n1154 = local read "REAL1"() -> (w2357:dbl)
                      n1155 = local read "AD1"() -> (w2355:dbl)
                      n1156 = local read "AD2"() -> (w2354:dbl)
                      n1157 = global write "EV05全局变量1.vi" "CAN接收"(FALSE ("CAN接收")) -> ()
                      n1158 = global write "EV05全局变量1.vi" "高压校正接收"(FALSE ("高压校正接收")) -> ()
                      n1159 = call "Cal_Gain&offset.vi"("REAL2"=w2356, "REAL1"=w2357, "AD2"=w2354, "AD1"=w2355) -> ("Offset"=w2352:i32, "Gain"=w2353:dbl)  [unwired: 5 out]
                      n1160 = local write "Offset"(w2352) -> ()
                      n1161 = local write "Gain"(w2353) -> ()
                      n1162 = property on="Set_in结果" class="Bool (严格)"("Colors [4]"=cluster{u32, u32}[] [{0, 0}] ("颜色[4]"), "BoolText.Text"="" ("布尔文本.文本")) -> ()  [unwired: 2 in, 2 out]
                    }
                    frame #1 {
                      n1163 = Enqueue Element(queue=w2364, element="Set_in" ("元素"), error in (no error)=w2363) -> (queue out=w2361:refnum<queue>, error out=w2362:errorcluster)  [unwired: 2 out]
                    }
                    frame #2 {
                      n1164 = while {
                        tunnel: [w2377] -> w2369
                        i -> [w2382]
                        stop <- w2378 stop-if-true
                        n1165 = property on="Set_in结果" class="Bool (严格)"() -> ("BoolText.Text"=w2376:string)  [unwired: 2 in, 2 out]
                        n1166 = Greater Or Equal?(x=w2382, y=30) -> (x >= y?=w2379:bool)
                        n1167 = Not Equal?(x=w2376, y="NG" ("布尔文本.文本")) -> (x != y?=w2377:bool)
                        n1168 = Or(x=w2377, y=w2379) -> (x .or. y?=w2378:bool)
                        n1169 = Wait Until Next ms Multiple(millisecond multiple=u32 110 ("毫秒倍数")) -> ()  [unwired: 1 out]
                      }
                      n1170 = case shown="真" w2369 {
                        tunnel: ["内总压参数写入NG" "内总压参数写入成功"] -> w2365
                        tunnel: [u32 16711680 u32 6618880] -> w2366
                        frame False {
                        }
                        frame True {
                        }
                      }
                      n1171 = control-ref of="结果"() -> (w2367:refnum<vi>)
                      n1172 = Build Array(w2365) -> (w2368:string[])
                      n1173 = call "表格编辑.vi"("新元素/子数组"=w2368, "活动单元格:单元格背景色"=w2366, "MCListbox引用句柄"=w2367) -> ()  [unwired: 9 out]
                    }
                  }
                }
                frame 21 {
                  # "SET外总压"
                  n1174 = flat-sequence {
                    tunnel: w2389 -> [w2403]
                    tunnel: w2390 -> [w2404]
                    tunnel: [w2404] -> w2392
                    tunnel: [w2403] -> w2391
                    tunnel: w2392 -> [w2409]
                    tunnel: w2391 -> [w2408]
                    tunnel: [w2407] -> w2386
                    tunnel: [w2406] -> w2385
                    tunnel: [w2415] -> w2388
                    tunnel: [w2416] -> w2387
                    tunnel: w2386 -> [w2416]
                    tunnel: w2385 -> [w2415]
                    tunnel: [w2414] -> w2384
                    frame #0 {
                      n1175 = local read "REAL2"() -> (w2396:dbl)
                      n1176 = local read "REAL1"() -> (w2395:dbl)
                      n1177 = local read "AD1"() -> (w2397:dbl)
                      n1178 = local read "AD2"() -> (w2398:dbl)
                      n1179 = global write "EV05全局变量1.vi" "CAN接收"(FALSE ("CAN接收")) -> ()
                      n1180 = global write "EV05全局变量1.vi" "高压校正接收"(FALSE ("高压校正接收")) -> ()
                      n1181 = call "Cal_Gain&offset.vi"("REAL2"=w2396, "REAL1"=w2395, "AD2"=w2398, "AD1"=w2397) -> ("Offset"=w2399:i32, "Gain"=w2400:dbl)  [unwired: 5 out]
                      n1182 = local write "Gain"(w2400) -> ()
                      n1183 = local write "Offset"(w2399) -> ()
                      n1184 = property on="Set_out结果" class="Bool (严格)"("Colors [4]"=cluster{u32, u32}[] [{0, 0}] ("颜色[4]"), "BoolText.Text"="" ("布尔文本.文本")) -> ()  [unwired: 2 in, 2 out]
                    }
                    frame #1 {
                      n1185 = Enqueue Element(queue=w2409, element="Set_out" ("元素"), error in (no error)=w2408) -> (queue out=w2406:refnum<queue>, error out=w2407:errorcluster)  [unwired: 2 out]
                    }
                    frame #2 {
                      n1186 = while {
                        tunnel: [w2422] -> w2414
                        i -> [w2427]
                        stop <- w2423 stop-if-true
                        n1187 = property on="Set_out结果" class="Bool (严格)"() -> ("BoolText.Text"=w2421:string)  [unwired: 2 in, 2 out]
                        n1188 = Greater Or Equal?(x=w2427, y=30) -> (x >= y?=w2424:bool)
                        n1189 = Not Equal?(x=w2421, y="NG" ("布尔文本.文本")) -> (x != y?=w2422:bool)
                        n1190 = Or(x=w2422, y=w2424) -> (x .or. y?=w2423:bool)
                        n1191 = Wait Until Next ms Multiple(millisecond multiple=u32 110 ("毫秒倍数")) -> ()  [unwired: 1 out]
                      }
                      n1192 = case shown="假" w2414 {
                        tunnel: ["外总压参数写入NG" "外总压参数写入成功"] -> w2410
                        tunnel: [u32 16711680 u32 6618880] -> w2411
                        frame False {
                        }
                        frame True {
                        }
                      }
                      n1193 = control-ref of="结果"() -> (w2412:refnum<vi>)
                      n1194 = Build Array(w2410) -> (w2413:string[])
                      n1195 = call "表格编辑.vi"("新元素/子数组"=w2413, "活动单元格:单元格背景色"=w2411, "MCListbox引用句柄"=w2412) -> ()  [unwired: 9 out]
                    }
                  }
                }
                frame 22 {
                  w2456 = "," ("字符串")
                  # "检验电压校正状态"
                  n1196 = flat-sequence {
                    tunnel: [w2481] -> w2436
                    tunnel: [w2472] -> w2429
                    tunnel: [w2490] -> w2437
                    tunnel: w2436 -> [w2490]
                    tunnel: [w2489] -> w2430
                    tunnel: w2429 -> [w2489]
                    tunnel: [w2500] -> w2471
                    tunnel: [w2499] -> w2470
                    tunnel: [w2498] -> w2469
                    tunnel: w2455 -> [w2495]
                    tunnel: w2447 -> [w2494]
                    tunnel: [w2493] -> w2438
                    tunnel: w2437 -> [w2493]
                    tunnel: [w2492] -> w2431
                    tunnel: w2430 -> [w2492]
                    tunnel: w2471 -> [w2507]
                    tunnel: [w2507] -> w2468
                    tunnel: w2470 -> [w2506]
                    tunnel: [w2506] -> w2467
                    tunnel: w2469 -> [w2505]
                    tunnel: [w2505] -> w2466
                    tunnel: [w2503] -> w2439
                    tunnel: w2438 -> [w2503]
                    tunnel: [w2502] -> w2432
                    tunnel: w2431 -> [w2502]
                    tunnel: w2468 -> [w2513]
                    tunnel: w2467 -> [w2512]
                    tunnel: w2466 -> [_]
                    tunnel: [w2511] -> w2465
                    tunnel: [w2510] -> w2464
                    tunnel: [w2509] -> w2440
                    tunnel: w2439 -> [w2509]
                    tunnel: [w2508] -> w2433
                    tunnel: w2432 -> [w2508]
                    tunnel: w2465 -> [w2521]
                    tunnel: [w2521] -> w2463
                    tunnel: w2464 -> [w2520]
                    tunnel: [w2520] -> w2462
                    tunnel: [w2518] -> w2441
                    tunnel: w2440 -> [w2518]
                    tunnel: [w2517] -> w2434
                    tunnel: w2433 -> [w2517]
                    tunnel: w2463 -> [w2526]
                    tunnel: w2462 -> [w2525]
                    tunnel: [w2524] -> w2445
                    tunnel: [w2523] -> w2442
                    tunnel: w2441 -> [w2523]
                    tunnel: [w2522] -> w2435
                    tunnel: w2434 -> [w2522]
                    tunnel: [w2532] -> w2444
                    tunnel: w2442 -> [w2534]
                    tunnel: w2435 -> [w2533]
                    frame #0 {
                      n1197 = local read "SumV_out"() -> (w2475:dbl)
                      n1198 = local read "SumV_in"() -> (w2482:dbl)
                      n1199 = local read "Actual"() -> (w2474:dbl)
                      n1200 = Subtract(x=w2482, y=w2474) -> (x-y=w2487:dbl)
                      n1201 = Subtract(x=w2474, y=w2475) -> (x-y=w2477:dbl)
                      n1202 = Absolute Value(x=w2487) -> (abs(x)=w2488:dbl)
                      n1203 = Absolute Value(x=w2477) -> (abs(x)=w2476:dbl)
                      n1204 = Divide(x=w2488, y=w2474) -> (x/y=w2484:dbl)
                      n1205 = Divide(x=w2476, y=w2474) -> (x/y=w2480:dbl)
                      n1206 = Multiply(x=w2484, y=100.0) -> (x*y=w2485:dbl)
                      n1207 = Multiply(x=w2480, y=100.0) -> (x*y=w2479:dbl)
                      n1208 = Format Into String(format string="%.3f%" ("格式字符串"), w2485) -> (resulting string=w2481:string)  [unwired: 2 in, 1 out]
                      n1209 = Format Into String(format string="%.3f%" ("格式字符串"), w2479) -> (resulting string=w2472:string)  [unwired: 2 in, 1 out]
                    }
                    frame #1 {
                      n1210 = Wait (ms)(milliseconds to wait=u32 50 ("等待时间（毫秒）")) -> ()  [unwired: 1 out]
                    }
                    frame #2 {
                      n1211 = local read "VISA资源名称输出 10"() -> (w2497:refnum<visa-resource-name>)
                      n1212 = Concatenate Strings("SET:GRO 12," ("写入缓冲区"), w2495, "\n") -> (w2498:string)
                      n1213 = VISA Write(VISA resource name=w2497, write buffer=w2498, error in (no error)=w2494) -> (VISA resource name out=w2500:refnum<visa-resource-name>, error out=w2499:errorcluster)  [unwired: 1 out]
                    }
                    frame #3 {
                      n1214 = Wait (ms)(milliseconds to wait=u32 50 ("等待时间（毫秒）")) -> ()  [unwired: 1 out]
                    }
                    frame #4 {
                      n1215 = Concatenate Strings("SET:STE 12" ("写入缓冲区"), "\n") -> (w2514:string)
                      n1216 = VISA Write(VISA resource name=w2513, write buffer=w2514, error in (no error)=w2512) -> (VISA resource name out=w2511:refnum<visa-resource-name>, error out=w2510:errorcluster)  [unwired: 1 out]
                    }
                    frame #5 {
                      n1217 = Wait (ms)(milliseconds to wait=u32 200 ("等待时间（毫秒）")) -> ()  [unwired: 1 out]
                    }
                    frame #6 {
                      n1218 = Concatenate Strings("OUT:ON" ("写入缓冲区"), "\n") -> (w2531:string)
                      n1219 = Wait (ms)(milliseconds to wait=u32 50 ("等待时间（毫秒）")) -> ()  [unwired: 1 out]
                      n1220 = VISA Write(VISA resource name=w2526, write buffer=w2531, error in (no error)=w2525) -> (VISA resource name out=w2528:refnum<visa-resource-name>, error out=w2524:errorcluster)  [unwired: 1 out]
                      n1221 = local write "VISA资源名称输出 10"(w2528) -> ()
                    }
                    frame #7 {
                      n1222 = stacked-sequence {
                        seq-local: [w2535 _ _ _] -> [_ w2548 _ _]
                        tunnel: w2534 -> [_ _ w2559 _]
                        tunnel: w2533 -> [_ _ _ w2575]
                        tunnel: [w2535 _ _ _] -> w2532
                        frame #0 {
                          n1223 = while {
                            tunnel: [w2538] -> w2535
                            i -> [w2539]
                            stop <- w2537 stop-if-true
                            w2536 = 150.0 ("x")
                            n1224 = local read "Actual"() -> (w2543:dbl)
                            n1225 = Greater Or Equal?(x=w2539, y=20) -> (x >= y?=w2541:bool)
                            n1226 = Multiply(x=w2536, y=0.02) -> (x*y=w2544:dbl)
                            n1227 = Add(x=w2536, y=w2544) -> (x+y=w2546:dbl)
                            n1228 = Subtract(x=w2536, y=w2544) -> (x-y=w2545:dbl)
                            n1229 = Wait Until Next ms Multiple(millisecond multiple=u32 200 ("毫秒倍数")) -> ()  [unwired: 1 out]
                            n1230 = In Range and Coerce(upper limit=w2546, x=w2543, lower limit=w2545) -> (In Range?=w2538:bool)  [unwired: 1 out]
                            n1231 = Or(x=w2538, y=w2541) -> (x .or. y?=w2537:bool)
                          }
                        }
                        frame #1 {
                          n1232 = case shown="假" w2548 {
                            tunnel: ["150V电压开启NG" "150V电压开启成功"] -> w2550
                            tunnel: [u32 16711680 u32 6618880] -> w2549
                            frame False {
                            }
                            frame True {
                            }
                          }
                          n1233 = control-ref of="结果"() -> (w2552:refnum<vi>)
                          n1234 = Build Array(w2550) -> (w2551:string[])
                          n1235 = call "表格编辑.vi"("新元素/子数组"=w2551, "活动单元格:单元格背景色"=w2549, "MCListbox引用句柄"=w2552) -> ()  [unwired: 9 out]
                        }
                        frame #2 {
                          n1236 = local read "SumV_in"() -> (w2560:dbl)
                          n1237 = local read "Actual"() -> (w2561:dbl)
                          n1238 = Subtract(x=w2561, y=w2560) -> (x-y=w2569:dbl)
                          n1239 = Absolute Value(x=w2569) -> (abs(x)=w2570:dbl)
                          n1240 = Divide(x=w2570, y=w2561) -> (x/y=w2565:dbl)
                          n1241 = Multiply(x=w2565, y=100.0) -> (x*y=w2566:dbl)
                          n1242 = Format Into String(format string="%.3f%" ("格式字符串"), w2566) -> (resulting string=w2558:string)  [unwired: 2 in, 1 out]
                          n1243 = Concatenate Strings("内总压150V误差", w2558, "  300V误差", w2559) -> (w2562:string)
                          n1244 = control-ref of="结果"() -> (w2572:refnum<vi>)
                          n1245 = local write "控制读取  5"(TRUE ("控制读取")) -> ()
                          n1246 = Build Array(w2562) -> (w2571:string[])
                          n1247 = call "表格编辑.vi"("新元素/子数组"=w2571, "活动单元格:单元格背景色"=u32 6618880, "MCListbox引用句柄"=w2572) -> ()  [unwired: 9 out]
                        }
                        frame #3 {
                          n1248 = local read "Actual"() -> (w2578:dbl)
                          n1249 = local read "SumV_out"() -> (w2576:dbl)
                          n1250 = Subtract(x=w2578, y=w2576) -> (x-y=w2586:dbl)
                          n1251 = Absolute Value(x=w2586) -> (abs(x)=w2587:dbl)
                          n1252 = Divide(x=w2587, y=w2578) -> (x/y=w2582:dbl)
                          n1253 = Multiply(x=w2582, y=100.0) -> (x*y=w2583:dbl)
                          n1254 = Format Into String(format string="%.3f%" ("格式字符串"), w2583) -> (resulting string=w2577:string)  [unwired: 2 in, 1 out]
                          n1255 = Concatenate Strings("外总压150V误差", w2577, "  300V误差", w2575) -> (w2579:string)
                          n1256 = control-ref of="结果"() -> (w2589:refnum<vi>)
                          n1257 = Build Array(w2579) -> (w2588:string[])
                          n1258 = call "表格编辑.vi"("新元素/子数组"=w2588, "活动单元格:单元格背景色"=u32 6618880, "MCListbox引用句柄"=w2589) -> ()  [unwired: 9 out]
                        }
                      }
                    }
                  }
                  n1259 = Number To Fractional String(number=150.0 ("数字"), precision (6)=i16 2 ("精度(6)")) -> (F-format string=w2460:string)  [unwired: 2 out]
                  n1260 = Number To Fractional String(number=0.2 ("数字"), precision (6)=i16 2 ("精度(6)")) -> (F-format string=w2459:string)  [unwired: 2 out]
                  n1261 = Number To Fractional String(number=320.0 ("数字"), precision (6)=i16 2 ("精度(6)")) -> (F-format string=w2458:string)  [unwired: 2 out]
                  n1262 = Number To Fractional String(number=1.0 ("数字"), precision (6)=i16 2 ("精度(6)")) -> (F-format string=w2457:string)  [unwired: 2 out]
                  n1263 = Concatenate Strings(w2460, w2456, w2459, w2456, w2458, w2456, w2457, w2456, w2456, w2456) -> (w2455:string)
                  n1264 = local write "控制读取  5"(FALSE ("控制读取")) -> ()
                }
                frame 23 {
                  # "关闭电压源"
                  n1265 = local read "VISA资源名称输出 10"() -> (w2596:refnum<visa-resource-name>)
                  n1266 = local write "控制读取  5"(FALSE ("控制读取")) -> ()
                  n1267 = flat-sequence {
                    tunnel: [w2603] -> w2601
                    tunnel: w2596 -> [w2603]
                    tunnel: w2601 -> [w2607]
                    tunnel: [w2606] -> w2600
                    tunnel: [w2605] -> w2599
                    tunnel: w2594 -> [w2604]
                    tunnel: w2600 -> [w2611]
                    tunnel: w2599 -> [w2610]
                    tunnel: [w2611] -> w2598
                    tunnel: [w2610] -> w2597
                    tunnel: w2598 -> [w2615]
                    tunnel: w2597 -> [w2614]
                    tunnel: [w2612] -> w2591
                    tunnel: [w2622] -> w2593
                    tunnel: w2591 -> [w2622]
                    tunnel: [FALSE ("status")] -> w2590
                    frame #0 {
                      n1268 = Wait (ms)(milliseconds to wait=u32 50 ("等待时间（毫秒）")) -> ()  [unwired: 1 out]
                    }
                    frame #1 {
                      n1269 = VISA Write(VISA resource name=w2607, write buffer="OUT:OFF" ("写入缓冲区"), error in (no error)=w2604) -> (VISA resource name out=w2606:refnum<visa-resource-name>, error out=w2605:errorcluster)  [unwired: 1 out]
                    }
                    frame #2 {
                      n1270 = Wait (ms)(milliseconds to wait=u32 50 ("等待时间（毫秒）")) -> ()  [unwired: 1 out]
                    }
                    frame #3 {
                      n1271 = local write "控制读取  5"(TRUE ("控制读取")) -> ()
                      n1272 = VISA Write(VISA resource name=w2615, write buffer="OUT:OFF" ("写入缓冲区"), error in (no error)=w2614) -> (error out=w2612:errorcluster)  [unwired: 2 out]
                    }
                    frame #4 {
                      n1273 = control-ref of="结果"() -> (w2619:refnum<vi>)
                      n1274 = Build Array("电压源关闭") -> (w2620:string[])
                      n1275 = call "表格编辑.vi"("新元素/子数组"=w2620, "活动单元格:单元格背景色"=u32 6618880, "MCListbox引用句柄"=w2619) -> ()  [unwired: 9 out]
                    }
                  }
                }
                frame 24 {
                  # "分流器型号"
                  n1276 = local read "分流器大小"() -> (w2628:T2)
                  n1277 = case shown="\"100A\", 默认" w2628 {
                    selector: w2628 -> [_ w2635]
                    tunnel: w2627 -> [w2633 w2642]
                    tunnel: w2626 -> [w2632 w2641]
                    tunnel: [w2632 w2640] -> w2624
                    tunnel: [w2633 w2639] -> w2625
                    tunnel: [TRUE ("status") w2636] -> w2623
                    frame "选择分流器型号" {
                      n1278 = One Button Dialog(message="分流器为无效值" ("消息"), button name ("OK")="确定" ("按钮名称（“确定”）")) -> ()  [unwired: 1 out]
                    }
                    frame "100A", Default {
                      n1279 = flat-sequence {
                        tunnel: w2641 -> [w2659]
                        tunnel: w2642 -> [w2660]
                        tunnel: [w2660] -> w2644
                        tunnel: [w2659] -> w2643
                        tunnel: w2644 -> [w2665]
                        tunnel: w2643 -> [w2664]
                        tunnel: [w2663] -> w2638
                        tunnel: [w2662] -> w2637
                        tunnel: [w2673] -> w2639
                        tunnel: [w2674] -> w2640
                        tunnel: w2638 -> [w2674]
                        tunnel: w2637 -> [w2673]
                        tunnel: [TRUE ("status")] -> w2636
                        tunnel: w2634 -> [w2666]
                        frame #0 {
                          n1280 = global write "EV05全局变量1.vi" "CAN接收"(FALSE ("CAN接收")) -> ()
                          n1281 = global write "EV05全局变量1.vi" "高压校正接收"(FALSE ("高压校正接收")) -> ()
                          n1282 = property on="Current Gain结果 4" class="Bool (严格)"("Colors [4]"=cluster{u32, u32}[] [{0, 0}] ("颜色[4]"), "BoolText.Text"="" ("布尔文本.文本")) -> ()  [unwired: 2 in, 2 out]
                        }
                        frame #1 {
                          n1283 = Enqueue Element(queue=w2665, element="Set Current Gain 4" ("元素"), error in (no error)=w2664) -> (queue out=w2662:refnum<queue>, error out=w2663:errorcluster)  [unwired: 2 out]
                        }
                        frame #2 {
                          n1284 = while {
                            tunnel: [w2686] -> w2668
                            i -> [w2691]
                            stop <- w2687 stop-if-true
                            n1285 = property on="Current Gain结果 4" class="Bool (严格)"() -> ("BoolText.Text"=w2685:string)  [unwired: 2 in, 2 out]
                            n1286 = Greater Or Equal?(x=w2691, y=30) -> (x >= y?=w2688:bool)
                            n1287 = Not Equal?(x=w2685, y="NG" ("布尔文本.文本")) -> (x != y?=w2686:bool)
                            n1288 = Or(x=w2686, y=w2688) -> (x .or. y?=w2687:bool)
                            n1289 = Wait Until Next ms Multiple(millisecond multiple=u32 110 ("毫秒倍数")) -> ()  [unwired: 1 out]
                          }
                          n1290 = case shown="假" w2668 {
                            tunnel: [w2675 w2680] -> w2669
                            tunnel: [u32 16711680 u32 6618880] -> w2670
                            tunnel: w2666 -> [w2677 w2682]
                            frame False {
                              n1291 = Concatenate Strings("分流器", w2677, " 写入NG") -> (w2675:string)
                            }
                            frame True {
                              n1292 = Concatenate Strings("分流器", w2682, " 写入成功") -> (w2680:string)
                            }
                          }
                          n1293 = control-ref of="结果"() -> (w2671:refnum<vi>)
                          n1294 = Build Array(w2669) -> (w2672:string[])
                          n1295 = call "表格编辑.vi"("新元素/子数组"=w2672, "活动单元格:单元格背景色"=w2670, "MCListbox引用句柄"=w2671) -> ()  [unwired: 9 out]
                        }
                      }
                      n1296 = case shown="\"100A\", 默认" w2635 {
                        tunnel: ["100A" "200A" "300A" "400A" "500A" "600A" "700A" "800A" "900A" "1000A"] -> w2634
                        frame "100A", Default {
                        }
                        frame "200A" {
                        }
                        frame "300A" {
                        }
                        frame "400A" {
                        }
                        frame "500A" {
                        }
                        frame "600A" {
                        }
                        frame "700A" {
                        }
                        frame "800A" {
                        }
                        frame "900A" {
                        }
                        frame "1000A" {
                        }
                      }
                    }
                  }
                }
              }
              n1297 = call <vilib>:"Set Busy.vi"() -> ()  [unwired: 10 in, 2 out]
              n1298 = case shown="假" w1282 {
                tunnel: ["校正完成" "校正NG"] -> w1279
                tunnel: [u32 6618880 u32 16711680] -> w1278
                frame False {
                  n1299 = call <vilib>:"Unset Busy.vi"() -> ()  [unwired: 11 in, 1 out]
                }
                frame True {
                }
              }
              n1300 = control-ref of="结果"() -> (w1281:refnum<vi>)
              n1301 = Build Array(w1279) -> (w1280:string[])
              n1302 = call "表格编辑.vi"("新元素/子数组"=w1280, "活动单元格:单元格背景色"=w1278, "MCListbox引用句柄"=w1281) -> ()  [unwired: 9 out]
            }
          }
        }
      }
      event "记录": Value Change {
        n1303 = event-data() -> ("NewVal"=w2693:bool)  [unwired: 6 out]
        n1304 = case shown="真" w2693 {
          frame False {
          }
          frame True {
            n1305 = call "当前时间解析-8.6.vi"() -> ("名称格式时间"=w2704:string)  [unwired: 1 in, 18 out]
            n1306 = call <vilib>:"Application Directory.vi"() -> ("Application Directory"=w2694:path)
            n1307 = Concatenate Strings(w2704, ".ini" ("字符串")) -> (w2708:string)
            n1308 = call "路径分析-8.6.vi"("第二个文件夹"="高压校正数据" ("第一个文件夹"), "第一个文件夹"="SaveData", "输入路径"=w2694) -> ("输出路径"=w2706:path)  [unwired: 8 in]
            n1309 = stacked-sequence {
              tunnel: [_ w2745 _] -> w2697
              tunnel: [_ _ w2762] -> w2696
              tunnel: [w2718 _ _] -> w2698
              frame #0 {
                n1310 = local read "REAL2"() -> (w2721:dbl)
                n1311 = local read "REAL1"() -> (w2719:dbl)
                n1312 = local read "Shunt Volt Offset"() -> (w2724:string)
                n1313 = local read "Gain"() -> (w2730:dbl)
                n1314 = local read "分流器大小"() -> (w2731:T2)
                n1315 = local read "AD1"() -> (w2720:u16)
                n1316 = local read "AD2"() -> (w2722:u16)
                n1317 = local read "Shunt Volt Gain"() -> (w2723:string)
                n1318 = local read "电流零点"() -> (w2726:string)
                n1319 = local read "电流增益"() -> (w2725:string)
                n1320 = Build Array(w2719, w2720, w2721, w2722, w2730) -> (w2729:dbl[])
                n1321 = case shown="\"100A\", 默认" w2731 {
                  tunnel: ["100A" "200A" "300A" "400A" "500A" "600A" "700A" "800A" "900A" "1000A"] -> w2727
                  frame "100A", Default {
                  }
                  frame "200A" {
                  }
                  frame "300A" {
                  }
                  frame "400A" {
                  }
                  frame "500A" {
                  }
                  frame "600A" {
                  }
                  frame "700A" {
                  }
                  frame "800A" {
                  }
                  frame "900A" {
                  }
                  frame "1000A" {
                  }
                }
                n1322 = for {
                  tunnel: w2729 -> [w2733] mode=indexing
                  tunnel: [w2732] -> w2728 mode=indexing
                  n1323 = Format Into String(format string="%#f" ("格式字符串"), w2733) -> (resulting string=w2732:string)  [unwired: 2 in, 1 out]
                }
                n1324 = Build Array (concatenate)(w2726, w2725, w2724, w2723, w2727, w2728) -> (w2718:string[])
              }
              frame #1 {
                n1325 = local read "Offset"() -> (w2746:i32)
                n1326 = local read "REAL1"() -> (w2751:dbl)
                n1327 = local read "REAL2"() -> (w2749:dbl)
                n1328 = local read "Gain"() -> (w2747:dbl)
                n1329 = local read "AD1"() -> (w2750:dbl)
                n1330 = local read "AD2"() -> (w2748:dbl)
                n1331 = Build Array(w2751, w2750, w2749, w2748, w2747, w2746) -> (w2752:dbl[])
                n1332 = for {
                  tunnel: w2752 -> [w2754] mode=indexing
                  tunnel: [w2753] -> w2745 mode=indexing
                  n1333 = Format Into String(format string="%#f" ("格式字符串"), w2754) -> (resulting string=w2753:string)  [unwired: 2 in, 1 out]
                }
              }
              frame #2 {
                n1334 = local read "Offset"() -> (w2756:i32)
                n1335 = local read "REAL1"() -> (w2761:dbl)
                n1336 = local read "REAL2"() -> (w2759:dbl)
                n1337 = local read "Gain"() -> (w2757:dbl)
                n1338 = local read "AD1"() -> (w2760:dbl)
                n1339 = local read "AD2"() -> (w2758:dbl)
                n1340 = Build Array(w2761, w2760, w2759, w2758, w2757, w2756) -> (w2763:dbl[])
                n1341 = for {
                  tunnel: w2763 -> [w2765] mode=indexing
                  tunnel: [w2764] -> w2762 mode=indexing
                  n1342 = Format Into String(format string="%#f" ("格式字符串"), w2765) -> (resulting string=w2764:string)  [unwired: 2 in, 1 out]
                }
              }
            }
            n1343 = Build Path(base path=w2706, name or relative path=w2708) -> (appended path=w2703:path)
            n1344 = call <vilib>:"Open Config Data.vi"("configuration file path"=w2703) -> ("refnum"=w2702:T13)  [unwired: 8 in, 2 out]
            n1345 = Build Array(w2698, w2697, w2696) -> (w2695:string[][])
            n1346 = for {
              tunnel: w2702 -> [w2771]
              tunnel: string[] ["Current Gain", "SumV in", "SumV Out"] -> [w2770] mode=indexing
              tunnel: string[][] [["Shunt Current Offset", "Shunt Current Gain", "Shunt Volt Offset", "Shunt Volt Gain", "Shunt Type", "REAL1", "AD1", "REAL2", "AD2", "Gain"], ["REAL1", "AD1", "REAL2", "AD2", "Gain", "Offset", "", "", "", ""], ["REAL1", "AD1", "REAL2", "AD2", "Gain", "Offset", "", "", "", ""]] -> [w2769] mode=indexing
              tunnel: [w2768] -> w2699
              tunnel: w2695 -> [w2767] mode=indexing
              n1347 = for {
                tunnel: w2771 -> [w2776]
                tunnel: w2770 -> [w2775]
                tunnel: w2769 -> [w2774] mode=indexing
                tunnel: [w2773] -> w2768
                tunnel: w2767 -> [w2772] mode=indexing
                n1348 = call-poly <vilib>:"Write Key.vi"("section"=w2775, "value"=w2772, "key"=w2774, "refnum"=w2776) -> ("refnum out"=w2773:T13)  [unwired: 5 in, 2 out]
              }
            }
            n1349 = stacked-sequence {
              tunnel: w2699 -> [w2717]
              frame #0 {
                n1350 = call <vilib>:"Close Config Data.vi"("refnum"=w2717) -> ("file path"=w2713:path)  [unwired: 9 in, 1 out]
                n1351 = Path To String(path=w2713) -> (string=w2712:string)
                n1352 = control-ref of="结果"() -> (w2715:refnum<vi>)
                n1353 = Concatenate Strings("记录完成,路径为:" ("字符串"), w2712) -> (w2710:string)
                n1354 = Build Array(w2710) -> (w2716:string[])
                n1355 = call "表格编辑.vi"("新元素/子数组"=w2716, "活动单元格:单元格背景色"=u32 6618880, "MCListbox引用句柄"=w2715) -> ()  [unwired: 9 out]
              }
            }
          }
        }
      }
      event "输出自定义值1 2": Value Change {
        n1356 = event-data() -> ("NewVal"=w2779:bool)  [unwired: 6 out]
        n1357 = case shown="假" w2779 {
          tunnel: w2778 -> [w2783 w2810]
          tunnel: [w2780 w2808] -> w2777
          frame False {
            w2784 = u8 0 ("禁用")
            n1358 = local read "VISA资源名称输出"() -> (w2789:refnum<visa-resource-name>)
            n1359 = local write "控制读取  2"(FALSE ("控制读取")) -> ()
            n1360 = flat-sequence {
              tunnel: [w2792] -> w2790
              tunnel: w2789 -> [w2792]
              tunnel: w2790 -> [w2796]
              tunnel: [w2795] -> w2787
              tunnel: w2783 -> [w2794]
              tunnel: [w2793] -> w2781
              tunnel: w2787 -> [w2800]
              tunnel: [w2800] -> w2786
              tunnel: [w2798] -> w2782
              tunnel: w2781 -> [w2798]
              tunnel: [w2804] -> w2788
              tunnel: w2786 -> [w2805]
              tunnel: w2782 -> [w2802]
              tunnel: [w2801] -> w2780
              frame #0 {
                n1361 = Wait (ms)(milliseconds to wait=u32 200 ("等待时间（毫秒）")) -> ()  [unwired: 1 out]
              }
              frame #1 {
                n1362 = VISA Write(VISA resource name=w2796, write buffer="outp off" ("写入缓冲区"), error in (no error)=w2794) -> (VISA resource name out=w2795:refnum<visa-resource-name>, error out=w2793:errorcluster)  [unwired: 1 out]
              }
              frame #2 {
                n1363 = Wait (ms)(milliseconds to wait=u32 50 ("等待时间（毫秒）")) -> ()  [unwired: 1 out]
              }
              frame #3 {
                n1364 = local write "控制读取  2"(TRUE ("控制读取")) -> ()
                n1365 = VISA Write(VISA resource name=w2805, write buffer="outp off" ("写入缓冲区"), error in (no error)=w2802) -> (VISA resource name out=w2804:refnum<visa-resource-name>, error out=w2801:errorcluster)  [unwired: 1 out]
              }
            }
            n1366 = local write "VISA资源名称输出"(w2788) -> ()
            n1367 = property on="输出100A" class="Bool"("Disabled"=w2784) -> ()  [unwired: 2 in, 2 out]
            n1368 = property on="输出200A" class="Bool"("Disabled"=w2784) -> ()  [unwired: 2 in, 2 out]
            n1369 = property on="输出自定义值2 2" class="Bool"("Disabled"=w2784) -> ()  [unwired: 2 in, 2 out]
            n1370 = property on="输出自定义值1 2" class="Bool"("Disabled"=w2784) -> ()  [unwired: 2 in, 2 out]
          }
          frame True {
            w2813 = u8 2 ("禁用")
            n1371 = property on="输出200A" class="Bool"("Disabled"=w2813) -> ()  [unwired: 2 in, 2 out]
            n1372 = property on="输出100A" class="Bool"("Disabled"=w2813) -> ()  [unwired: 2 in, 2 out]
            n1373 = property on="输出自定义值2 2" class="Bool"("Disabled"=w2813) -> ()  [unwired: 2 in, 2 out]
            n1374 = local read "Curr1"() -> (w2807:dbl)
            n1375 = flat-sequence {
              tunnel: FALSE ("控制读取") -> [w2823]
              tunnel: [w2833] -> w2818
              tunnel: [w2832] -> w2816
              tunnel: [w2826] -> w2811
              tunnel: w2810 -> [w2825]
              tunnel: w2818 -> [w2837]
              tunnel: [w2837] -> w2817
              tunnel: w2816 -> [w2836]
              tunnel: [w2836] -> w2815
              tunnel: [w2834] -> w2812
              tunnel: w2811 -> [w2834]
              tunnel: w2817 -> [w2842]
              tunnel: w2815 -> [w2841]
              tunnel: [w2840] -> w2822
              tunnel: [w2839] -> w2820
              tunnel: w2812 -> [w2838]
              tunnel: w2822 -> [w2845]
              tunnel: [w2845] -> w2821
              tunnel: w2820 -> [w2844]
              tunnel: [w2844] -> w2819
              tunnel: w2821 -> [w2849]
              tunnel: w2819 -> [w2848]
              tunnel: [w2846] -> w2809
              tunnel: w2809 -> [w2852]
              tunnel: [w2852] -> w2808
              frame #0 {
                n1376 = local write "控制读取  2"(w2823) -> ()
              }
              frame #1 {
                n1377 = Wait (ms)(milliseconds to wait=u32 50 ("等待时间（毫秒）")) -> ()  [unwired: 1 out]
              }
              frame #2 {
                n1378 = local read "VISA资源名称输出"() -> (w2831:refnum<visa-resource-name>)
                n1379 = local read "Curr1"() -> (w2829:dbl)
                n1380 = Number To Fractional String(number=w2829, precision (6)=i16 3 ("精度(6)")) -> (F-format string=w2827:string)  [unwired: 2 out]
                n1381 = Concatenate Strings("volt 1;curr " ("写入缓冲区"), w2827) -> (w2826:string)
                n1382 = VISA Write(VISA resource name=w2831, write buffer=w2826, error in (no error)=w2825) -> (VISA resource name out=w2833:refnum<visa-resource-name>, error out=w2832:errorcluster)  [unwired: 1 out]
              }
              frame #3 {
                n1383 = Wait (ms)(milliseconds to wait=u32 50 ("等待时间（毫秒）")) -> ()  [unwired: 1 out]
              }
              frame #4 {
                n1384 = VISA Write(VISA resource name=w2842, write buffer=w2838, error in (no error)=w2841) -> (VISA resource name out=w2840:refnum<visa-resource-name>, error out=w2839:errorcluster)  [unwired: 1 out]
              }
              frame #5 {
                n1385 = Wait (ms)(milliseconds to wait=u32 200 ("等待时间（毫秒）")) -> ()  [unwired: 1 out]
              }
              frame #6 {
                n1386 = Wait (ms)(milliseconds to wait=u32 50 ("等待时间（毫秒）")) -> ()  [unwired: 1 out]
                n1387 = VISA Write(VISA resource name=w2849, write buffer="outp on" ("写入缓冲区"), error in (no error)=w2848) -> (VISA resource name out=w2851:refnum<visa-resource-name>, error out=w2846:errorcluster)  [unwired: 1 out]
                n1388 = local write "VISA资源名称输出"(w2851) -> ()
              }
              frame #7 {
                n1389 = local write "控制读取  2"(TRUE ("控制读取")) -> ()
              }
            }
            n1390 = local write "REAL1"(w2807) -> ()
            n1391 = local write "Set"(w2807) -> ()
          }
        }
      }
      event "输出自定义值2 2": Value Change {
        n1392 = event-data() -> ("NewVal"=w2856:bool)  [unwired: 6 out]
        n1393 = case shown="真" w2856 {
          tunnel: w2855 -> [_ w2880]
          tunnel: [w2857 w2878] -> w2854
          frame False {
            w2858 = u8 0 ("禁用")
            n1394 = local read "VISA资源名称输出"() -> (w2863:refnum<visa-resource-name>)
            n1395 = local write "控制读取  2"(FALSE ("控制读取")) -> ()
            n1396 = flat-sequence {
              tunnel: [w2866] -> w2864
              tunnel: w2863 -> [w2866]
              tunnel: w2864 -> [w2868]
              tunnel: [w2867] -> w2861
              tunnel: w2861 -> [w2871]
              tunnel: [w2871] -> w2860
              tunnel: [w2874] -> w2862
              tunnel: w2860 -> [w2875]
              tunnel: [w2872] -> w2857
              frame #0 {
                n1397 = Wait (ms)(milliseconds to wait=u32 200 ("等待时间（毫秒）")) -> ()  [unwired: 1 out]
              }
              frame #1 {
                n1398 = VISA Write(VISA resource name=w2868, write buffer="outp off" ("写入缓冲区")) -> (VISA resource name out=w2867:refnum<visa-resource-name>)  [unwired: 1 in, 2 out]
              }
              frame #2 {
                n1399 = Wait (ms)(milliseconds to wait=u32 50 ("等待时间（毫秒）")) -> ()  [unwired: 1 out]
              }
              frame #3 {
                n1400 = local write "控制读取  2"(TRUE ("控制读取")) -> ()
                n1401 = VISA Write(VISA resource name=w2875, write buffer="outp off" ("写入缓冲区")) -> (VISA resource name out=w2874:refnum<visa-resource-name>, error out=w2872:errorcluster)  [unwired: 1 in, 1 out]
              }
            }
            n1402 = local write "VISA资源名称输出"(w2862) -> ()
            n1403 = property on="输出100A" class="Bool"("Disabled"=w2858) -> ()  [unwired: 2 in, 2 out]
            n1404 = property on="输出200A" class="Bool"("Disabled"=w2858) -> ()  [unwired: 2 in, 2 out]
            n1405 = property on="输出自定义值2 2" class="Bool"("Disabled"=w2858) -> ()  [unwired: 2 in, 2 out]
            n1406 = property on="输出自定义值1 2" class="Bool"("Disabled"=w2858) -> ()  [unwired: 2 in, 2 out]
          }
          frame True {
            n1407 = local read "Curr2"() -> (w2877:dbl)
            n1408 = flat-sequence {
              tunnel: FALSE ("控制读取") -> [w2892]
              tunnel: [w2902] -> w2887
              tunnel: [w2901] -> w2885
              tunnel: [w2896] -> w2881
              tunnel: w2880 -> [w2894]
              tunnel: w2887 -> [w2906]
              tunnel: [w2906] -> w2886
              tunnel: w2885 -> [w2905]
              tunnel: [w2905] -> w2884
              tunnel: [w2903] -> w2882
              tunnel: w2881 -> [w2903]
              tunnel: w2886 -> [w2911]
              tunnel: w2884 -> [w2910]
              tunnel: [w2909] -> w2891
              tunnel: [w2908] -> w2889
              tunnel: w2882 -> [w2907]
              tunnel: w2891 -> [w2914]
              tunnel: [w2914] -> w2890
              tunnel: w2889 -> [w2913]
              tunnel: [w2913] -> w2888
              tunnel: w2890 -> [w2918]
              tunnel: w2888 -> [w2917]
              tunnel: [w2915] -> w2879
              tunnel: w2879 -> [w2921]
              tunnel: [w2921] -> w2878
              frame #0 {
                n1409 = local write "控制读取  2"(w2892) -> ()
              }
              frame #1 {
                n1410 = Wait (ms)(milliseconds to wait=u32 50 ("等待时间（毫秒）")) -> ()  [unwired: 1 out]
              }
              frame #2 {
                n1411 = local read "VISA资源名称输出"() -> (w2900:refnum<visa-resource-name>)
                n1412 = local read "Curr2"() -> (w2895:dbl)
                n1413 = Number To Fractional String(number=w2895, precision (6)=i16 3 ("精度(6)")) -> (F-format string=w2897:string)  [unwired: 2 out]
                n1414 = Concatenate Strings("volt 1;curr " ("写入缓冲区"), w2897) -> (w2896:string)
                n1415 = VISA Write(VISA resource name=w2900, write buffer=w2896, error in (no error)=w2894) -> (VISA resource name out=w2902:refnum<visa-resource-name>, error out=w2901:errorcluster)  [unwired: 1 out]
              }
              frame #3 {
                n1416 = Wait (ms)(milliseconds to wait=u32 50 ("等待时间（毫秒）")) -> ()  [unwired: 1 out]
              }
              frame #4 {
                n1417 = VISA Write(VISA resource name=w2911, write buffer=w2907, error in (no error)=w2910) -> (VISA resource name out=w2909:refnum<visa-resource-name>, error out=w2908:errorcluster)  [unwired: 1 out]
              }
              frame #5 {
                n1418 = Wait (ms)(milliseconds to wait=u32 200 ("等待时间（毫秒）")) -> ()  [unwired: 1 out]
              }
              frame #6 {
                n1419 = Wait (ms)(milliseconds to wait=u32 50 ("等待时间（毫秒）")) -> ()  [unwired: 1 out]
                n1420 = VISA Write(VISA resource name=w2918, write buffer="outp on" ("写入缓冲区"), error in (no error)=w2917) -> (VISA resource name out=w2920:refnum<visa-resource-name>, error out=w2915:errorcluster)  [unwired: 1 out]
                n1421 = local write "VISA资源名称输出"(w2920) -> ()
              }
              frame #7 {
                n1422 = local write "控制读取  2"(TRUE ("控制读取")) -> ()
              }
            }
            n1423 = local write "REAL2"(w2877) -> ()
            n1424 = local write "Set"(w2877) -> ()
          }
        }
      }
      event Timeout {
        n1425 = event-data() -> ()  [unwired: 4 out]
      }
      event "监控": Value Change {
        n1426 = event-data() -> ("NewVal"=w2924:bool)  [unwired: 6 out]
        n1427 = case shown="真" w2924 {
          tunnel: [FALSE ("监控 2") TRUE ("监控 2")] -> w2923
          frame False {
          }
          frame True {
          }
        }
        n1428 = local write "监控 2"(w2923) -> ()
      }
      event Menu Selection (User) {
        n1429 = event-data() -> ("ItemTag"=w2927:string)  [unwired: 7 out]
        n1430 = call "getpath.vi"() -> ("stripped path"=w2928:path)  [unwired: 11 out]
        n1431 = case shown="\"自定义\"" w2927 {
          tunnel: w2928 -> [_ w2931 w3014 w3097 w3180]
          frame "假", Default {
          }
          frame "300A以下" {
            n1432 = Build Path(base path=w2931, name or relative path="Settings\\300以下分辨率偏移值.xls" ("名称或相对路径")) -> (appended path=w2937:path)
            n1433 = local read "分辨率偏移值 3"() -> (w2932:T4)
            n1434 = call-poly <vilib>:"Read From Spreadsheet File.vi"("file path (dialog if empty)"=w2937) -> ("all rows"=w2934:string[][])  [unwired: 3 in, 7 out]
            n1435 = Delete From Array(array=w2934, length=1 ("长度"), index (row)=0 ("索引")) -> (array with subset deleted=w2933:string[][])  [unwired: 1 in, 1 out]
            n1436 = for {
              tunnel: w2933 -> [w2946] mode=indexing
              shift-right: [w2938] -> w2929
              shift-left: w2932 -> [w2943]
              n1437 = Index Array(array=w2946, index #1=0 ("索引")) -> (element #1=w2944:string, element #2=w2942:string, element #3=w2940:string)  [unwired: 2 in]
              n1438 = Fract/Exp String To Number(string=w2942) -> (number=w2941:dbl)  [unwired: 4 out]
              n1439 = Fract/Exp String To Number(string=w2940) -> (number=w2939:dbl)  [unwired: 4 out]
              n1440 = case shown="\"高压板功率\"" w2944 {
                tunnel: w2943 -> [w2947 w2951 w2955 w2959 w2963 w2967 w2971 w2975 w2979 w2983 w2987 w2991 w2995 w2999 w3003 w3007 w3011]
                tunnel: [w2947 w2950 w2954 w2958 w2962 w2966 w2970 w2974 w2978 w2982 w2986 w2990 w2994 w2998 w3002 w3006 w3010] -> w2938
                tunnel: w2941 -> [_ w2949 w2953 w2957 w2961 w2965 w2969 w2973 w2977 w2981 w2985 w2989 w2993 w2997 w3001 w3005 w3009]
                tunnel: w2939 -> [_ w2948 w2952 w2956 w2960 w2964 w2968 w2972 w2976 w2980 w2984 w2988 w2992 w2996 w3000 w3004 w3008]
                frame "假", Default {
                }
                frame "主板总电压" {
                  n1441 = Bundle By Name(cluster=w2951, "主板总电压分辨率"=w2949, "主板总电压偏移量"=w2948) -> (w2950:T4)
                }
                frame "高压板总电压" {
                  n1442 = Bundle By Name(cluster=w2955, "高压板总电压分辨率"=w2953, "高压板总电压偏移量"=w2952) -> (w2954:T4)
                }
                frame "高压板总电流" {
                  n1443 = Bundle By Name(cluster=w2959, "高压板总电流分辨率"=w2957, "高压板总电流偏移量"=w2956) -> (w2958:T4)
                }
                frame "高压板安时" {
                  n1444 = Bundle By Name(cluster=w2963, "高压板安时分辨率"=w2961, "高压板安时偏移量"=w2960) -> (w2962:T4)
                }
                frame "高压板SOC" {
                  n1445 = Bundle By Name(cluster=w2967, "高压板SOC分辨率"=w2965, "高压板SOC偏移量"=w2964) -> (w2966:T4)
                }
                frame "高压板功率" {
                  n1446 = Bundle By Name(cluster=w2971, "高压板功率分辨率"=w2969, "高压板功率偏移量"=w2968) -> (w2970:T4)
                }
                frame "主板总电流" {
                  n1447 = Bundle By Name(cluster=w2975, "主板总电流分辨率"=w2973, "主板总电流偏移量"=w2972) -> (w2974:T4)
                }
                frame "主板安时" {
                  n1448 = Bundle By Name(cluster=w2979, "主板安时分辨率"=w2977, "主板安时偏移量"=w2976) -> (w2978:T4)
                }
                frame "主板SOC" {
                  n1449 = Bundle By Name(cluster=w2983, "主板SOC分辨率"=w2981, "主板SOC偏移量"=w2980) -> (w2982:T4)
                }
                frame "从板总电压" {
                  n1450 = Bundle By Name(cluster=w2987, "从板总电压分辨率"=w2985, "从板总电压偏移量"=w2984) -> (w2986:T4)
                }
                frame "从板总电流" {
                  n1451 = Bundle By Name(cluster=w2991, "从板总电流分辨率"=w2989, "从板总电流偏移量"=w2988) -> (w2990:T4)
                }
                frame "从板安时" {
                  n1452 = Bundle By Name(cluster=w2995, "从板安时分辨率"=w2993, "从板安时偏移量"=w2992) -> (w2994:T4)
                }
                frame "从板SOC" {
                  n1453 = Bundle By Name(cluster=w2999, "从板SOC分辨率"=w2997, "从板SOC偏移量"=w2996) -> (w2998:T4)
                }
                frame "温度" {
                  n1454 = Bundle By Name(cluster=w3003, "温度分辨率"=w3001, "温度偏移量"=w3000) -> (w3002:T4)
                }
                frame "功率" {
                  n1455 = Bundle By Name(cluster=w3007, "功率分辨率"=w3005, "功率偏移量"=w3004) -> (w3006:T4)
                }
                frame "单体电压" {
                  n1456 = Bundle By Name(cluster=w3011, "单体电压分辨率"=w3009, "单体电压偏移量"=w3008) -> (w3010:T4)
                }
              }
            }
            n1457 = local write "分辨率偏移值 3"(w2929) -> ()
          }
          frame "400A以上" {
            n1458 = Build Path(base path=w3014, name or relative path="Settings\\400以上分辨率偏移值.xls" ("名称或相对路径")) -> (appended path=w3020:path)
            n1459 = local read "分辨率偏移值 3"() -> (w3015:T4)
            n1460 = call-poly <vilib>:"Read From Spreadsheet File.vi"("file path (dialog if empty)"=w3020) -> ("all rows"=w3017:string[][])  [unwired: 3 in, 7 out]
            n1461 = Delete From Array(array=w3017, length=1 ("长度"), index (row)=0 ("索引")) -> (array with subset deleted=w3016:string[][])  [unwired: 1 in, 1 out]
            n1462 = for {
              tunnel: w3016 -> [w3029] mode=indexing
              shift-right: [w3021] -> w3012
              shift-left: w3015 -> [w3026]
              n1463 = Index Array(array=w3029, index #1=0 ("索引")) -> (element #1=w3027:string, element #2=w3025:string, element #3=w3023:string)  [unwired: 2 in]
              n1464 = Fract/Exp String To Number(string=w3025) -> (number=w3024:dbl)  [unwired: 4 out]
              n1465 = Fract/Exp String To Number(string=w3023) -> (number=w3022:dbl)  [unwired: 4 out]
              n1466 = case shown="\"高压板功率\"" w3027 {
                tunnel: w3026 -> [w3030 w3034 w3038 w3042 w3046 w3050 w3054 w3058 w3062 w3066 w3070 w3074 w3078 w3082 w3086 w3090 w3094]
                tunnel: [w3030 w3033 w3037 w3041 w3045 w3049 w3053 w3057 w3061 w3065 w3069 w3073 w3077 w3081 w3085 w3089 w3093] -> w3021
                tunnel: w3024 -> [_ w3032 w3036 w3040 w3044 w3048 w3052 w3056 w3060 w3064 w3068 w3072 w3076 w3080 w3084 w3088 w3092]
                tunnel: w3022 -> [_ w3031 w3035 w3039 w3043 w3047 w3051 w3055 w3059 w3063 w3067 w3071 w3075 w3079 w3083 w3087 w3091]
                frame "假", Default {
                }
                frame "主板总电压" {
                  n1467 = Bundle By Name(cluster=w3034, "主板总电压分辨率"=w3032, "主板总电压偏移量"=w3031) -> (w3033:T4)
                }
                frame "高压板总电压" {
                  n1468 = Bundle By Name(cluster=w3038, "高压板总电压分辨率"=w3036, "高压板总电压偏移量"=w3035) -> (w3037:T4)
                }
                frame "高压板总电流" {
                  n1469 = Bundle By Name(cluster=w3042, "高压板总电流分辨率"=w3040, "高压板总电流偏移量"=w3039) -> (w3041:T4)
                }
                frame "高压板安时" {
                  n1470 = Bundle By Name(cluster=w3046, "高压板安时分辨率"=w3044, "高压板安时偏移量"=w3043) -> (w3045:T4)
                }
                frame "高压板SOC" {
                  n1471 = Bundle By Name(cluster=w3050, "高压板SOC分辨率"=w3048, "高压板SOC偏移量"=w3047) -> (w3049:T4)
                }
                frame "高压板功率" {
                  n1472 = Bundle By Name(cluster=w3054, "高压板功率分辨率"=w3052, "高压板功率偏移量"=w3051) -> (w3053:T4)
                }
                frame "主板总电流" {
                  n1473 = Bundle By Name(cluster=w3058, "主板总电流分辨率"=w3056, "主板总电流偏移量"=w3055) -> (w3057:T4)
                }
                frame "主板安时" {
                  n1474 = Bundle By Name(cluster=w3062, "主板安时分辨率"=w3060, "主板安时偏移量"=w3059) -> (w3061:T4)
                }
                frame "主板SOC" {
                  n1475 = Bundle By Name(cluster=w3066, "主板SOC分辨率"=w3064, "主板SOC偏移量"=w3063) -> (w3065:T4)
                }
                frame "从板总电压" {
                  n1476 = Bundle By Name(cluster=w3070, "从板总电压分辨率"=w3068, "从板总电压偏移量"=w3067) -> (w3069:T4)
                }
                frame "从板总电流" {
                  n1477 = Bundle By Name(cluster=w3074, "从板总电流分辨率"=w3072, "从板总电流偏移量"=w3071) -> (w3073:T4)
                }
                frame "从板安时" {
                  n1478 = Bundle By Name(cluster=w3078, "从板安时分辨率"=w3076, "从板安时偏移量"=w3075) -> (w3077:T4)
                }
                frame "从板SOC" {
                  n1479 = Bundle By Name(cluster=w3082, "从板SOC分辨率"=w3080, "从板SOC偏移量"=w3079) -> (w3081:T4)
                }
                frame "温度" {
                  n1480 = Bundle By Name(cluster=w3086, "温度分辨率"=w3084, "温度偏移量"=w3083) -> (w3085:T4)
                }
                frame "功率" {
                  n1481 = Bundle By Name(cluster=w3090, "功率分辨率"=w3088, "功率偏移量"=w3087) -> (w3089:T4)
                }
                frame "单体电压" {
                  n1482 = Bundle By Name(cluster=w3094, "单体电压分辨率"=w3092, "单体电压偏移量"=w3091) -> (w3093:T4)
                }
              }
            }
            n1483 = local write "分辨率偏移值 3"(w3012) -> ()
          }
          frame "自定义" {
            n1484 = Build Path(base path=w3097, name or relative path="Settings\\分辨率偏移值.xls" ("名称或相对路径")) -> (appended path=w3103:path)
            n1485 = local read "分辨率偏移值 3"() -> (w3098:T4)
            n1486 = call-poly <vilib>:"Read From Spreadsheet File.vi"("file path (dialog if empty)"=w3103) -> ("all rows"=w3100:string[][])  [unwired: 3 in, 7 out]
            n1487 = Delete From Array(array=w3100, length=1 ("长度"), index (row)=0 ("索引")) -> (array with subset deleted=w3099:string[][])  [unwired: 1 in, 1 out]
            n1488 = for {
              tunnel: w3099 -> [w3112] mode=indexing
              shift-right: [w3104] -> w3095
              shift-left: w3098 -> [w3109]
              n1489 = Index Array(array=w3112, index #1=0 ("索引")) -> (element #1=w3110:string, element #2=w3108:string, element #3=w3106:string)  [unwired: 2 in]
              n1490 = Fract/Exp String To Number(string=w3108) -> (number=w3107:dbl)  [unwired: 4 out]
              n1491 = Fract/Exp String To Number(string=w3106) -> (number=w3105:dbl)  [unwired: 4 out]
              n1492 = case shown="\"高压板功率\"" w3110 {
                tunnel: w3109 -> [w3113 w3117 w3121 w3125 w3129 w3133 w3137 w3141 w3145 w3149 w3153 w3157 w3161 w3165 w3169 w3173 w3177]
                tunnel: [w3113 w3116 w3120 w3124 w3128 w3132 w3136 w3140 w3144 w3148 w3152 w3156 w3160 w3164 w3168 w3172 w3176] -> w3104
                tunnel: w3107 -> [_ w3115 w3119 w3123 w3127 w3131 w3135 w3139 w3143 w3147 w3151 w3155 w3159 w3163 w3167 w3171 w3175]
                tunnel: w3105 -> [_ w3114 w3118 w3122 w3126 w3130 w3134 w3138 w3142 w3146 w3150 w3154 w3158 w3162 w3166 w3170 w3174]
                frame "假", Default {
                }
                frame "主板总电压" {
                  n1493 = Bundle By Name(cluster=w3117, "主板总电压分辨率"=w3115, "主板总电压偏移量"=w3114) -> (w3116:T4)
                }
                frame "高压板总电压" {
                  n1494 = Bundle By Name(cluster=w3121, "高压板总电压分辨率"=w3119, "高压板总电压偏移量"=w3118) -> (w3120:T4)
                }
                frame "高压板总电流" {
                  n1495 = Bundle By Name(cluster=w3125, "高压板总电流分辨率"=w3123, "高压板总电流偏移量"=w3122) -> (w3124:T4)
                }
                frame "高压板安时" {
                  n1496 = Bundle By Name(cluster=w3129, "高压板安时分辨率"=w3127, "高压板安时偏移量"=w3126) -> (w3128:T4)
                }
                frame "高压板SOC" {
                  n1497 = Bundle By Name(cluster=w3133, "高压板SOC分辨率"=w3131, "高压板SOC偏移量"=w3130) -> (w3132:T4)
                }
                frame "高压板功率" {
                  n1498 = Bundle By Name(cluster=w3137, "高压板功率分辨率"=w3135, "高压板功率偏移量"=w3134) -> (w3136:T4)
                }
                frame "主板总电流" {
                  n1499 = Bundle By Name(cluster=w3141, "主板总电流分辨率"=w3139, "主板总电流偏移量"=w3138) -> (w3140:T4)
                }
                frame "主板安时" {
                  n1500 = Bundle By Name(cluster=w3145, "主板安时分辨率"=w3143, "主板安时偏移量"=w3142) -> (w3144:T4)
                }
                frame "主板SOC" {
                  n1501 = Bundle By Name(cluster=w3149, "主板SOC分辨率"=w3147, "主板SOC偏移量"=w3146) -> (w3148:T4)
                }
                frame "从板总电压" {
                  n1502 = Bundle By Name(cluster=w3153, "从板总电压分辨率"=w3151, "从板总电压偏移量"=w3150) -> (w3152:T4)
                }
                frame "从板总电流" {
                  n1503 = Bundle By Name(cluster=w3157, "从板总电流分辨率"=w3155, "从板总电流偏移量"=w3154) -> (w3156:T4)
                }
                frame "从板安时" {
                  n1504 = Bundle By Name(cluster=w3161, "从板安时分辨率"=w3159, "从板安时偏移量"=w3158) -> (w3160:T4)
                }
                frame "从板SOC" {
                  n1505 = Bundle By Name(cluster=w3165, "从板SOC分辨率"=w3163, "从板SOC偏移量"=w3162) -> (w3164:T4)
                }
                frame "温度" {
                  n1506 = Bundle By Name(cluster=w3169, "温度分辨率"=w3167, "温度偏移量"=w3166) -> (w3168:T4)
                }
                frame "功率" {
                  n1507 = Bundle By Name(cluster=w3173, "功率分辨率"=w3171, "功率偏移量"=w3170) -> (w3172:T4)
                }
                frame "单体电压" {
                  n1508 = Bundle By Name(cluster=w3177, "单体电压分辨率"=w3175, "单体电压偏移量"=w3174) -> (w3176:T4)
                }
              }
            }
            n1509 = local write "分辨率偏移值 3"(w3095) -> ()
          }
          frame "自定义分辨率" {
            n1510 = Build Path(base path=w3180, name or relative path="SubVi\\分辨率自定义.vi" ("名称或相对路径")) -> (appended path=w3178:path)
            n1511 = Open VI Reference(vi path=w3178) -> (vi reference=w3187:refnum<vi>)  [unwired: 1 in, 5 out]
            n1512 = invoke class="VI" method="FP.Open"(reference=w3187, "Activate"=TRUE ("激活？"), "State"=T12."Standard" ("状态")) -> (reference out=w3184:refnum<vi>, error out=w3183:errorcluster)  [unwired: 2 in, 3 out]
            n1513 = invoke class="VI" method="Run VI"(reference=w3184, error in=w3183, "Wait until done"=FALSE ("结束前等待"), "Auto Dispose Ref"=TRUE ("自动销毁引用")) -> ()  [unwired: 1 in, 5 out]
          }
        }
      }
      event "Read1": Value Change {
        n1514 = event-data() -> ("NewVal"=w3192:bool)  [unwired: 6 out]
        n1515 = case shown="真" w3192 {
          tunnel: w3191 -> [w3194 w3211]
          tunnel: w3190 -> [w3193 w3210]
          tunnel: [w3193 w3209] -> w3189
          tunnel: [w3194 w3208] -> w3188
          frame False {
          }
          frame True {
            n1516 = flat-sequence {
              tunnel: w3210 -> [w3212]
              tunnel: w3211 -> [w3213]
              tunnel: [w3213] -> w3201
              tunnel: [w3212] -> w3199
              tunnel: w3201 -> [w3215]
              tunnel: [w3215] -> w3200
              tunnel: w3199 -> [w3214]
              tunnel: [w3214] -> w3198
              tunnel: w3200 -> [w3217]
              tunnel: [w3217] -> w3205
              tunnel: w3198 -> [w3216]
              tunnel: [w3216] -> w3203
              tunnel: w3205 -> [w3219]
              tunnel: [w3219] -> w3204
              tunnel: w3203 -> [w3218]
              tunnel: [w3218] -> w3202
              tunnel: [w3224] -> w3209
              tunnel: [w3223] -> w3208
              tunnel: w3204 -> [w3226]
              tunnel: w3202 -> [w3225]
              frame #0 {
              }
              frame #1 {
              }
              frame #2 {
              }
              frame #3 {
                n1517 = disable-structure shown="禁用" {
                  frame Disabled {
                    n1518 = local read "自动控制仪器"() -> (w3220:bool)
                    n1519 = case shown="真" w3220 {
                      frame False {
                      }
                      frame True {
                        n1520 = Wait (ms)(milliseconds to wait=u32 2000 ("等待时间（毫秒）")) -> ()  [unwired: 1 out]
                      }
                    }
                  }
                  frame Enabled {
                  }
                }
              }
              frame #4 {
                n1521 = Enqueue Element(queue=w3226, element="Read1" ("元素"), error in (no error)=w3225) -> (queue out=w3223:refnum<queue>, error out=w3224:errorcluster)  [unwired: 2 out]
              }
            }
            n1522 = global write "EV05全局变量1.vi" "CAN接收"(FALSE ("CAN接收")) -> ()
            n1523 = global write "EV05全局变量1.vi" "高压校正接收"(FALSE ("高压校正接收")) -> ()
            n1524 = call <vilib>:"Set Busy.vi"() -> ()  [unwired: 4 in, 8 out]
            n1525 = local write "AD1"(u16 0 ("AD1")) -> ()
            n1526 = property on="Read1结果" class="Bool (严格)"("Colors [4]"=cluster{u32, u32}[] [{0, 0}] ("颜色[4]"), "BoolText.Text"="" ("布尔文本.文本")) -> ()  [unwired: 2 in, 2 out]
          }
        }
      }
      event "Read1_Out": Value Change {
        n1527 = event-data() -> ("NewVal"=w3231:bool)  [unwired: 6 out]
        n1528 = case shown="真" w3231 {
          tunnel: w3230 -> [w3233 w3250]
          tunnel: w3229 -> [w3232 w3249]
          tunnel: [w3232 w3248] -> w3228
          tunnel: [w3233 w3247] -> w3227
          frame False {
          }
          frame True {
            n1529 = flat-sequence {
              tunnel: w3249 -> [w3251]
              tunnel: w3250 -> [w3252]
              tunnel: [w3252] -> w3240
              tunnel: [w3251] -> w3238
              tunnel: w3240 -> [w3254]
              tunnel: [w3254] -> w3239
              tunnel: w3238 -> [w3253]
              tunnel: [w3253] -> w3237
              tunnel: w3239 -> [w3256]
              tunnel: [w3256] -> w3244
              tunnel: w3237 -> [w3255]
              tunnel: [w3255] -> w3242
              tunnel: w3244 -> [w3258]
              tunnel: [w3258] -> w3243
              tunnel: w3242 -> [w3257]
              tunnel: [w3257] -> w3241
              tunnel: [w3261] -> w3248
              tunnel: [w3260] -> w3247
              tunnel: w3243 -> [w3263]
              tunnel: w3241 -> [w3262]
              frame #0 {
              }
              frame #1 {
              }
              frame #2 {
              }
              frame #3 {
              }
              frame #4 {
                n1530 = Enqueue Element(queue=w3263, element="Read1_out" ("元素"), error in (no error)=w3262) -> (queue out=w3260:refnum<queue>, error out=w3261:errorcluster)  [unwired: 2 out]
              }
            }
            n1531 = global write "EV05全局变量1.vi" "CAN接收"(FALSE ("CAN接收")) -> ()
            n1532 = global write "EV05全局变量1.vi" "高压校正接收"(FALSE ("高压校正接收")) -> ()
            n1533 = call <vilib>:"Set Busy.vi"() -> ()  [unwired: 4 in, 8 out]
            n1534 = property on="Read1_Out结果" class="Bool (严格)"("Colors [4]"=cluster{u32, u32}[] [{0, 0}] ("颜色[4]"), "BoolText.Text"="" ("布尔文本.文本")) -> ()  [unwired: 2 in, 2 out]
            n1535 = local write "AD1"(0.0 ("AD1 3")) -> ()
          }
        }
      }
      event "Read2_Out": Value Change {
        n1536 = event-data() -> ("NewVal"=w3268:bool)  [unwired: 6 out]
        n1537 = case shown="真" w3268 {
          tunnel: w3267 -> [w3270 w3286]
          tunnel: w3266 -> [w3269 w3285]
          tunnel: [w3269 w3284] -> w3265
          tunnel: [w3270 w3283] -> w3264
          frame False {
          }
          frame True {
            n1538 = flat-sequence {
              tunnel: w3285 -> [w3287]
              tunnel: w3286 -> [w3288]
              tunnel: [w3288] -> w3276
              tunnel: [w3287] -> w3274
              tunnel: w3276 -> [w3290]
              tunnel: [w3290] -> w3275
              tunnel: w3274 -> [w3289]
              tunnel: [w3289] -> w3273
              tunnel: w3275 -> [w3292]
              tunnel: [w3292] -> w3280
              tunnel: w3273 -> [w3291]
              tunnel: [w3291] -> w3278
              tunnel: w3280 -> [w3294]
              tunnel: [w3294] -> w3279
              tunnel: w3278 -> [w3293]
              tunnel: [w3293] -> w3277
              tunnel: [w3297] -> w3284
              tunnel: [w3296] -> w3283
              tunnel: w3279 -> [w3299]
              tunnel: w3277 -> [w3298]
              frame #0 {
              }
              frame #1 {
              }
              frame #2 {
              }
              frame #3 {
              }
              frame #4 {
                n1539 = Enqueue Element(queue=w3299, element="Read2_out" ("元素"), error in (no error)=w3298) -> (queue out=w3296:refnum<queue>, error out=w3297:errorcluster)  [unwired: 2 out]
              }
            }
            n1540 = global write "EV05全局变量1.vi" "高压校正接收"(FALSE ("高压校正接收")) -> ()
            n1541 = global write "EV05全局变量1.vi" "CAN接收"(FALSE ("CAN接收")) -> ()
            n1542 = call <vilib>:"Set Busy.vi"() -> ()  [unwired: 4 in, 8 out]
            n1543 = property on="Read2_Out结果" class="Bool (严格)"("Colors [4]"=cluster{u32, u32}[] [{0, 0}] ("颜色[4]"), "BoolText.Text"="" ("布尔文本.文本")) -> ()  [unwired: 2 in, 2 out]
          }
        }
      }
      event "Clear": Value Change {
        n1544 = event-data() -> ("NewVal"=w3304:bool)  [unwired: 6 out]
        n1545 = case shown="真" w3304 {
          tunnel: w3303 -> [w3306 w3314]
          tunnel: w3302 -> [w3305 w3313]
          tunnel: [w3305 w3312] -> w3301
          tunnel: [w3306 w3311] -> w3300
          frame False {
          }
          frame True {
            n1546 = flat-sequence {
              tunnel: w3313 -> [w3315]
              tunnel: w3314 -> [w3316]
              tunnel: [w3316] -> w3310
              tunnel: [w3315] -> w3309
              tunnel: [w3319] -> w3312
              tunnel: [w3318] -> w3311
              tunnel: w3310 -> [w3321]
              tunnel: w3309 -> [w3320]
              frame #0 {
              }
              frame #1 {
                n1547 = Enqueue Element(queue=w3321, element="Clear" ("元素"), error in (no error)=w3320) -> (queue out=w3318:refnum<queue>, error out=w3319:errorcluster)  [unwired: 2 out]
              }
            }
            n1548 = property on="Clear结果" class="Bool (严格)"("Colors [4]"=cluster{u32, u32}[] [{0, 0}] ("颜色[4]"), "BoolText.Text"="" ("布尔文本.文本")) -> ()  [unwired: 2 in, 2 out]
          }
        }
      }
      event "写配置文件版本": Value Change {
        n1549 = event-data() -> ("NewVal"=w3326:bool)  [unwired: 6 out]
        n1550 = case shown="真" w3326 {
          tunnel: w3325 -> [w3328 w3336]
          tunnel: w3324 -> [w3327 w3335]
          tunnel: [w3327 w3334] -> w3323
          tunnel: [w3328 w3333] -> w3322
          frame False {
          }
          frame True {
            n1551 = flat-sequence {
              tunnel: w3335 -> [w3337]
              tunnel: w3336 -> [w3338]
              tunnel: [w3338] -> w3332
              tunnel: [w3337] -> w3331
              tunnel: [w3341] -> w3334
              tunnel: [w3340] -> w3333
              tunnel: w3332 -> [w3343]
              tunnel: w3331 -> [w3342]
              frame #0 {
              }
              frame #1 {
                n1552 = Enqueue Element(queue=w3343, element="写配置文件版本" ("元素"), error in (no error)=w3342) -> (queue out=w3340:refnum<queue>, error out=w3341:errorcluster)  [unwired: 2 out]
              }
            }
            n1553 = property on="写版本结果" class="Bool (严格)"("Colors [4]"=cluster{u32, u32}[] [{0, 0}] ("颜色[4]"), "BoolText.Text"="" ("布尔文本.文本")) -> ()  [unwired: 2 in, 2 out]
          }
        }
      }
      event "读配置文件版本": Value Change {
        n1554 = event-data() -> ("NewVal"=w3348:bool)  [unwired: 6 out]
        n1555 = case shown="真" w3348 {
          tunnel: w3347 -> [w3350 w3359]
          tunnel: w3346 -> [w3349 w3358]
          tunnel: [w3349 w3357] -> w3345
          tunnel: [w3350 w3356] -> w3344
          frame False {
          }
          frame True {
            n1556 = flat-sequence {
              tunnel: w3358 -> [w3360]
              tunnel: w3359 -> [w3361]
              tunnel: [w3361] -> w3355
              tunnel: [w3360] -> w3354
              tunnel: [w3364] -> w3357
              tunnel: [w3363] -> w3356
              tunnel: w3355 -> [w3366]
              tunnel: w3354 -> [w3365]
              frame #0 {
              }
              frame #1 {
                n1557 = Enqueue Element(queue=w3366, element="读配置文件版本" ("元素"), error in (no error)=w3365) -> (queue out=w3363:refnum<queue>, error out=w3364:errorcluster)  [unwired: 2 out]
              }
            }
            n1558 = local write "版本号-读"("\u0000\u0000\u0000\u0000\u0000\u0000\u0000\u0000" ("版本号-读")) -> ()
            n1559 = property on="读版本结果" class="Bool (严格)"("Colors [4]"=cluster{u32, u32}[] [{0, 0}] ("颜色[4]"), "BoolText.Text"="" ("布尔文本.文本")) -> ()  [unwired: 2 in, 2 out]
          }
        }
      }
      event "设置参数": Value Change {
        n1560 = event-data() -> ("NewVal"=w3371:bool)  [unwired: 6 out]
        n1561 = case shown="真" w3371 {
          tunnel: w3370 -> [w3373 w3453]
          tunnel: w3369 -> [w3372 w3452]
          tunnel: [w3372 w3451] -> w3368
          tunnel: [w3373 w3450] -> w3367
          frame False {
          }
          frame True {
            w3445 = u16 1 ("y")
            n1562 = flat-sequence {
              tunnel: w3452 -> [w3454]
              tunnel: w3453 -> [w3455]
              tunnel: [w3455] -> w3449
              tunnel: [w3454] -> w3448
              tunnel: [w3458] -> w3451
              tunnel: [w3457] -> w3450
              tunnel: w3449 -> [w3460]
              tunnel: w3448 -> [w3459]
              frame #0 {
              }
              frame #1 {
                n1563 = Enqueue Element(queue=w3460, element="设置参数" ("元素"), error in (no error)=w3459) -> (queue out=w3457:refnum<queue>, error out=w3458:errorcluster)  [unwired: 2 out]
              }
            }
            n1564 = Add(x="传感器类型", y=u16 1) -> (x+y=w3431:u16)
            n1565 = Add(x="分流器大小/A", y=u16 1) -> (x+y=w3432:u16)
            n1566 = Add(x=w3445, y="电压分辨率/V") -> (x+y=w3442:u16)
            n1567 = Add(x=w3445, y="安时分辨率/AH") -> (x+y=w3441:u16)
            n1568 = Add(x="电流分辨率/A", y=w3445) -> (x+y=w3381:u16)
            n1569 = Multiply(x=u16 16, y=w3432) -> (x*y=w3430:u16)
            n1570 = Add(x=w3431, y=w3430) -> (x+y=w3428:u16)
            n1571 = Multiply(x=u16 16, y=w3441) -> (x*y=w3439:u16)
            n1572 = Multiply(x=u16 4, y=w3442) -> (x*y=w3440:u16)
            n1573 = Number To Hexadecimal String(1:i16 2 ("宽度(-)"), 2:w3428) -> (0:w3401:string)
            n1574 = property on="连接状态 10" class="Bool (严格)"("Colors [4]"=cluster{u32, u32}[] [{0, 0}] ("颜色[4]"), "BoolText.Text"="" ("布尔文本.文本")) -> ()  [unwired: 2 in, 2 out]
            n1575 = Compound Arithmetic op=ADD(w3381, w3440, w3439) -> (w3437:u16)
            n1576 = Number To Hexadecimal String(1:i16 2 ("宽度(-)"), 2:w3437) -> (0:w3402:string)
            n1577 = Equal?(x="分流器大小/A", y=u16 0) -> (x = y?=w3419:bool)
            n1578 = Multiply(x=u16 100, y="分流器大小/A") -> (x*y=w3415:u16)
            n1579 = Equal?(x="安时分辨率/AH", y=u16 0) -> (x = y?=w3386:bool)
            n1580 = Equal?(x="是否有外部高压", y=u16 0) -> (x = y?=w3425:bool)
            n1581 = Select(t=u16 50 ("y"), s=w3419, f=w3415) -> (s? t:f=w3409:u16)
            n1582 = Select(t=u16 5 ("y"), s=w3425, f=u16 0 ("y")) -> (s? t:f=w3423:u16)
            n1583 = Select(t=u16 375 ("y"), s=w3386, f=u32 75006 ("y")) -> (s? t:f=w3408:u32)
            n1584 = Number To Hexadecimal String(1:i16 2 ("宽度(-)"), 2:w3423) -> (0:w3400:string)
            n1585 = Multiply(x=u16 300 ("y"), y=w3408) -> (x*y=w3406:u32)
            n1586 = Divide(x=w3406, y=w3409) -> (x/y=w3405:dbl)
            n1587 = Round To Nearest(number=w3405) -> (nearest integer value=w3404:dbl)
            "充放电阈值" <- w3404
            n1588 = Number To Hexadecimal String(1:i16 8 ("宽度(-)"), 2:w3404) -> (0:w3403:string)
            n1589 = Number To Hexadecimal String(1:i16 2 ("宽度(-)"), 2:0 ("数字")) -> (0:w3396:string)
            n1590 = Concatenate Strings(w3403, w3396, w3402, w3401, w3400) -> (→"config_data":string)
            n1591 = Equal?(x="电流分辨率/A", y=u16 0) -> (x = y?=w3376:bool)
            n1592 = Equal?(x="电压分辨率/V", y=u16 0) -> (x = y?=w3393:bool)
            n1593 = Select(t=sgl 0.01 ("y"), s=w3393, f=sgl 0.1 ("y")) -> (s? t:f=w3390:sgl)
            n1594 = Select(t=sgl 0.01 ("y"), s=w3376, f=sgl 0.1 ("y")) -> (s? t:f=w3380:sgl)
            n1595 = Select(t=sgl -300.0 ("y"), s=w3376, f=sgl -3000.0 ("y")) -> (s? t:f=w3375:sgl)
            n1596 = Select(t=sgl 0.001 ("y"), s=w3386, f=sgl 0.2 ("y")) -> (s? t:f=w3385:sgl)
            n1597 = local read "分辨率偏移值 3"() -> (w3395:T4)
            n1598 = Bundle By Name(cluster=w3395, "高压板总电压分辨率"=w3390, "高压板总电流分辨率"=w3380, "高压板总电流偏移量"=w3375, "高压板安时分辨率"=w3385) -> (w3379:T4)
            n1599 = local write "分辨率偏移值 3"(w3379) -> ()
          }
        }
      }
      event "生成配置": Value Change {
        n1600 = event-data() -> ("NewVal"=w3462:bool)  [unwired: 6 out]
        n1601 = case shown="真" w3462 {
          tunnel: w3461 -> [_ w3464]
          frame False {
          }
          frame True {
            n1602 = call "文件对话框"("error in"=w3464, "pattern (all files)"=".txt") -> ("selected path"=w3465:path, "cancelled"=w3466:bool, "error out"=w3463:errorcluster)  [unwired: 5 in, 6 out]
            n1603 = case shown="假" w3466 {
              tunnel: w3465 -> [w3471 _]
              tunnel: w3463 -> [_ _]
              frame False {
                n1604 = local read "安时分辨率/AH"() -> (w3506:u16)
                n1605 = local read "是否有外部高压"() -> (w3488:u16)
                n1606 = local read "电流分辨率/A"() -> (w3519:u16)
                n1607 = local read "电压分辨率/V"() -> (w3511:u16)
                n1608 = local read "传感器类型"() -> (w3501:u16)
                n1609 = local read "分流器大小/A"() -> (w3499:u16)
                n1610 = Equal To 0?(x=w3519) -> (x = 0?=w3518:bool)
                n1611 = Equal To 0?(x=w3511) -> (x = 0?=w3512:bool)
                n1612 = Equal To 0?(x=w3506) -> (x = 0?=w3509:bool)
                n1613 = local read "充放电阈值"() -> (w3486:dbl)
                n1614 = Equal To 0?(x=w3501) -> (x = 0?=w3502:bool)
                n1615 = Equal?(x=w3499, y=u16 0) -> (x = y?=w3497:bool)
                n1616 = Select(t="0.01", s=w3518, f="0.1") -> (s? t:f=w3515:string)
                n1617 = Select(t="0.01", s=w3512, f="0.1") -> (s? t:f=w3510:string)
                n1618 = Multiply(x=u16 100, y=w3499) -> (x*y=w3494:u16)
                n1619 = Select(t="0.001", s=w3509, f="0.2") -> (s? t:f=w3505:string)
                n1620 = Select(t="霍尔传感器", s=w3502, f="分流器") -> (s? t:f=w3500:string)
                n1621 = Equal To 0?(x=w3488) -> (x = 0?=w3491:bool)
                n1622 = Select(t=u16 50 ("y"), s=w3497, f=w3494) -> (s? t:f=w3493:u16)
                n1623 = Select(t="有", s=w3491, f="无") -> (s? t:f=w3487:string)
                n1624 = Number To Decimal String(number=w3493) -> (decimal integer string=w3492:string)  [unwired: 1 out]
                n1625 = Number To Decimal String(number=w3486) -> (decimal integer string=w3485:string)  [unwired: 1 out]
                n1626 = local read "版本号"() -> (w3480:string)
                n1627 = Build Array("参数值" ("元素"), w3515, w3510, w3505, w3500, w3492, w3487, w3485, w3480) -> (w3483:string[])
                n1628 = Build Array(string[] ["参数名称", "电流分辨率", "电压分辨率", "安时分辨率", "传感器类型", "分流器大小", "是否有外部高压", "充放电阈值", "配置文件版本号"], w3483) -> (w3481:string[][])
                n1629 = Transpose 2D Array(2D array=w3481) -> (transposed array=w3472:string[][])
                n1630 = call-poly <vilib>:"Write To Spreadsheet File.vi"("2D data"=w3472, "file path (dialog if empty)"=w3471) -> ("new file path (Not A Path if cancelled)"=w3468:path)  [unwired: 4 in, 2 out]
                n1631 = call <vilib>:"MD5Checksum File.vi"("Path"=w3468) -> ("MD5 message-digest"=w3478:string)  [unwired: 1 in, 9 out]
                n1632 = Strip Path(path=w3468) -> (stripped path=w3469:path)  [unwired: 1 out]
                n1633 = call <vilib>:"Get File Extension.vi"("file"=w3468) -> ("filename without extension"=w3476:string)  [unwired: 1 in, 9 out]
                n1634 = Concatenate Strings(w3476, "_(MD5=" ("字符串"), w3478, ")" ("字符串"), ".txt" ("字符串")) -> (w3474:string)
                n1635 = Build Path(base path=w3469, name or relative path=w3474) -> (appended path=w3473:path)
                n1636 = call-poly <vilib>:"Write To Spreadsheet File.vi"("2D data"=w3472, "file path (dialog if empty)"=w3473) -> ("new file path (Not A Path if cancelled)"=w3470:path)  [unwired: 4 in, 2 out]
                n1637 = flat-sequence {
                  tunnel: w3470 -> [_]
                  tunnel: w3468 -> [w3520]
                  frame #0 {
                    n1638 = Delete(path (use dialog)=w3520) -> ()  [unwired: 1 in, 6 out]
                  }
                }
              }
              frame True {
              }
            }
          }
        }
      }
      event "导入配置": Value Change {
        n1639 = event-data() -> ("NewVal"=w3522:bool)  [unwired: 6 out]
        n1640 = case shown="真" w3522 {
          tunnel: w3521 -> [_ w3524]
          frame False {
          }
          frame True {
            n1641 = property on="导入配置结果" class="Bool (严格)"("Colors [4]"=cluster{u32, u32}[] [{0, 0}] ("颜色[4]"), "BoolText.Text"="" ("布尔文本.文本")) -> ()  [unwired: 2 in, 2 out]
            n1642 = call "文件对话框2"("default name"=".txt", "error in"=w3524) -> ("selected path"=w3527:path, "cancelled"=w3528:bool, "error out"=w3523:errorcluster)  [unwired: 5 in, 6 out]
            n1643 = case shown="假" w3528 {
              tunnel: w3527 -> [w3544 _]
              tunnel: w3523 -> [_ _]
              frame False {
                n1644 = call-poly <vilib>:"Read From Spreadsheet File.vi"("file path (dialog if empty)"=w3544) -> ("all rows"=w3547:string[][])  [unwired: 3 in, 7 out]
                n1645 = call <vilib>:"Get File Extension.vi"("file"=w3544) -> ("filename without extension"=w3541:string)  [unwired: 1 in, 9 out]
                n1646 = call <vilib>:"MD5Checksum File.vi"("Path"=w3544) -> ("MD5 message-digest"=w3535:string)  [unwired: 1 in, 9 out]
                n1647 = Index Array(array=w3547, index (col)=0 ("禁用的索引 (列)")) -> (element=w3550:string[])  [unwired: 1 in]
                n1648 = Index Array(array=w3547, index (col)=1 ("禁用的索引 (列)")) -> (element=w3546:string[])  [unwired: 1 in]
                n1649 = Match Pattern(string=w3541, regular expression="(MD5=" ("正则表达式")) -> (offset past match=w3539:i32)  [unwired: 4 out]
                n1650 = Match Pattern(string=w3541, regular expression=")" ("正则表达式")) -> (offset past match=w3540:i32)  [unwired: 4 out]
                n1651 = Subtract(x=w3540, y=w3539) -> (x-y=w3538:i32)
                n1652 = Decrement(x=w3538) -> (x-1=w3537:i32)
                n1653 = String Subset(string=w3541, offset (0)=w3539, length (rest)=w3537) -> (substring=w3536:string)
                n1654 = for {
                  N: 9 -> [_]
                  tunnel: w3550 -> [w3556] mode=indexing
                  tunnel: w3546 -> [w3555] mode=indexing
                  n1655 = case shown="\"配置文件版本号\"" w3556 {
                    tunnel: w3555 -> [_ w3562 w3564 w3570 w3576 w3582 w3588 w3589 w3591]
                    frame "假", Default {
                    }
                    frame "电流分辨率" {
                      n1656 = Equal?(x=w3562, y="0.01") -> (x = y?=w3560:bool)
                      n1657 = Select(t=0.0, s=w3560, f=1.0) -> (s? t:f=w3559:dbl)
                      n1658 = local write "电流分辨率/A"(w3559) -> ()
                    }
                    frame "电压分辨率" {
                      n1659 = Equal?(x=w3564, y="0.01") -> (x = y?=w3567:bool)
                      n1660 = Select(t=0.0, s=w3567, f=1.0) -> (s? t:f=w3563:dbl)
                      n1661 = local write "电压分辨率/V"(w3563) -> ()
                    }
                    frame "安时分辨率" {
                      n1662 = Equal?(x=w3570, y="0.001") -> (x = y?=w3573:bool)
                      n1663 = Select(t=0.0, s=w3573, f=1.0) -> (s? t:f=w3569:dbl)
                      n1664 = local write "安时分辨率/AH"(w3569) -> ()
                    }
                    frame "传感器类型" {
                      n1665 = Equal?(x=w3576, y="霍尔传感器") -> (x = y?=w3579:bool)
                      n1666 = Select(t=0.0, s=w3579, f=1.0) -> (s? t:f=w3575:dbl)
                      n1667 = local write "传感器类型"(w3575) -> ()
                    }
                    frame "是否有外部高压" {
                      n1668 = Equal?(x=w3582, y="有") -> (x = y?=w3585:bool)
                      n1669 = Select(t=0.0, s=w3585, f=1.0) -> (s? t:f=w3581:dbl)
                      n1670 = local write "是否有外部高压"(w3581) -> ()
                    }
                    frame "充放电阈值" {
                      n1671 = Decimal String To Number(string=w3588) -> (number=w3587:i32)  [unwired: 3 out]
                      n1672 = local write "充放电阈值"(w3587) -> ()
                    }
                    frame "配置文件版本号" {
                      n1673 = local write "版本号"(w3589) -> ()
                    }
                    frame "分流器大小" {
                      n1674 = Search 1D Array(1D array=string[] ["50", "100", "200", "300", "400", "500", "600", "700", "800", "900", "1000"], element=w3591) -> (index of element=w3590:i32)  [unwired: 1 out]
                      n1675 = local write "分流器大小/A"(w3590) -> ()
                    }
                  }
                }
                n1676 = Equal?(x=w3535, y=w3536) -> (x = y?=w3532:bool)
                n1677 = case shown="假" w3532 {
                  tunnel: cluster{u32, u32}[] [{6618880, 6618880}] ("颜色[4]") -> [w3551 _]
                  tunnel: cluster{u32, u32}[] [{15663131, 6618880}] ("颜色[4]") -> [_ w3554]
                  tunnel: [w3551 w3554] -> w3531
                  tunnel: ["通过" ("布尔文本.文本") "失败" ("布尔文本.文本")] -> w3530
                  frame True {
                  }
                  frame False {
                  }
                }
                n1678 = property on="导入配置结果" class="Bool (严格)"("Colors [4]"=w3531, "BoolText.Text"=w3530) -> ()  [unwired: 2 in, 2 out]
              }
              frame True {
              }
            }
          }
        }
      }
      event "分流器大小/A": Value Change {
        n1679 = event-data() -> ("NewVal"=w3593:u16)  [unwired: 6 out]
        n1680 = local read "安时分辨率/AH"() -> (w3608:u16)
        n1681 = Equal?(x=w3593, y=u16 0) -> (x = y?=w3606:bool)
        n1682 = Multiply(x=u16 100, y=w3593) -> (x*y=w3603:u16)
        n1683 = Select(t=u16 50 ("y"), s=w3606, f=w3603) -> (s? t:f=w3598:u16)
        n1684 = Equal?(x=w3608, y=u16 0) -> (x = y?=w3601:bool)
        n1685 = Select(t=u16 375 ("y"), s=w3601, f=u32 75006 ("y")) -> (s? t:f=w3597:u32)
        n1686 = Multiply(x=u16 300 ("y"), y=w3597) -> (x*y=w3595:u32)
        n1687 = Divide(x=w3595, y=w3598) -> (x/y=w3594:dbl)
        n1688 = Round To Nearest(number=w3594) -> (nearest integer value=w3609:dbl)
        n1689 = local write "充放电阈值"(w3609) -> ()
      }
      event "安时分辨率/AH": Value Change {
        n1690 = event-data() -> ("NewVal"=w3610:u16)  [unwired: 6 out]
        n1691 = local read "分流器大小/A"() -> (w3626:u16)
        n1692 = Equal?(x=w3626, y=u16 0) -> (x = y?=w3623:bool)
        n1693 = Multiply(x=u16 100, y=w3626) -> (x*y=w3620:u16)
        n1694 = Select(t=u16 50 ("y"), s=w3623, f=w3620) -> (s? t:f=w3615:u16)
        n1695 = Equal?(x=w3610, y=u16 0) -> (x = y?=w3618:bool)
        n1696 = Select(t=u16 375 ("y"), s=w3618, f=u32 75006 ("y")) -> (s? t:f=w3614:u32)
        n1697 = Multiply(x=u16 300 ("y"), y=w3614) -> (x*y=w3612:u32)
        n1698 = Divide(x=w3612, y=w3615) -> (x/y=w3611:dbl)
        n1699 = Round To Nearest(number=w3611) -> (nearest integer value=w3625:dbl)
        n1700 = local write "充放电阈值"(w3625) -> ()
      }
      event "Set Current Offset": Value Change {
        n1701 = event-data() -> ("NewVal"=w3631:bool)  [unwired: 6 out]
        n1702 = case shown="真" w3631 {
          tunnel: w3630 -> [w3633 w3643]
          tunnel: w3629 -> [w3632 w3642]
          tunnel: [w3632 w3641] -> w3628
          tunnel: [w3633 w3640] -> w3627
          frame False {
          }
          frame True {
            n1703 = Enqueue Element(queue=w3643, element="Set Current Offset" ("元素"), error in (no error)=w3642) -> (queue out=w3640:refnum<queue>, error out=w3641:errorcluster)  [unwired: 2 out]
            n1704 = global write "EV05全局变量1.vi" "高压校正接收"(FALSE ("高压校正接收")) -> ()
            n1705 = global write "EV05全局变量1.vi" "CAN接收"(FALSE ("CAN接收")) -> ()
            n1706 = call <vilib>:"Set Busy.vi"() -> ()  [unwired: 4 in, 8 out]
            n1707 = property on="Current Offset结果" class="Bool (严格)"("Colors [4]"=cluster{u32, u32}[] [{0, 0}] ("颜色[4]"), "BoolText.Text"="" ("布尔文本.文本")) -> ()  [unwired: 2 in, 2 out]
            n1708 = local write "电流零点"("" ("5460Current Offset")) -> ()
          }
        }
      }
      event "Set Current Offset 3": Value Change {
        n1709 = event-data() -> ("NewVal"=w3648:bool)  [unwired: 6 out]
        n1710 = case shown="真" w3648 {
          tunnel: w3647 -> [w3650 w3660]
          tunnel: w3646 -> [w3649 w3659]
          tunnel: [w3649 w3658] -> w3645
          tunnel: [w3650 w3657] -> w3644
          frame False {
          }
          frame True {
            n1711 = flat-sequence {
              tunnel: w3659 -> [w3661]
              tunnel: w3660 -> [w3662]
              tunnel: [w3662] -> w3656
              tunnel: [w3661] -> w3655
              tunnel: [w3665] -> w3658
              tunnel: [w3664] -> w3657
              tunnel: w3656 -> [w3667]
              tunnel: w3655 -> [w3666]
              frame #0 {
              }
              frame #1 {
                n1712 = Enqueue Element(queue=w3667, element="Set Current Offset 3" ("元素"), error in (no error)=w3666) -> (queue out=w3664:refnum<queue>, error out=w3665:errorcluster)  [unwired: 2 out]
              }
            }
            n1713 = global write "EV05全局变量1.vi" "CAN接收"(FALSE ("CAN接收")) -> ()
            n1714 = global write "EV05全局变量1.vi" "高压校正接收"(FALSE ("高压校正接收")) -> ()
            n1715 = call <vilib>:"Set Busy.vi"() -> ()  [unwired: 4 in, 8 out]
            n1716 = property on="Current Offset结果 3" class="Bool (严格)"("Colors [4]"=cluster{u32, u32}[] [{0, 0}] ("颜色[4]"), "BoolText.Text"="" ("布尔文本.文本")) -> ()  [unwired: 2 in, 2 out]
          }
        }
      }
      event "充电能量阀值": Value Change {
        n1717 = event-data() -> ("NewVal"=w3672:bool)  [unwired: 6 out]
        n1718 = case shown="真" w3672 {
          tunnel: w3671 -> [w3674 w3684]
          tunnel: w3670 -> [w3673 w3683]
          tunnel: [w3673 w3682] -> w3669
          tunnel: [w3674 w3681] -> w3668
          frame False {
          }
          frame True {
            n1719 = flat-sequence {
              tunnel: w3683 -> [w3685]
              tunnel: w3684 -> [w3686]
              tunnel: [w3686] -> w3680
              tunnel: [w3685] -> w3679
              tunnel: [w3689] -> w3682
              tunnel: [w3688] -> w3681
              tunnel: w3680 -> [w3691]
              tunnel: w3679 -> [w3690]
              frame #0 {
              }
              frame #1 {
                n1720 = Enqueue Element(queue=w3691, element="Set Current Offset 4" ("元素"), error in (no error)=w3690) -> (queue out=w3688:refnum<queue>, error out=w3689:errorcluster)  [unwired: 2 out]
              }
            }
            n1721 = call <vilib>:"Set Busy.vi"() -> ()  [unwired: 4 in, 8 out]
            n1722 = global write "EV05全局变量1.vi" "CAN接收"(FALSE ("CAN接收")) -> ()
            n1723 = global write "EV05全局变量1.vi" "高压校正接收"(FALSE ("高压校正接收")) -> ()
            n1724 = property on="Current Offset结果 4" class="Bool (严格)"("Colors [4]"=cluster{u32, u32}[] [{0, 0}] ("颜色[4]"), "BoolText.Text"="" ("布尔文本.文本")) -> ()  [unwired: 2 in, 2 out]
          }
        }
      }
      event "分流器型号": Value Change {
        n1725 = event-data() -> ("NewVal"=w3696:bool)  [unwired: 6 out]
        n1726 = case shown="真" w3696 {
          tunnel: w3695 -> [w3698 w3707]
          tunnel: w3694 -> [w3697 w3706]
          tunnel: [w3697 w3705] -> w3693
          tunnel: [w3698 w3704] -> w3692
          frame False {
          }
          frame True {
            n1727 = local read "分流器大小"() -> (w3699:T2)
            n1728 = case shown="\"100A\", 默认" w3699 {
              tunnel: w3707 -> [w3711 w3715]
              tunnel: w3706 -> [w3710 w3714]
              tunnel: [w3710 w3713] -> w3705
              tunnel: [w3711 w3712] -> w3704
              frame "选择分流器型号" {
                n1729 = One Button Dialog(message="分流器为无效值" ("消息"), button name ("OK")="确定" ("按钮名称（“确定”）")) -> ()  [unwired: 1 out]
              }
              frame "100A", Default {
                n1730 = flat-sequence {
                  tunnel: w3714 -> [w3718]
                  tunnel: w3715 -> [w3719]
                  tunnel: [w3719] -> w3717
                  tunnel: [w3718] -> w3716
                  tunnel: [w3722] -> w3713
                  tunnel: [w3721] -> w3712
                  tunnel: w3717 -> [w3724]
                  tunnel: w3716 -> [w3723]
                  frame #0 {
                  }
                  frame #1 {
                    n1731 = Enqueue Element(queue=w3724, element="Set Current Gain 4" ("元素"), error in (no error)=w3723) -> (queue out=w3721:refnum<queue>, error out=w3722:errorcluster)  [unwired: 2 out]
                  }
                }
              }
            }
            n1732 = call <vilib>:"Set Busy.vi"() -> ()  [unwired: 4 in, 8 out]
            n1733 = global write "EV05全局变量1.vi" "CAN接收"(FALSE ("CAN接收")) -> ()
            n1734 = global write "EV05全局变量1.vi" "高压校正接收"(FALSE ("高压校正接收")) -> ()
            n1735 = property on="Current Gain结果 4" class="Bool (严格)"("Colors [4]"=cluster{u32, u32}[] [{0, 0}] ("颜色[4]"), "BoolText.Text"="" ("布尔文本.文本")) -> ()  [unwired: 2 in, 2 out]
          }
        }
      }
      event "Set Current Gain 3": Value Change {
        n1736 = event-data() -> ("NewVal"=w3729:bool)  [unwired: 6 out]
        n1737 = case shown="真" w3729 {
          tunnel: w3728 -> [w3731 w3741]
          tunnel: w3727 -> [w3730 w3740]
          tunnel: [w3730 w3739] -> w3726
          tunnel: [w3731 w3738] -> w3725
          frame False {
          }
          frame True {
            n1738 = flat-sequence {
              tunnel: w3740 -> [w3742]
              tunnel: w3741 -> [w3743]
              tunnel: [w3743] -> w3737
              tunnel: [w3742] -> w3736
              tunnel: [w3746] -> w3739
              tunnel: [w3745] -> w3738
              tunnel: w3737 -> [w3748]
              tunnel: w3736 -> [w3747]
              frame #0 {
              }
              frame #1 {
                n1739 = Enqueue Element(queue=w3748, element="Set Current Gain 3" ("元素"), error in (no error)=w3747) -> (queue out=w3745:refnum<queue>, error out=w3746:errorcluster)  [unwired: 2 out]
              }
            }
            n1740 = global write "EV05全局变量1.vi" "CAN接收"(FALSE ("CAN接收")) -> ()
            n1741 = call <vilib>:"Set Busy.vi"() -> ()  [unwired: 4 in, 8 out]
            n1742 = global write "EV05全局变量1.vi" "高压校正接收"(FALSE ("高压校正接收")) -> ()
            n1743 = property on="Current Gain结果 3" class="Bool (严格)"("Colors [4]"=cluster{u32, u32}[] [{0, 0}] ("颜色[4]"), "BoolText.Text"="" ("布尔文本.文本")) -> ()  [unwired: 2 in, 2 out]
          }
        }
      }
      event "Set Current Gain": Value Change {
        n1744 = event-data() -> ("NewVal"=w3753:bool)  [unwired: 6 out]
        n1745 = case shown="真" w3753 {
          tunnel: w3752 -> [w3755 w3766]
          tunnel: w3751 -> [w3754 w3765]
          tunnel: [w3754 w3764] -> w3750
          tunnel: [w3755 w3763] -> w3749
          frame False {
          }
          frame True {
            n1746 = flat-sequence {
              tunnel: w3765 -> [w3767]
              tunnel: w3766 -> [w3768]
              tunnel: [w3768] -> w3762
              tunnel: [w3767] -> w3761
              tunnel: [w3771] -> w3764
              tunnel: [w3770] -> w3763
              tunnel: w3762 -> [w3773]
              tunnel: w3761 -> [w3772]
              frame #0 {
              }
              frame #1 {
                n1747 = Enqueue Element(queue=w3773, element="Set Current Gain" ("元素"), error in (no error)=w3772) -> (queue out=w3770:refnum<queue>, error out=w3771:errorcluster)  [unwired: 2 out]
              }
            }
            n1748 = global write "EV05全局变量1.vi" "CAN接收"(FALSE ("CAN接收")) -> ()
            n1749 = global write "EV05全局变量1.vi" "高压校正接收"(FALSE ("高压校正接收")) -> ()
            n1750 = call <vilib>:"Set Busy.vi"() -> ()  [unwired: 4 in, 8 out]
            n1751 = local write "电流增益"("" ("5460Current Gain")) -> ()
            n1752 = property on="Current Gain结果" class="Bool (严格)"("Colors [4]"=cluster{u32, u32}[] [{0, 0}] ("颜色[4]"), "BoolText.Text"="" ("布尔文本.文本")) -> ()  [unwired: 2 in, 2 out]
          }
        }
      }
      event "Set Current Gain 2": Value Change {
        n1753 = event-data() -> ("NewVal"=w3778:bool)  [unwired: 6 out]
        n1754 = case shown="真" w3778 {
          tunnel: w3777 -> [w3780 w3791]
          tunnel: w3776 -> [w3779 w3790]
          tunnel: [w3779 w3789] -> w3775
          tunnel: [w3780 w3788] -> w3774
          frame False {
          }
          frame True {
            n1755 = flat-sequence {
              tunnel: w3790 -> [w3792]
              tunnel: w3791 -> [w3793]
              tunnel: [w3793] -> w3787
              tunnel: [w3792] -> w3786
              tunnel: [w3796] -> w3789
              tunnel: [w3795] -> w3788
              tunnel: w3787 -> [w3798]
              tunnel: w3786 -> [w3797]
              frame #0 {
              }
              frame #1 {
                n1756 = Enqueue Element(queue=w3798, element="Set Volt Gain" ("元素"), error in (no error)=w3797) -> (queue out=w3795:refnum<queue>, error out=w3796:errorcluster)  [unwired: 2 out]
              }
            }
            n1757 = global write "EV05全局变量1.vi" "CAN接收"(FALSE ("CAN接收")) -> ()
            n1758 = global write "EV05全局变量1.vi" "高压校正接收"(FALSE ("高压校正接收")) -> ()
            n1759 = call <vilib>:"Set Busy.vi"() -> ()  [unwired: 4 in, 8 out]
            n1760 = local write "Shunt Volt Gain"(" " ("5460Volt Gain")) -> ()
            n1761 = property on="Current Gain结果 2" class="Bool (严格)"("Colors [4]"=cluster{u32, u32}[] [{0, 0}] ("颜色[4]"), "BoolText.Text"="" ("布尔文本.文本")) -> ()  [unwired: 2 in, 2 out]
          }
        }
      }
      event "Volt Offset": Value Change {
        n1762 = event-data() -> ("NewVal"=w3803:bool)  [unwired: 6 out]
        n1763 = case shown="真" w3803 {
          tunnel: w3802 -> [w3805 w3816]
          tunnel: w3801 -> [w3804 w3815]
          tunnel: [w3804 w3814] -> w3800
          tunnel: [w3805 w3813] -> w3799
          frame False {
          }
          frame True {
            n1764 = flat-sequence {
              tunnel: w3815 -> [w3817]
              tunnel: w3816 -> [w3818]
              tunnel: [w3818] -> w3812
              tunnel: [w3817] -> w3811
              tunnel: [w3821] -> w3814
              tunnel: [w3820] -> w3813
              tunnel: w3812 -> [w3823]
              tunnel: w3811 -> [w3822]
              frame #0 {
              }
              frame #1 {
                n1765 = Enqueue Element(queue=w3823, element="Set Volt offset" ("元素"), error in (no error)=w3822) -> (queue out=w3820:refnum<queue>, error out=w3821:errorcluster)  [unwired: 2 out]
              }
            }
            n1766 = global write "EV05全局变量1.vi" "CAN接收"(FALSE ("CAN接收")) -> ()
            n1767 = global write "EV05全局变量1.vi" "高压校正接收"(FALSE ("高压校正接收")) -> ()
            n1768 = call <vilib>:"Set Busy.vi"() -> ()  [unwired: 4 in, 8 out]
            n1769 = local write "Shunt Volt Offset"(" " ("5460Volt Offset")) -> ()
            n1770 = property on="Current Offset结果 2" class="Bool (严格)"("Colors [4]"=cluster{u32, u32}[] [{0, 0}] ("颜色[4]"), "BoolText.Text"="" ("布尔文本.文本")) -> ()  [unwired: 2 in, 2 out]
          }
        }
      }
      event "Clear_in": Value Change {
        n1771 = event-data() -> ("NewVal"=w3828:bool)  [unwired: 6 out]
        n1772 = case shown="真" w3828 {
          tunnel: w3827 -> [w3830 w3838]
          tunnel: w3826 -> [w3829 w3837]
          tunnel: [w3829 w3836] -> w3825
          tunnel: [w3830 w3835] -> w3824
          frame False {
          }
          frame True {
            n1773 = flat-sequence {
              tunnel: w3837 -> [w3839]
              tunnel: w3838 -> [w3840]
              tunnel: [w3840] -> w3834
              tunnel: [w3839] -> w3833
              tunnel: [w3843] -> w3836
              tunnel: [w3842] -> w3835
              tunnel: w3834 -> [w3845]
              tunnel: w3833 -> [w3844]
              frame #0 {
              }
              frame #1 {
                n1774 = Enqueue Element(queue=w3845, element="Clear_in" ("元素"), error in (no error)=w3844) -> (queue out=w3842:refnum<queue>, error out=w3843:errorcluster)  [unwired: 2 out]
              }
            }
            n1775 = property on="Clear_in结果" class="Bool (严格)"("Colors [4]"=cluster{u32, u32}[] [{0, 0}] ("颜色[4]"), "BoolText.Text"="" ("布尔文本.文本")) -> ()  [unwired: 2 in, 2 out]
          }
        }
      }
      event "Clear_out": Value Change {
        n1776 = event-data() -> ("NewVal"=w3850:bool)  [unwired: 6 out]
        n1777 = case shown="真" w3850 {
          tunnel: w3849 -> [w3852 w3860]
          tunnel: w3848 -> [w3851 w3859]
          tunnel: [w3851 w3858] -> w3847
          tunnel: [w3852 w3857] -> w3846
          frame False {
          }
          frame True {
            n1778 = flat-sequence {
              tunnel: w3859 -> [w3861]
              tunnel: w3860 -> [w3862]
              tunnel: [w3862] -> w3856
              tunnel: [w3861] -> w3855
              tunnel: [w3865] -> w3858
              tunnel: [w3864] -> w3857
              tunnel: w3856 -> [w3867]
              tunnel: w3855 -> [w3866]
              frame #0 {
              }
              frame #1 {
                n1779 = Enqueue Element(queue=w3867, element="Clear_out" ("元素"), error in (no error)=w3866) -> (queue out=w3864:refnum<queue>, error out=w3865:errorcluster)  [unwired: 2 out]
              }
            }
            n1780 = property on="Clear_out结果" class="Bool (严格)"("Colors [4]"=cluster{u32, u32}[] [{0, 0}] ("颜色[4]"), "BoolText.Text"="" ("布尔文本.文本")) -> ()  [unwired: 2 in, 2 out]
          }
        }
      }
      event "Read1_in": Value Change {
        n1781 = event-data() -> ("NewVal"=w3872:bool)  [unwired: 6 out]
        n1782 = case shown="真" w3872 {
          tunnel: w3871 -> [w3874 w3891]
          tunnel: w3870 -> [w3873 w3890]
          tunnel: [w3873 w3889] -> w3869
          tunnel: [w3874 w3888] -> w3868
          frame False {
          }
          frame True {
            n1783 = flat-sequence {
              tunnel: w3890 -> [w3892]
              tunnel: w3891 -> [w3893]
              tunnel: [w3893] -> w3881
              tunnel: [w3892] -> w3879
              tunnel: w3881 -> [w3895]
              tunnel: [w3895] -> w3880
              tunnel: w3879 -> [w3894]
              tunnel: [w3894] -> w3878
              tunnel: w3880 -> [w3897]
              tunnel: [w3897] -> w3885
              tunnel: w3878 -> [w3896]
              tunnel: [w3896] -> w3883
              tunnel: w3885 -> [w3899]
              tunnel: [w3899] -> w3884
              tunnel: w3883 -> [w3898]
              tunnel: [w3898] -> w3882
              tunnel: [w3902] -> w3889
              tunnel: [w3901] -> w3888
              tunnel: w3884 -> [w3904]
              tunnel: w3882 -> [w3903]
              frame #0 {
              }
              frame #1 {
              }
              frame #2 {
              }
              frame #3 {
              }
              frame #4 {
                n1784 = Enqueue Element(queue=w3904, element="Read1_in" ("元素"), error in (no error)=w3903) -> (queue out=w3901:refnum<queue>, error out=w3902:errorcluster)  [unwired: 2 out]
              }
            }
            n1785 = global write "EV05全局变量1.vi" "高压校正接收"(FALSE ("高压校正接收")) -> ()
            n1786 = local write "AD1"(0.0 ("AD1 2")) -> ()
            n1787 = global write "EV05全局变量1.vi" "CAN接收"(FALSE ("CAN接收")) -> ()
            n1788 = call <vilib>:"Set Busy.vi"() -> ()  [unwired: 4 in, 8 out]
            n1789 = property on="Read1_in结果" class="Bool (严格)"("Colors [4]"=cluster{u32, u32}[] [{0, 0}] ("颜色[4]"), "BoolText.Text"="" ("布尔文本.文本")) -> ()  [unwired: 2 in, 2 out]
          }
        }
      }
      event "Read2_in": Value Change {
        n1790 = event-data() -> ("NewVal"=w3909:bool)  [unwired: 6 out]
        n1791 = case shown="真" w3909 {
          tunnel: w3908 -> [w3911 w3928]
          tunnel: w3907 -> [w3910 w3927]
          tunnel: [w3910 w3926] -> w3906
          tunnel: [w3911 w3925] -> w3905
          frame False {
          }
          frame True {
            n1792 = flat-sequence {
              tunnel: w3927 -> [w3929]
              tunnel: w3928 -> [w3930]
              tunnel: [w3930] -> w3918
              tunnel: [w3929] -> w3916
              tunnel: w3918 -> [w3932]
              tunnel: [w3932] -> w3917
              tunnel: w3916 -> [w3931]
              tunnel: [w3931] -> w3915
              tunnel: w3917 -> [w3934]
              tunnel: [w3934] -> w3922
              tunnel: w3915 -> [w3933]
              tunnel: [w3933] -> w3920
              tunnel: w3922 -> [w3936]
              tunnel: [w3936] -> w3921
              tunnel: w3920 -> [w3935]
              tunnel: [w3935] -> w3919
              tunnel: [w3939] -> w3926
              tunnel: [w3938] -> w3925
              tunnel: w3921 -> [w3941]
              tunnel: w3919 -> [w3940]
              frame #0 {
              }
              frame #1 {
              }
              frame #2 {
              }
              frame #3 {
              }
              frame #4 {
                n1793 = Enqueue Element(queue=w3941, element="Read2_in" ("元素"), error in (no error)=w3940) -> (queue out=w3938:refnum<queue>, error out=w3939:errorcluster)  [unwired: 2 out]
              }
            }
            n1794 = global write "EV05全局变量1.vi" "高压校正接收"(FALSE ("高压校正接收")) -> ()
            n1795 = global write "EV05全局变量1.vi" "CAN接收"(FALSE ("CAN接收")) -> ()
            n1796 = local write "AD2"(0.0 ("AD2 2")) -> ()
            n1797 = call <vilib>:"Set Busy.vi"() -> ()  [unwired: 4 in, 8 out]
            n1798 = property on="Read2_in结果" class="Bool (严格)"("Colors [4]"=cluster{u32, u32}[] [{0, 0}] ("颜色[4]"), "BoolText.Text"="" ("布尔文本.文本")) -> ()  [unwired: 2 in, 2 out]
          }
        }
      }
      event "Read2": Value Change {
        n1799 = event-data() -> ("NewVal"=w3946:bool)  [unwired: 6 out]
        n1800 = case shown="真" w3946 {
          tunnel: w3945 -> [w3948 w3965]
          tunnel: w3944 -> [w3947 w3964]
          tunnel: [w3947 w3963] -> w3943
          tunnel: [w3948 w3962] -> w3942
          frame False {
          }
          frame True {
            n1801 = flat-sequence {
              tunnel: w3964 -> [w3966]
              tunnel: w3965 -> [w3967]
              tunnel: [w3967] -> w3959
              tunnel: [w3966] -> w3957
              tunnel: w3959 -> [w3969]
              tunnel: [w3969] -> w3958
              tunnel: w3957 -> [w3968]
              tunnel: [w3968] -> w3956
              tunnel: w3958 -> [w3971]
              tunnel: [w3971] -> w3955
              tunnel: w3956 -> [w3970]
              tunnel: [w3970] -> w3953
              tunnel: w3955 -> [w3973]
              tunnel: [w3973] -> w3954
              tunnel: w3953 -> [w3972]
              tunnel: [w3972] -> w3952
              tunnel: [w3978] -> w3963
              tunnel: [w3977] -> w3962
              tunnel: w3954 -> [w3980]
              tunnel: w3952 -> [w3979]
              frame #0 {
              }
              frame #1 {
              }
              frame #2 {
              }
              frame #3 {
                n1802 = disable-structure shown="禁用" {
                  frame Disabled {
                    n1803 = local read "自动控制仪器"() -> (w3974:bool)
                    n1804 = case shown="真" w3974 {
                      frame False {
                      }
                      frame True {
                        n1805 = Wait (ms)(milliseconds to wait=u32 2000 ("等待时间（毫秒）")) -> ()  [unwired: 1 out]
                      }
                    }
                  }
                  frame Enabled {
                  }
                }
              }
              frame #4 {
                n1806 = Enqueue Element(queue=w3980, element="Read2" ("元素"), error in (no error)=w3979) -> (queue out=w3977:refnum<queue>, error out=w3978:errorcluster)  [unwired: 2 out]
              }
            }
            n1807 = global write "EV05全局变量1.vi" "高压校正接收"(FALSE ("高压校正接收")) -> ()
            n1808 = global write "EV05全局变量1.vi" "CAN接收"(FALSE ("CAN接收")) -> ()
            n1809 = local write "AD2"(u16 0 ("AD2")) -> ()
            n1810 = call <vilib>:"Set Busy.vi"() -> ()  [unwired: 4 in, 8 out]
            n1811 = property on="Read2结果" class="Bool (严格)"("Colors [4]"=cluster{u32, u32}[] [{0, 0}] ("颜色[4]"), "BoolText.Text"="" ("布尔文本.文本")) -> ()  [unwired: 2 in, 2 out]
          }
        }
      }
      event "Set": Value Change {
        n1812 = event-data() -> ("NewVal"=w3985:bool)  [unwired: 6 out]
        n1813 = case shown="真" w3985 {
          tunnel: w3984 -> [w3987 w3997]
          tunnel: w3983 -> [w3986 w3996]
          tunnel: [w3986 w3995] -> w3982
          tunnel: [w3987 w3994] -> w3981
          frame False {
          }
          frame True {
            n1814 = flat-sequence {
              tunnel: w3996 -> [w4008]
              tunnel: w3997 -> [w4009]
              tunnel: [w4009] -> w3993
              tunnel: [w4008] -> w3992
              tunnel: [w4012] -> w3995
              tunnel: [w4011] -> w3994
              tunnel: w3993 -> [w4014]
              tunnel: w3992 -> [w4013]
              frame #0 {
                n1815 = local read "REAL2"() -> (w4006:dbl)
                n1816 = local read "REAL1"() -> (w4005:dbl)
                n1817 = local read "AD1"() -> (w4001:u16)
                n1818 = local read "AD2"() -> (w4002:u16)
                n1819 = Subtract(x=w4006, y=w4005) -> (x-y=w4004:dbl)
                n1820 = Subtract(x=w4002, y=w4001) -> (x-y=w4000:u16)
                n1821 = Multiply(x=w4004, y=1000000.0) -> (x*y=w4003:dbl)
                n1822 = Divide(x=w4003, y=w4000) -> (x/y=w3999:dbl)
                n1823 = Round Toward -Infinity(1:w3999) -> (0:w3998:dbl)
                n1824 = local write "Gain"(w3998) -> ()
              }
              frame #1 {
                n1825 = Enqueue Element(queue=w4014, element="Set" ("元素"), error in (no error)=w4013) -> (queue out=w4011:refnum<queue>, error out=w4012:errorcluster)  [unwired: 2 out]
              }
            }
            n1826 = global write "EV05全局变量1.vi" "CAN接收"(FALSE ("CAN接收")) -> ()
            n1827 = global write "EV05全局变量1.vi" "高压校正接收"(FALSE ("高压校正接收")) -> ()
            n1828 = call <vilib>:"Set Busy.vi"() -> ()  [unwired: 4 in, 8 out]
            n1829 = property on="Set结果" class="Bool (严格)"("Colors [4]"=cluster{u32, u32}[] [{0, 0}] ("颜色[4]"), "BoolText.Text"="" ("布尔文本.文本")) -> ()  [unwired: 2 in, 2 out]
          }
        }
      }
      event "Set_in": Value Change {
        n1830 = event-data() -> ("NewVal"=w4019:bool)  [unwired: 6 out]
        n1831 = case shown="真" w4019 {
          tunnel: w4018 -> [w4021 w4031]
          tunnel: w4017 -> [w4020 w4030]
          tunnel: [w4020 w4029] -> w4016
          tunnel: [w4021 w4028] -> w4015
          frame False {
          }
          frame True {
            n1832 = flat-sequence {
              tunnel: w4030 -> [w4038]
              tunnel: w4031 -> [w4039]
              tunnel: [w4039] -> w4027
              tunnel: [w4038] -> w4026
              tunnel: [w4042] -> w4029
              tunnel: [w4041] -> w4028
              tunnel: w4027 -> [w4044]
              tunnel: w4026 -> [w4043]
              frame #0 {
                n1833 = local read "REAL2"() -> (w4036:dbl)
                n1834 = local read "REAL1"() -> (w4037:dbl)
                n1835 = local read "AD1"() -> (w4035:dbl)
                n1836 = local read "AD2"() -> (w4034:dbl)
                n1837 = call "Cal_Gain&offset.vi"("REAL2"=w4036, "REAL1"=w4037, "AD2"=w4034, "AD1"=w4035) -> ("Offset"=w4032:i32, "Gain"=w4033:dbl)  [unwired: 5 out]
                n1838 = local write "Gain"(w4033) -> ()
                n1839 = local write "Offset"(w4032) -> ()
              }
              frame #1 {
                n1840 = Enqueue Element(queue=w4044, element="Set_in" ("元素"), error in (no error)=w4043) -> (queue out=w4041:refnum<queue>, error out=w4042:errorcluster)  [unwired: 2 out]
              }
            }
            n1841 = global write "EV05全局变量1.vi" "CAN接收"(FALSE ("CAN接收")) -> ()
            n1842 = global write "EV05全局变量1.vi" "高压校正接收"(FALSE ("高压校正接收")) -> ()
            n1843 = call <vilib>:"Set Busy.vi"() -> ()  [unwired: 4 in, 8 out]
            n1844 = property on="Set_in结果" class="Bool (严格)"("Colors [4]"=cluster{u32, u32}[] [{0, 0}] ("颜色[4]"), "BoolText.Text"="" ("布尔文本.文本")) -> ()  [unwired: 2 in, 2 out]
          }
        }
      }
      event "连接GPIB": Value Change {
        n1845 = event-data() -> ("NewVal"=w4047:bool)  [unwired: 6 out]
        n1846 = case shown="真" w4047 {
          tunnel: w4046 -> [w4049 w4079]
          tunnel: [w4048 w4080] -> w4045
          frame False {
            w4051 = u8 2 ("禁用")
            n1847 = property on="输出100A" class="Bool"("Disabled"=w4051) -> ()  [unwired: 2 in, 2 out]
            n1848 = property on="输出200A" class="Bool"("Disabled"=w4051) -> ()  [unwired: 2 in, 2 out]
            n1849 = property on="输出自定义值2 2" class="Bool"("Disabled"=w4051) -> ()  [unwired: 2 in, 2 out]
            n1850 = property on="输出自定义值1 2" class="Bool"("Disabled"=w4051) -> ()  [unwired: 2 in, 2 out]
            n1851 = invoke on="输出200A" class="Bool" method="Reinit To Default"() -> ()  [unwired: 3 in, 3 out]
            n1852 = invoke on="输出100A" class="Bool" method="Reinit To Default"() -> ()  [unwired: 3 in, 3 out]
            n1853 = invoke on="输出自定义值2 2" class="Bool" method="Reinit To Default"() -> ()  [unwired: 3 in, 3 out]
            n1854 = invoke on="输出自定义值1 2" class="Bool" method="Reinit To Default"() -> ()  [unwired: 3 in, 3 out]
            n1855 = local read "VISA资源名称输出"() -> (w4056:refnum<visa-resource-name>)
            n1856 = flat-sequence {
              tunnel: w4056 -> [w4060]
              tunnel: [w4060] -> w4058
              tunnel: w4058 -> [w4062]
              tunnel: [w4062] -> w4057
              tunnel: w4057 -> [w4067]
              tunnel: [w4066] -> w4053
              tunnel: [w4065] -> w4052
              tunnel: [w4064] -> w4050
              tunnel: w4049 -> [w4063]
              tunnel: [w4072] -> w4054
              tunnel: [w4071] -> w4055
              tunnel: w4053 -> [w4074]
              tunnel: w4052 -> [w4073]
              tunnel: w4050 -> [w4070]
              frame #0 {
                n1857 = local write "连接状态 10"(FALSE ("连接状态")) -> ()
              }
              frame #1 {
                n1858 = Wait (ms)(milliseconds to wait=u32 50 ("等待时间（毫秒）")) -> ()  [unwired: 1 out]
              }
              frame #2 {
                w4064 = "outp off" ("写入缓冲区")
                n1859 = VISA Write(VISA resource name=w4067, write buffer=w4064, error in (no error)=w4063) -> (VISA resource name out=w4066:refnum<visa-resource-name>, error out=w4065:errorcluster)  [unwired: 1 out]
              }
              frame #3 {
                n1860 = VISA Write(VISA resource name=w4074, write buffer=w4070, error in (no error)=w4073) -> (VISA resource name out=w4071:refnum<visa-resource-name>, error out=w4072:errorcluster)  [unwired: 1 out]
                n1861 = local write "Actual"(0.0 ("实际值")) -> ()
                n1862 = Wait (ms)(milliseconds to wait=u32 50 ("等待时间（毫秒）")) -> ()  [unwired: 1 out]
                n1863 = local write "Set"(0.0 ("设定值")) -> ()
              }
            }
            n1864 = VISA Close(VISA resource name=w4055, error in (no error)=w4054) -> (error out=w4048:errorcluster)
          }
          frame True {
            n1865 = VISA Open(error in (no error)=w4079, VISA resource name="VISA resource name 2") -> (VISA resource name=w4077:refnum<visa-resource-name>, error out=w4083:errorcluster)  [unwired: 3 out]
            n1866 = property class="Instr"(reference=w4077, "Timeout"=u32 100 ("General Settings:Timeout Value")) -> (reference out=w4076:refnum<visa-resource-name>)  [unwired: 1 in, 1 out]
            n1867 = VISA Write(VISA resource name=w4076, write buffer="*rst" ("写入缓冲区"), error in (no error)=w4083) -> (VISA resource name out=w4082:refnum<visa-resource-name>, error out=w4080:errorcluster)  [unwired: 1 out]
            n1868 = Unbundle(w4080) -> ("status"=w4085:bool)  [unwired: 2 out]
            n1869 = case shown="假" w4085 {
              tunnel: w4082 -> [w4089 w4092]
              frame False {
                w4087 = u8 0 ("禁用")
                n1870 = local write "VISA资源名称输出"(w4089) -> ()
                n1871 = local write "连接状态 10"(TRUE ("连接状态")) -> ()
                n1872 = property on="连接状态 10" class="Bool (严格)"("Colors [4]"=cluster{u32, u32}[] [{6618880, 6618880}] ("颜色[4]")) -> ()  [unwired: 2 in, 2 out]
                n1873 = property on="输出100A" class="Bool"("Disabled"=w4087) -> ()  [unwired: 2 in, 2 out]
                n1874 = property on="输出200A" class="Bool"("Disabled"=w4087) -> ()  [unwired: 2 in, 2 out]
                n1875 = property on="输出自定义值2 2" class="Bool"("Disabled"=w4087) -> ()  [unwired: 2 in, 2 out]
                n1876 = property on="输出自定义值1 2" class="Bool"("Disabled"=w4087) -> ()  [unwired: 2 in, 2 out]
              }
              frame True {
                w4091 = u8 2 ("禁用")
                n1877 = local write "VISA资源名称输出"(w4092) -> ()
                n1878 = local write "连接状态 10"(FALSE ("连接状态")) -> ()
                n1879 = property on="连接状态 10" class="Bool (严格)"("Colors [4]"=cluster{u32, u32}[] [{15663131, 6618880}] ("颜色[4]")) -> ()  [unwired: 2 in, 2 out]
                n1880 = property on="输出100A" class="Bool"("Disabled"=w4091) -> ()  [unwired: 2 in, 2 out]
                n1881 = property on="输出200A" class="Bool"("Disabled"=w4091) -> ()  [unwired: 2 in, 2 out]
                n1882 = property on="输出自定义值2 2" class="Bool"("Disabled"=w4091) -> ()  [unwired: 2 in, 2 out]
                n1883 = property on="输出自定义值1 2" class="Bool"("Disabled"=w4091) -> ()  [unwired: 2 in, 2 out]
              }
            }
          }
        }
      }
      event "输出自定义值1": Value Change {
        n1884 = event-data() -> ("NewVal"=w4096:bool)  [unwired: 6 out]
        n1885 = case shown="真" w4096 {
          tunnel: w4095 -> [w4098 w4122]
          tunnel: [w4097 w4123] -> w4094
          frame False {
            w4099 = u8 0 ("禁用")
            n1886 = local read "VISA资源名称输出 10"() -> (w4105:refnum<visa-resource-name>)
            n1887 = local write "控制读取  5"(FALSE ("控制读取")) -> ()
            n1888 = flat-sequence {
              tunnel: [w4108] -> w4106
              tunnel: w4105 -> [w4108]
              tunnel: w4106 -> [w4112]
              tunnel: [w4111] -> w4104
              tunnel: [w4110] -> w4103
              tunnel: w4098 -> [w4109]
              tunnel: w4104 -> [w4116]
              tunnel: w4103 -> [w4115]
              tunnel: [w4116] -> w4102
              tunnel: [w4115] -> w4101
              tunnel: w4102 -> [w4120]
              tunnel: w4101 -> [w4119]
              tunnel: [w4117] -> w4097
              frame #0 {
                n1889 = Wait (ms)(milliseconds to wait=u32 200 ("等待时间（毫秒）")) -> ()  [unwired: 1 out]
              }
              frame #1 {
                n1890 = VISA Write(VISA resource name=w4112, write buffer="OUT:OFF" ("写入缓冲区"), error in (no error)=w4109) -> (VISA resource name out=w4111:refnum<visa-resource-name>, error out=w4110:errorcluster)  [unwired: 1 out]
              }
              frame #2 {
                n1891 = Wait (ms)(milliseconds to wait=u32 50 ("等待时间（毫秒）")) -> ()  [unwired: 1 out]
              }
              frame #3 {
                n1892 = local write "控制读取  5"(TRUE ("控制读取")) -> ()
                n1893 = VISA Write(VISA resource name=w4120, write buffer="OUT:OFF" ("写入缓冲区"), error in (no error)=w4119) -> (error out=w4117:errorcluster)  [unwired: 2 out]
              }
            }
            n1894 = property on="输出150V" class="Bool"("Disabled"=w4099) -> ()  [unwired: 2 in, 2 out]
            n1895 = property on="输出300V" class="Bool"("Disabled"=w4099) -> ()  [unwired: 2 in, 2 out]
            n1896 = property on="输出自定义值2" class="Bool"("Disabled"=w4099) -> ()  [unwired: 2 in, 2 out]
            n1897 = property on="输出自定义值1" class="Bool"("Disabled"=w4099) -> ()  [unwired: 2 in, 2 out]
          }
          frame True {
            w4132 = u8 2 ("禁用")
            w4134 = "," ("字符串")
            n1898 = local read "Volt1"() -> (w4125:dbl)
            n1899 = local write "Set"(w4125) -> ()
            n1900 = local write "控制读取  5"(FALSE ("控制读取")) -> ()
            n1901 = property on="输出150V" class="Bool"("Disabled"=w4132) -> ()  [unwired: 2 in, 2 out]
            n1902 = property on="输出300V" class="Bool"("Disabled"=w4132) -> ()  [unwired: 2 in, 2 out]
            n1903 = property on="输出自定义值2" class="Bool"("Disabled"=w4132) -> ()  [unwired: 2 in, 2 out]
            n1904 = Number To Fractional String(number=w4125, precision (6)=i16 2 ("精度(6)")) -> (F-format string=w4138:string)  [unwired: 2 out]
            n1905 = Number To Fractional String(number=0.2 ("数字"), precision (6)=i16 2 ("精度(6)")) -> (F-format string=w4137:string)  [unwired: 2 out]
            n1906 = Number To Fractional String(number=1.0 ("数字"), precision (6)=i16 2 ("精度(6)")) -> (F-format string=w4135:string)  [unwired: 2 out]
            n1907 = Number To Fractional String(number=320.0 ("数字"), precision (6)=i16 2 ("精度(6)")) -> (F-format string=w4136:string)  [unwired: 2 out]
            n1908 = Concatenate Strings(w4138, w4134, w4137, w4134, w4136, w4134, w4135, w4134, w4134, w4134) -> (w4133:string)
            n1909 = flat-sequence {
              tunnel: [w4157] -> w4145
              tunnel: [w4156] -> w4143
              tunnel: [w4155] -> w4141
              tunnel: w4133 -> [w4152]
              tunnel: w4122 -> [w4151]
              tunnel: w4145 -> [w4162]
              tunnel: [w4162] -> w4144
              tunnel: w4143 -> [w4161]
              tunnel: [w4161] -> w4142
              tunnel: w4141 -> [w4160]
              tunnel: [w4160] -> w4140
              tunnel: w4144 -> [w4166]
              tunnel: w4142 -> [w4165]
              tunnel: w4140 -> [_]
              tunnel: [w4164] -> w4149
              tunnel: [w4163] -> w4147
              tunnel: w4149 -> [w4172]
              tunnel: [w4172] -> w4148
              tunnel: w4147 -> [w4171]
              tunnel: [w4171] -> w4146
              tunnel: w4148 -> [w4175]
              tunnel: w4146 -> [w4174]
              tunnel: [w4173] -> w4123
              frame #0 {
                n1910 = Wait (ms)(milliseconds to wait=u32 200 ("等待时间（毫秒）")) -> ()  [unwired: 1 out]
              }
              frame #1 {
                n1911 = local read "VISA资源名称输出 10"() -> (w4154:refnum<visa-resource-name>)
                n1912 = Concatenate Strings("SET:GRO 12," ("写入缓冲区"), w4152, "\n") -> (w4155:string)
                n1913 = VISA Write(VISA resource name=w4154, write buffer=w4155, error in (no error)=w4151) -> (VISA resource name out=w4157:refnum<visa-resource-name>, error out=w4156:errorcluster)  [unwired: 1 out]
              }
              frame #2 {
                n1914 = Wait (ms)(milliseconds to wait=u32 50 ("等待时间（毫秒）")) -> ()  [unwired: 1 out]
              }
              frame #3 {
                n1915 = Concatenate Strings("SET:STE 12" ("写入缓冲区"), "\n") -> (w4167:string)
                n1916 = VISA Write(VISA resource name=w4166, write buffer=w4167, error in (no error)=w4165) -> (VISA resource name out=w4164:refnum<visa-resource-name>, error out=w4163:errorcluster)  [unwired: 1 out]
              }
              frame #4 {
                n1917 = Wait (ms)(milliseconds to wait=u32 200 ("等待时间（毫秒）")) -> ()  [unwired: 1 out]
              }
              frame #5 {
                n1918 = Concatenate Strings("OUT:ON" ("写入缓冲区"), "\n") -> (w4180:string)
                n1919 = Wait (ms)(milliseconds to wait=u32 50 ("等待时间（毫秒）")) -> ()  [unwired: 1 out]
                n1920 = VISA Write(VISA resource name=w4175, write buffer=w4180, error in (no error)=w4174) -> (VISA resource name out=w4177:refnum<visa-resource-name>, error out=w4173:errorcluster)  [unwired: 1 out]
                n1921 = local write "VISA资源名称输出 10"(w4177) -> ()
              }
              frame #6 {
                n1922 = local write "控制读取  5"(TRUE ("控制读取")) -> ()
              }
            }
          }
        }
      }
      event "输出自定义值2": Value Change {
        n1923 = event-data() -> ("NewVal"=w4184:bool)  [unwired: 6 out]
        n1924 = case shown="真" w4184 {
          tunnel: w4183 -> [w4185 w4214]
          tunnel: [w4187 w4212] -> w4182
          frame False {
            w4188 = u8 0 ("禁用")
            n1925 = local read "VISA资源名称输出 10"() -> (w4194:refnum<visa-resource-name>)
            n1926 = local write "控制读取  5"(FALSE ("控制读取")) -> ()
            n1927 = flat-sequence {
              tunnel: [w4198] -> w4195
              tunnel: w4194 -> [w4198]
              tunnel: [w4196] -> w4186
              tunnel: w4185 -> [w4196]
              tunnel: w4195 -> [w4202]
              tunnel: [w4201] -> w4193
              tunnel: [w4200] -> w4192
              tunnel: w4186 -> [w4199]
              tunnel: w4193 -> [w4206]
              tunnel: w4192 -> [w4205]
              tunnel: [w4206] -> w4191
              tunnel: [w4205] -> w4190
              tunnel: w4191 -> [w4210]
              tunnel: w4190 -> [w4209]
              tunnel: [w4207] -> w4187
              frame #0 {
                n1928 = Wait (ms)(milliseconds to wait=u32 200 ("等待时间（毫秒）")) -> ()  [unwired: 1 out]
              }
              frame #1 {
                n1929 = VISA Write(VISA resource name=w4202, write buffer="OUT:OFF" ("写入缓冲区"), error in (no error)=w4199) -> (VISA resource name out=w4201:refnum<visa-resource-name>, error out=w4200:errorcluster)  [unwired: 1 out]
              }
              frame #2 {
                n1930 = Wait (ms)(milliseconds to wait=u32 50 ("等待时间（毫秒）")) -> ()  [unwired: 1 out]
              }
              frame #3 {
                n1931 = local write "控制读取  5"(TRUE ("控制读取")) -> ()
                n1932 = VISA Write(VISA resource name=w4210, write buffer="OUT:OFF" ("写入缓冲区"), error in (no error)=w4209) -> (error out=w4207:errorcluster)  [unwired: 2 out]
              }
            }
            n1933 = property on="输出150V" class="Bool"("Disabled"=w4188) -> ()  [unwired: 2 in, 2 out]
            n1934 = property on="输出300V" class="Bool"("Disabled"=w4188) -> ()  [unwired: 2 in, 2 out]
            n1935 = property on="输出自定义值2" class="Bool"("Disabled"=w4188) -> ()  [unwired: 2 in, 2 out]
            n1936 = property on="输出自定义值1" class="Bool"("Disabled"=w4188) -> ()  [unwired: 2 in, 2 out]
          }
          frame True {
            w4219 = i16 2 ("精度(6)")
            w4220 = u8 2 ("禁用")
            w4222 = "," ("字符串")
            n1937 = local read "Volt2"() -> (w4216:dbl)
            n1938 = local write "控制读取  5"(FALSE ("控制读取")) -> ()
            n1939 = property on="输出150V" class="Bool"("Disabled"=w4220) -> ()  [unwired: 2 in, 2 out]
            n1940 = property on="输出300V" class="Bool"("Disabled"=w4220) -> ()  [unwired: 2 in, 2 out]
            n1941 = property on="输出自定义值1" class="Bool"("Disabled"=w4220) -> ()  [unwired: 2 in, 2 out]
            n1942 = Number To Fractional String(number=w4216, precision (6)=w4219) -> (F-format string=w4226:string)  [unwired: 2 out]
            n1943 = Number To Fractional String(number=0.2 ("数字"), precision (6)=w4219) -> (F-format string=w4225:string)  [unwired: 2 out]
            n1944 = Number To Fractional String(number=1.0 ("数字"), precision (6)=w4219) -> (F-format string=w4223:string)  [unwired: 2 out]
            n1945 = Number To Fractional String(number=320.0 ("数字"), precision (6)=w4219) -> (F-format string=w4224:string)  [unwired: 2 out]
            n1946 = local write "Set"(w4216) -> ()
            n1947 = Concatenate Strings(w4226, w4222, w4225, w4222, w4224, w4222, w4223, w4222, w4222, w4222) -> (w4221:string)
            n1948 = flat-sequence {
              tunnel: [w4245] -> w4233
              tunnel: [w4244] -> w4231
              tunnel: [w4243] -> w4229
              tunnel: w4221 -> [w4240]
              tunnel: w4214 -> [w4239]
              tunnel: w4233 -> [w4250]
              tunnel: [w4250] -> w4232
              tunnel: w4231 -> [w4249]
              tunnel: [w4249] -> w4230
              tunnel: w4229 -> [w4248]
              tunnel: [w4248] -> w4228
              tunnel: w4232 -> [w4254]
              tunnel: w4230 -> [w4253]
              tunnel: w4228 -> [_]
              tunnel: [w4252] -> w4237
              tunnel: [w4251] -> w4235
              tunnel: w4237 -> [w4260]
              tunnel: [w4260] -> w4236
              tunnel: w4235 -> [w4259]
              tunnel: [w4259] -> w4234
              tunnel: w4236 -> [w4263]
              tunnel: w4234 -> [w4262]
              tunnel: [w4261] -> w4213
              tunnel: w4213 -> [w4269]
              tunnel: [w4269] -> w4212
              frame #0 {
                n1949 = Wait (ms)(milliseconds to wait=u32 200 ("等待时间（毫秒）")) -> ()  [unwired: 1 out]
              }
              frame #1 {
                n1950 = local read "VISA资源名称输出 10"() -> (w4242:refnum<visa-resource-name>)
                n1951 = Concatenate Strings("SET:GRO 12," ("写入缓冲区"), w4240, "\n") -> (w4243:string)
                n1952 = VISA Write(VISA resource name=w4242, write buffer=w4243, error in (no error)=w4239) -> (VISA resource name out=w4245:refnum<visa-resource-name>, error out=w4244:errorcluster)  [unwired: 1 out]
              }
              frame #2 {
                n1953 = Wait (ms)(milliseconds to wait=u32 50 ("等待时间（毫秒）")) -> ()  [unwired: 1 out]
              }
              frame #3 {
                n1954 = Concatenate Strings("SET:STE 12" ("写入缓冲区"), "\n") -> (w4255:string)
                n1955 = VISA Write(VISA resource name=w4254, write buffer=w4255, error in (no error)=w4253) -> (VISA resource name out=w4252:refnum<visa-resource-name>, error out=w4251:errorcluster)  [unwired: 1 out]
              }
              frame #4 {
                n1956 = Wait (ms)(milliseconds to wait=u32 200 ("等待时间（毫秒）")) -> ()  [unwired: 1 out]
              }
              frame #5 {
                n1957 = Concatenate Strings("OUT:ON" ("写入缓冲区"), "\n") -> (w4268:string)
                n1958 = Wait (ms)(milliseconds to wait=u32 50 ("等待时间（毫秒）")) -> ()  [unwired: 1 out]
                n1959 = VISA Write(VISA resource name=w4263, write buffer=w4268, error in (no error)=w4262) -> (VISA resource name out=w4265:refnum<visa-resource-name>, error out=w4261:errorcluster)  [unwired: 1 out]
                n1960 = local write "VISA资源名称输出 10"(w4265) -> ()
              }
              frame #6 {
                n1961 = local write "控制读取  5"(TRUE ("控制读取")) -> ()
              }
            }
          }
        }
      }
      event "连接电压源": Value Change {
        n1962 = event-data() -> ("NewVal"=w4273:bool)  [unwired: 6 out]
        n1963 = case shown="真" w4273 {
          tunnel: [w4277 w4307] -> w4272
          tunnel: w4271 -> [w4276 w4306]
          frame False {
            w4278 = u8 2 ("禁用")
            n1964 = property on="输出150V" class="Bool"("Disabled"=w4278) -> ()  [unwired: 2 in, 2 out]
            n1965 = property on="输出300V" class="Bool"("Disabled"=w4278) -> ()  [unwired: 2 in, 2 out]
            n1966 = property on="输出自定义值2" class="Bool"("Disabled"=w4278) -> ()  [unwired: 2 in, 2 out]
            n1967 = property on="输出自定义值1" class="Bool"("Disabled"=w4278) -> ()  [unwired: 2 in, 2 out]
            n1968 = invoke on="输出300V" class="Bool" method="Reinit To Default"() -> ()  [unwired: 3 in, 3 out]
            n1969 = invoke on="输出150V" class="Bool" method="Reinit To Default"() -> ()  [unwired: 3 in, 3 out]
            n1970 = invoke on="输出自定义值2" class="Bool" method="Reinit To Default"() -> ()  [unwired: 3 in, 3 out]
            n1971 = invoke on="输出自定义值1" class="Bool" method="Reinit To Default"() -> ()  [unwired: 3 in, 3 out]
            n1972 = local read "VISA资源名称输出 10"() -> (w4283:refnum<visa-resource-name>)
            n1973 = flat-sequence {
              tunnel: w4283 -> [w4288]
              tunnel: [w4288] -> w4285
              tunnel: w4276 -> [w4286]
              tunnel: [w4286] -> w4274
              tunnel: w4285 -> [w4291]
              tunnel: [w4291] -> w4284
              tunnel: [w4289] -> w4275
              tunnel: w4274 -> [w4289]
              tunnel: w4284 -> [w4295]
              tunnel: [w4294] -> w4280
              tunnel: [w4293] -> w4279
              tunnel: w4275 -> [w4292]
              tunnel: [w4299] -> w4281
              tunnel: [w4300] -> w4282
              tunnel: w4280 -> [w4300]
              tunnel: w4279 -> [w4299]
              frame #0 {
                n1974 = local write "连接状态 10"(FALSE ("连接状态")) -> ()
              }
              frame #1 {
                n1975 = Wait (ms)(milliseconds to wait=u32 50 ("等待时间（毫秒）")) -> ()  [unwired: 1 out]
              }
              frame #2 {
                n1976 = VISA Write(VISA resource name=w4295, write buffer="OUT:OFF" ("写入缓冲区"), error in (no error)=w4292) -> (VISA resource name out=w4294:refnum<visa-resource-name>, error out=w4293:errorcluster)  [unwired: 1 out]
              }
              frame #3 {
                w4297 = 0.0 ("电压/V")
                n1977 = local write "电流/A 4"(w4297) -> ()
                n1978 = local write "Actual"(w4297) -> ()
                n1979 = Wait (ms)(milliseconds to wait=u32 50 ("等待时间（毫秒）")) -> ()  [unwired: 1 out]
              }
            }
            n1980 = VISA Close(VISA resource name=w4282, error in (no error)=w4281) -> (error out=w4277:errorcluster)
          }
          frame True {
            n1981 = VISA Open(error in (no error)=w4306, VISA resource name="VISA resource name 4") -> (VISA resource name=w4304:refnum<visa-resource-name>, error out=w4303:errorcluster)  [unwired: 1 in, 2 out]
            n1982 = property class="Instr"(reference=w4304, error in=w4303, "Timeout"=u32 100 ("General Settings:Timeout Value")) -> (reference out=w4301:refnum<visa-resource-name>, error out=w4302:errorcluster)
            n1983 = call-poly "VISA Configure Serial Port"("VISA resource name"=w4301, "error in (no error)"=w4302) -> ("VISA resource name out"=w4310:refnum<visa-resource-name>, "error out"=w4307:errorcluster)  [unwired: 4 in, 8 out]
            n1984 = Unbundle(w4307) -> ("status"=w4309:bool)  [unwired: 2 out]
            n1985 = case shown="假" w4309 {
              tunnel: w4310 -> [w4314 w4317]
              frame False {
                w4312 = u8 0 ("禁用")
                n1986 = local write "VISA资源名称输出 10"(w4314) -> ()
                n1987 = local write "连接状态 10"(TRUE ("连接状态")) -> ()
                n1988 = property on="输出150V" class="Bool"("Disabled"=w4312) -> ()  [unwired: 2 in, 2 out]
                n1989 = property on="输出300V" class="Bool"("Disabled"=w4312) -> ()  [unwired: 2 in, 2 out]
                n1990 = property on="输出自定义值2" class="Bool"("Disabled"=w4312) -> ()  [unwired: 2 in, 2 out]
                n1991 = property on="输出自定义值1" class="Bool"("Disabled"=w4312) -> ()  [unwired: 2 in, 2 out]
                n1992 = property on="连接状态 10" class="Bool (严格)"("Colors [4]"=cluster{u32, u32}[] [{6618880, 6618880}] ("颜色[4]")) -> ()  [unwired: 2 in, 2 out]
              }
              frame True {
                w4316 = u8 2 ("禁用")
                n1993 = local write "VISA资源名称输出 10"(w4317) -> ()
                n1994 = local write "连接状态 10"(FALSE ("连接状态")) -> ()
                n1995 = property on="输出150V" class="Bool"("Disabled"=w4316) -> ()  [unwired: 2 in, 2 out]
                n1996 = property on="输出300V" class="Bool"("Disabled"=w4316) -> ()  [unwired: 2 in, 2 out]
                n1997 = property on="输出自定义值2" class="Bool"("Disabled"=w4316) -> ()  [unwired: 2 in, 2 out]
                n1998 = property on="输出自定义值1" class="Bool"("Disabled"=w4316) -> ()  [unwired: 2 in, 2 out]
                n1999 = property on="连接状态 10" class="Bool (严格)"("Colors [4]"=cluster{u32, u32}[] [{15663131, 6618880}] ("颜色[4]")) -> ()  [unwired: 2 in, 2 out]
              }
            }
          }
        }
      }
      event "Set_out": Value Change {
        n2000 = event-data() -> ("NewVal"=w4323:bool)  [unwired: 6 out]
        n2001 = case shown="真" w4323 {
          tunnel: w4322 -> [w4325 w4335]
          tunnel: w4321 -> [w4324 w4334]
          tunnel: [w4324 w4333] -> w4320
          tunnel: [w4325 w4332] -> w4319
          frame False {
          }
          frame True {
            n2002 = flat-sequence {
              tunnel: w4334 -> [w4342]
              tunnel: w4335 -> [w4343]
              tunnel: [w4343] -> w4331
              tunnel: [w4342] -> w4330
              tunnel: [w4346] -> w4333
              tunnel: [w4345] -> w4332
              tunnel: w4331 -> [w4348]
              tunnel: w4330 -> [w4347]
              frame #0 {
                n2003 = local read "REAL2"() -> (w4340:dbl)
                n2004 = local read "REAL1"() -> (w4341:dbl)
                n2005 = local read "AD1"() -> (w4339:dbl)
                n2006 = local read "AD2"() -> (w4338:dbl)
                n2007 = call "Cal_Gain&offset.vi"("REAL2"=w4340, "REAL1"=w4341, "AD2"=w4338, "AD1"=w4339) -> ("Offset"=w4337:i32, "Gain"=w4336:dbl)  [unwired: 5 out]
                n2008 = local write "Offset"(w4337) -> ()
                n2009 = local write "Gain"(w4336) -> ()
              }
              frame #1 {
                n2010 = Enqueue Element(queue=w4348, element="Set_out" ("元素"), error in (no error)=w4347) -> (queue out=w4345:refnum<queue>, error out=w4346:errorcluster)  [unwired: 2 out]
              }
            }
            n2011 = global write "EV05全局变量1.vi" "CAN接收"(FALSE ("CAN接收")) -> ()
            n2012 = global write "EV05全局变量1.vi" "高压校正接收"(FALSE ("高压校正接收")) -> ()
            n2013 = call <vilib>:"Set Busy.vi"() -> ()  [unwired: 4 in, 8 out]
            n2014 = property on="Set_out结果" class="Bool (严格)"("Colors [4]"=cluster{u32, u32}[] [{0, 0}] ("颜色[4]"), "BoolText.Text"="" ("布尔文本.文本")) -> ()  [unwired: 2 in, 2 out]
          }
        }
      }
    }
  }
  n2015 = while {
    tunnel: "error in (no error)" -> [w4356]
    tunnel: [w4349] -> _
    stop <- "停止 7" stop-if-true
    n2016 = local read "连接状态 10"() -> (w4357:bool)
    n2017 = local read "控制读取  2"() -> (w4358:bool)
    n2018 = Tick Count (ms)() -> (millisecond timer value=w4354:u32)
    n2019 = And(x=w4357, y=w4358) -> (x .and. y?=w4350:bool)
    n2020 = case shown="真" w4350 {
      tunnel: w4356 -> [_ w4372]
      tunnel: [_ w4364] -> w4355
      tunnel: w4354 -> [w4361 w4366]
      tunnel: [w4361 w4366] -> w4353
      tunnel: [w4362 w4363] -> w4352
      frame False {
        n2021 = Tick Count (ms)() -> (millisecond timer value=w4362:u32)
      }
      frame True {
        n2022 = local read "VISA资源名称输出"() -> (w4376:refnum<visa-resource-name>)
        n2023 = VISA Write(VISA resource name=w4376, write buffer="MEAS:curr?" ("写入缓冲区"), error in (no error)=w4372) -> (VISA resource name out=w4371:refnum<visa-resource-name>, error out=w4370:errorcluster)  [unwired: 1 out]
        n2024 = flat-sequence {
          tunnel: w4371 -> [w4381]
          tunnel: w4370 -> [w4380]
          tunnel: [w4381] -> w4369
          tunnel: [w4380] -> w4368
          frame #0 {
            n2025 = Wait (ms)(milliseconds to wait=u32 50 ("等待时间（毫秒）")) -> ()  [unwired: 1 out]
          }
        }
        n2026 = VISA Read(VISA resource name=w4369, byte count=u32 20 ("字节总数"), error in (no error)=w4368) -> (read buffer=w4374:string, error out=w4365:errorcluster)  [unwired: 2 out]
        n2027 = Fract/Exp String To Number(string=w4374) -> (number=w4373:dbl)  [unwired: 4 out]
        n2028 = local write "Actual"(w4373) -> ()
        n2029 = flat-sequence {
          tunnel: w4365 -> [w4378]
          tunnel: [w4378] -> w4364
          tunnel: [w4377] -> w4363
          frame #0 {
            n2030 = Tick Count (ms)() -> (millisecond timer value=w4377:u32)
          }
        }
      }
    }
    n2031 = Wait (ms)(milliseconds to wait=u32 50 ("等待时间（毫秒）")) -> ()  [unwired: 1 out]
    n2032 = Subtract(x=w4352, y=w4353) -> (x-y=→"x-y":u32)
    n2033 = call <vilib>:"Clear Errors.vi"("error in (no error)"=w4355) -> ("error out"=w4349:errorcluster)  [unwired: 6 out]
  }
  n2034 = while {
    tunnel: w8 -> [w4392]
    tunnel: w42 -> [w4391]
    tunnel: [w4384] -> w4
    tunnel: [w4383] -> w5
    stop <- w4394 stop-if-true
    n2035 = local read "CAN路数"() -> (w4385:u16)
    n2036 = local read "CAN卡类型"() -> (w4387:u32)
    n2037 = local read "设备索引"() -> (w4386:u16)
    n2038 = local read "停止 2"() -> (w4394:bool)
    n2039 = call "receiver-8.6.vi"("CAN端口"=w4385, "设备索引号"=w4386, "CAN卡类型"=w4387) -> ("输出簇"=w4382:T14, "接收成功"=w4393:bool)  [unwired: 1 in, 4 out]
    n2040 = case shown="真" w4393 {
      tunnel: w4392 -> [w4405 w4410]
      tunnel: w4391 -> [w4404 w4409]
      tunnel: w4382 -> [_ w4408]
      tunnel: [w4405 w4407] -> w4389
      tunnel: [w4404 w4406] -> w4388
      frame False {
      }
      frame True {
        n2041 = Enqueue Element(queue=w4410, element=w4408, error in (no error)=w4409) -> (queue out=w4407:refnum<queue>, error out=w4406:errorcluster)  [unwired: 1 in, 1 out]
      }
    }
    n2042 = call "已用时间"() -> ("Elapsed Time (s)"=w4390:dbl)  [unwired: 12 in, 7 out]
    n2043 = case shown="0, 默认" w4390 {
      tunnel: w4389 -> [w4395 w4398]
      tunnel: w4388 -> [w4396 w4400]
      tunnel: w4387 -> [_ w4403]
      tunnel: w4386 -> [_ w4402]
      tunnel: w4385 -> [_ w4401]
      tunnel: [w4396 w4399] -> w4384
      tunnel: [w4395 w4397] -> w4383
      frame 0, Default {
      }
      frame 1 {
        n2044 = dll-call lib="PTH1aabs FBluewave New Energy\t上位机BMS_Monitor - 91版 新源data\nkerneldlls\nusbcan.dll" fn="VCI_ClearBuffer"(error in=w4400, "DeviceType"=w4403, "DeviceInd"=w4402, "CANInd"=w4401) -> (error out=w4399:errorcluster)  [unwired: 3 in, 4 out]
        n2045 = Flush Queue(queue=w4398) -> (queue out=w4397:refnum<queue>)  [unwired: 1 in, 2 out]
      }
    }
  }
  n2046 = global read "功能码全局.vi" "13"() -> (w18:bool[])
  n2047 = Index Array(array=w18) -> (element #5=w9:bool, element #6=w10:bool, element #7=w11:bool, element #8=w12:bool)  [unwired: 8 in, 4 out]
  n2048 = Not(x=w9) -> (.not. x?=w17:bool)
  n2049 = Not(x=w10) -> (.not. x?=w14:bool)
  n2050 = Compound Arithmetic op=AND(w12, w11, w10, w9) -> (w13:bool)
  n2051 = property on="电流校正 2" class="TabCtl (严格)"("Visible"=w17) -> ()  [unwired: 2 in, 2 out]
  n2052 = property on="电流校正" class="TabCtl (严格)"("Visible"=w17) -> ()  [unwired: 2 in, 2 out]
  n2053 = Not(x=w11) -> (.not. x?=w15:bool)
  n2054 = Not(x=w12) -> (.not. x?=w16:bool)
  n2055 = property on="一键校正" class="Bool (严格)"("Visible"=w13) -> ()  [unwired: 2 in, 2 out]
  n2056 = property on="外总压" class="TabCtl (严格)"("Visible"=w14) -> ()  [unwired: 2 in, 2 out]
  n2057 = property on="内总压" class="TabCtl (严格)"("Visible"=w15) -> ()  [unwired: 2 in, 2 out]
  n2058 = property on="分流器" class="TabCtl (严格)"("Visible"=w16) -> ()  [unwired: 2 in, 2 out]
  n2059 = Release Queue(queue=w5, force destroy? (F)=TRUE ("强制销毁？(F)"), error in (no error)=w4) -> (error out=w7:errorcluster)  [unwired: 2 out]
  n2060 = call <vilib>:"Clear Errors.vi"("error in (no error)"=w7) -> ()  [unwired: 7 out]
  n2061 = control-ref of="结果"() -> (w22:refnum<vi>)
  n2062 = for {
    N: 40 -> [_]
    tunnel: w22 -> [w4415]
    i -> [w4413]
    n2063 = Bundle(w4413, 0) -> (w4411:cluster{i32, i32})  [unwired: 1 out]
    n2064 = property class="MCListbox (严格)"(reference=w4415, "ActiveCell"=w4411, "CellBG"=u32 16448250) -> ()  [unwired: 1 in, 2 out]
  }
  n2065 = property class="MCListbox (严格)"(reference=w22, "ItemNames"=string[][] [] ("项名")) -> ()  [unwired: 1 in, 2 out]
  n2066 = global write "EV05全局变量1.vi" "CAN接收"(TRUE ("CAN接收")) -> ()
  n2067 = local write "监控状态"(FALSE ("监控状态")) -> ()
  n2068 = property on="SumV_out" class="DigNum (严格)"("NumText.BGColor"=w19) -> ()  [unwired: 2 in, 2 out]
  n2069 = property on="SumV_in" class="DigNum (严格)"("NumText.BGColor"=w19) -> ()  [unwired: 2 in, 2 out]
  n2070 = property on="Curr" class="DigNum (严格)"("NumText.BGColor"=w19) -> ()  [unwired: 2 in, 2 out]
  n2071 = call "自适应屏幕分辨率.vi"() -> ()  [unwired: 16 in]
  n2072 = Release Queue(queue=w31, force destroy? (F)=TRUE ("强制销毁？(F)"), error in (no error)=w32) -> (error out=w29:errorcluster)  [unwired: 2 out]
  n2073 = property on="连接状态 10" class="Bool (严格)"("Colors [4]"=w25) -> ()  [unwired: 2 in, 2 out]
  n2074 = property on="连接状态 10" class="Bool (严格)"("Colors [4]"=w25) -> ()  [unwired: 2 in, 2 out]
  n2075 = property on="监控状态" class="Bool (严格)"("Colors [4]"=w25) -> ()  [unwired: 2 in, 2 out]
  n2076 = call <vilib>:"Clear Errors.vi"("error in (no error)"=w29) -> ()  [unwired: 7 out]
  n2077 = property on="Set结果" class="Bool (严格)"("Colors [4]"=w25, "BoolText.Text"=w24) -> ()  [unwired: 2 in, 2 out]
  n2078 = property on="Read1结果" class="Bool (严格)"("Colors [4]"=w25, "BoolText.Text"=w24) -> ()  [unwired: 2 in, 2 out]
  n2079 = local write "行号"(0.0 ("行号")) -> ()
  n2080 = property on="Clear_in结果" class="Bool (严格)"("Colors [4]"=w25, "BoolText.Text"=w24) -> ()  [unwired: 2 in, 2 out]
  n2081 = property on="Current Offset结果 2" class="Bool (严格)"("Colors [4]"=w25, "BoolText.Text"=w24) -> ()  [unwired: 2 in, 2 out]
  n2082 = property on="Current Offset结果 4" class="Bool (严格)"("Colors [4]"=w25, "BoolText.Text"=w24) -> ()  [unwired: 2 in, 2 out]
  n2083 = property on="Current Gain结果 4" class="Bool (严格)"("Colors [4]"=w25, "BoolText.Text"=w24) -> ()  [unwired: 2 in, 2 out]
  n2084 = property on="Set_out结果" class="Bool (严格)"("Colors [4]"=w25, "BoolText.Text"=w24) -> ()  [unwired: 2 in, 2 out]
  n2085 = local write "停止"(w36) -> ()
  n2086 = property on="Read2_Out结果" class="Bool (严格)"("Colors [4]"=w25, "BoolText.Text"=w24) -> ()  [unwired: 2 in, 2 out]
  n2087 = property on="Read1_Out结果" class="Bool (严格)"("Colors [4]"=w25, "BoolText.Text"=w24) -> ()  [unwired: 2 in, 2 out]
  n2088 = property on="Current Offset结果" class="Bool (严格)"("Colors [4]"=w25, "BoolText.Text"=w24) -> ()  [unwired: 2 in, 2 out]
  n2089 = property on="Current Offset结果 3" class="Bool (严格)"("Colors [4]"=w25, "BoolText.Text"=w24) -> ()  [unwired: 2 in, 2 out]
  n2090 = property on="Current Gain结果 3" class="Bool (严格)"("Colors [4]"=w25, "BoolText.Text"=w24) -> ()  [unwired: 2 in, 2 out]
  n2091 = local write "停止 3"(w36) -> ()
  n2092 = local write "停止 2"(w36) -> ()
  n2093 = local write "停止 6"(w36) -> ()
  n2094 = local write "停止 7"(w36) -> ()
  n2095 = property on="Read2结果" class="Bool (严格)"("Colors [4]"=w25, "BoolText.Text"=w24) -> ()  [unwired: 2 in, 2 out]
  n2096 = property on="Current Offset结果" class="Bool (严格)"("Colors [4]"=w25, "BoolText.Text"=w24) -> ()  [unwired: 2 in, 2 out]
  n2097 = property on="Current Gain结果" class="Bool (严格)"("Colors [4]"=w25, "BoolText.Text"=w24) -> ()  [unwired: 2 in, 2 out]
  n2098 = property on="Clear结果" class="Bool (严格)"("Colors [4]"=w25, "BoolText.Text"=w24) -> ()  [unwired: 2 in, 2 out]
  n2099 = property on="Read1_in结果" class="Bool (严格)"("Colors [4]"=w25, "BoolText.Text"=w24) -> ()  [unwired: 2 in, 2 out]
  n2100 = property on="Clear_out结果" class="Bool (严格)"("Colors [4]"=w25, "BoolText.Text"=w24) -> ()  [unwired: 2 in, 2 out]
  n2101 = property on="Read2_in结果" class="Bool (严格)"("Colors [4]"=w25, "BoolText.Text"=w24) -> ()  [unwired: 2 in, 2 out]
  n2102 = property on="Set_in结果" class="Bool (严格)"("Colors [4]"=w25, "BoolText.Text"=w24) -> ()  [unwired: 2 in, 2 out]
  n2103 = property on="Current Gain结果 2" class="Bool (严格)"("Colors [4]"=w25, "BoolText.Text"=w24) -> ()  [unwired: 2 in, 2 out]
  "CAN连接状态" <- FALSE ("CAN连接状态")
  "CAN" <- FALSE ("CAN接收")
  "测试结果" <- TRUE ("测试结果")
  "Set" <- 0.0 ("电压/V")
  "Actual" <- 0.0 ("电流/A")
  "电流/A 4" <- 0.0 ("电流/A")
  "设定值 2" <- 0.0 ("电压/V")
  "实际值 2" <- w47
